vi "MICS Wakeup Calibration Tool JTAG.vi"(8 "error in (no error)":errorcluster, 10 "MICS Dongle Address":refnum<visa-resource-name>="COM8") -> (0 "error out":errorcluster, 2 "Trim Settings":string)   [LabVIEW 2010]
uses:
  <vilib>/Instr/_visa.llb/VISA Configure Serial Port (Instr).vi
panel:
  in  "RSSI Gain":enum16{"1", "3", "10", "30"}(ring)
  in  "WakeupRF":bool
  out "RSSI":u8 format="%02x"
  out "Device Vcc":i32
  in  "DetTrim":bool=TRUE
  in  "Wakeup Signal Transmit":bool
  in  "Samples to Average":u8=5 format="%02d"
  out "Retries":u8 format="%02d"
  out "Loopback Data":u8 format="%02x"
  in  "Loopback Detector":bool
  in  "Update Radio Settings":bool
  in  "Done":bool
  in  "Do RSSI":bool
  out "RSSI Reading":u8(knob) scale=0.0..31.0 scale format="%x"
  in  "Detector Offset Trim":u8(knob)=31 scale=0.0..63.0 scale format="%x"
  in  "Wakeup Signal Power, dBm":dbl(knob)=-32.0 min=-32.25 max=0.0 step=0.25
  in  "RSSI Fine Trim":u8(knob)=16 scale=0.0..31.0 scale format="%x"
  in  "RX Antenna Tune":u8(knob)=7 scale=0.0..15.0 scale format="%x"
  in  "LNA Frequency Trim":u8(knob)=15 scale=0.0..31.0 scale format="%x"
  in  "LNA Gain Trim":u8(knob)=20 scale=0.0..63.0 scale format="%x"
  # "MICS Dongle Address"
  # "All Trims"
  # "Detector Trims Only"
  # "CW RF"
  # "Wakeup Packet"
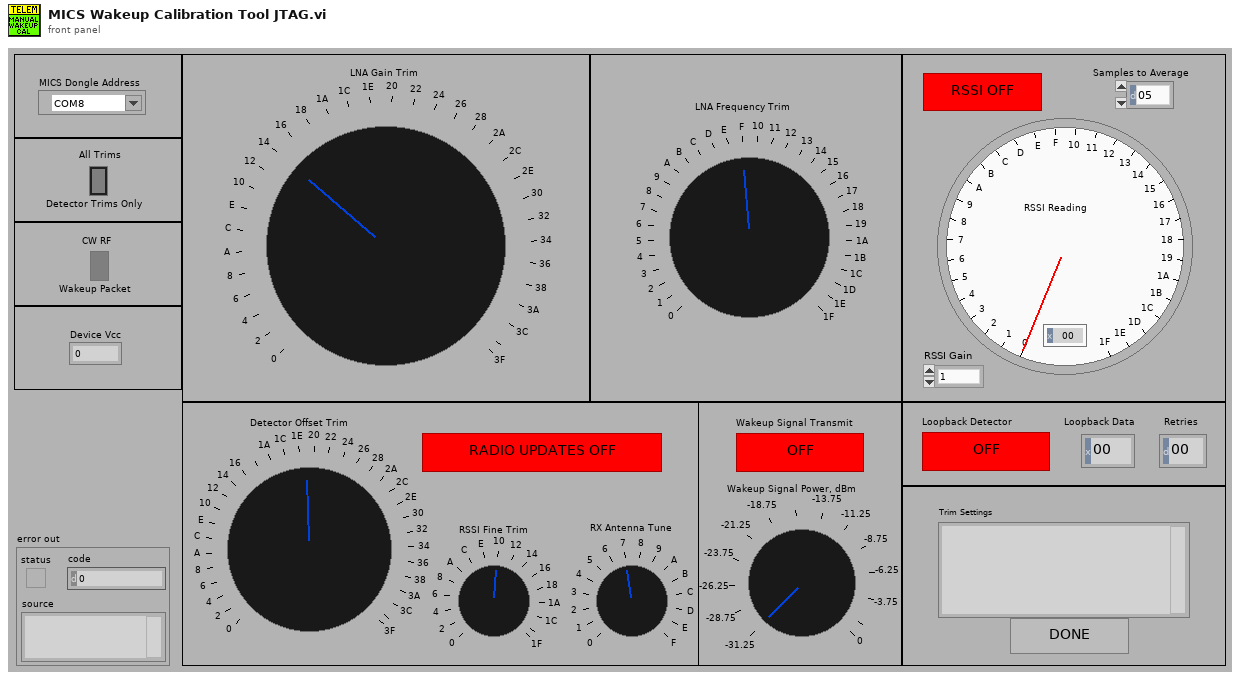
[diagram p1: front panel]
types:
  T1 = cluster{"ConfigFlags":u8, "ImplantID":u32, "CompanyID":u8, "Normal_Comm":cluster{"RF_Channel":u8, "UserData":u8, "TX_Mod":u8, "RX_Mod":u8, "RX_BlockSize":u8, "BlockPerPack":u8, "TX_BlockSize":u8}, "Emerg_Comm":cluster{"RF_Channel":u8, "UserData":u8, "TX_Mod":u8, "RX_Mod":u8, "TX_BlockSize":u8, "BlockPerPack":u8, "RX_BlockSize":u8}, "ImplantRev":u8, "245TX_PowerCal":i8, "245TX_Power":i8, "CCA_RSSI_Thresholds":cluster{"ch0":u16, "ch1":u16, "ch2":u16, "ch3":u16, "ch4":u16, "ch5":u16, "ch6":u16, "ch7":u16, "ch8":u16, "ch9":u16}}
  T2 = enum16{"Start Search", "Continue Search", "End Search"}
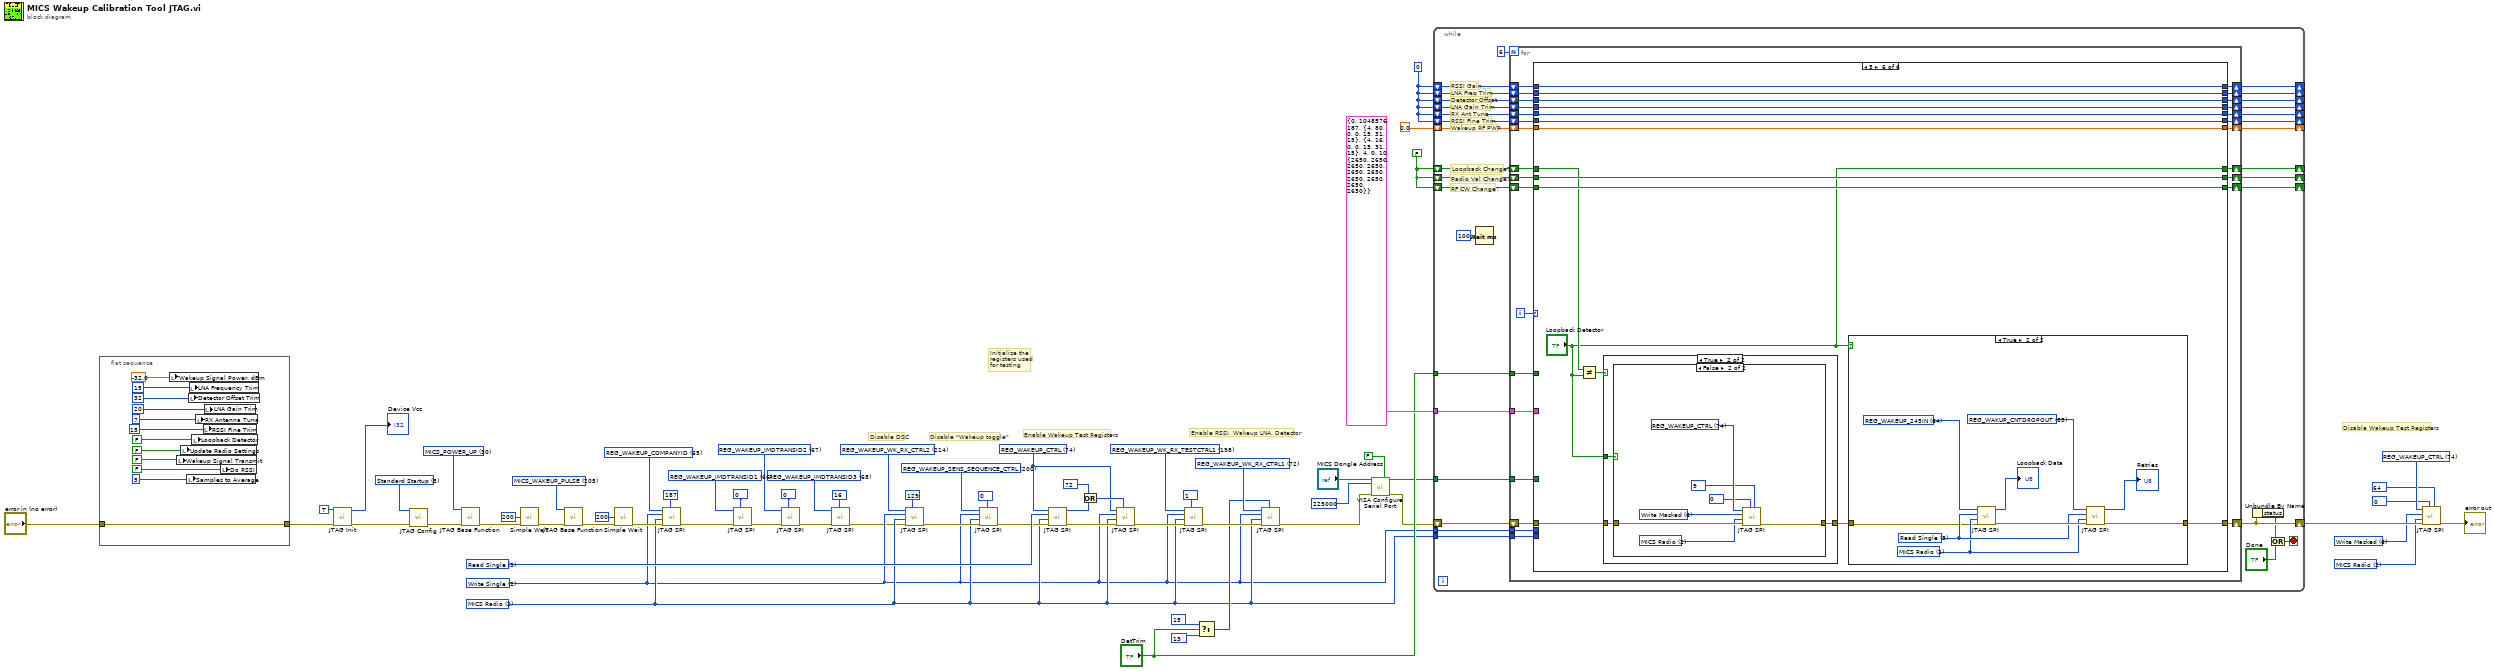
[diagram p0: block diagram]
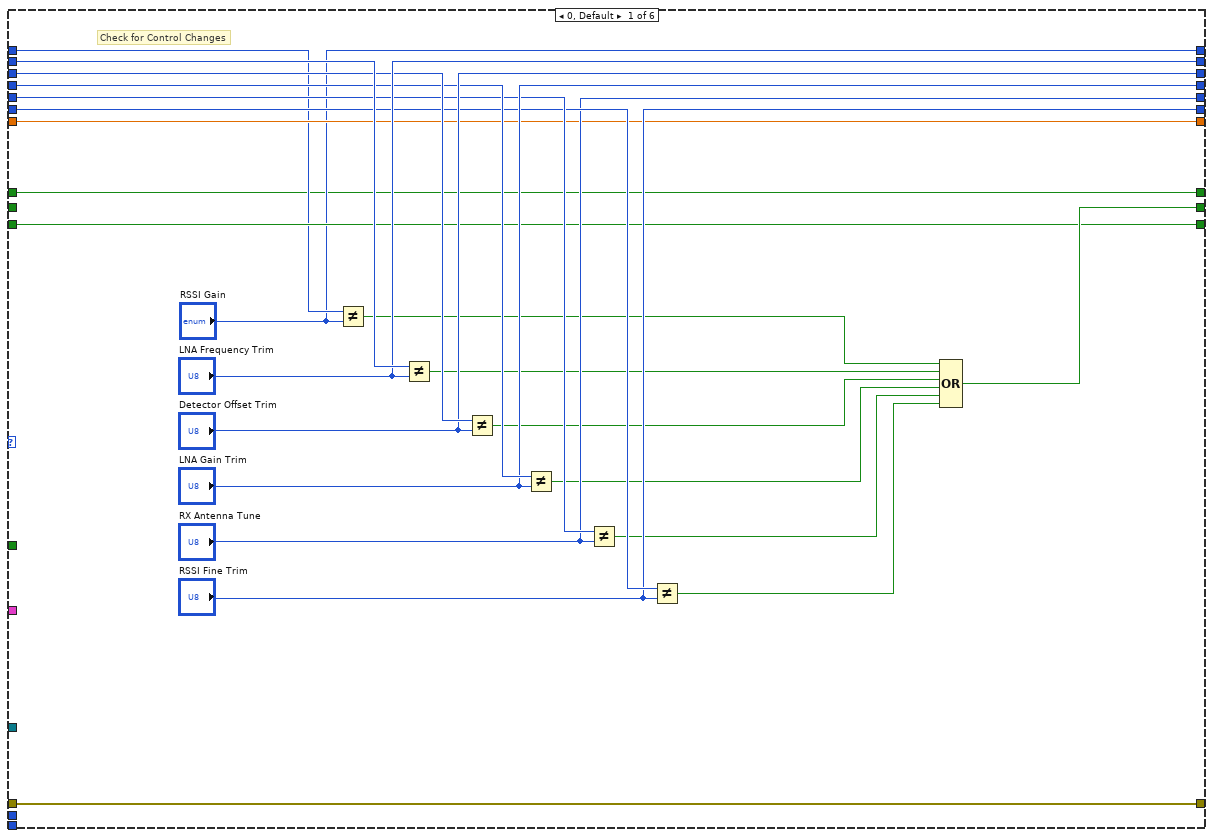
[diagram p2: hidden frame]
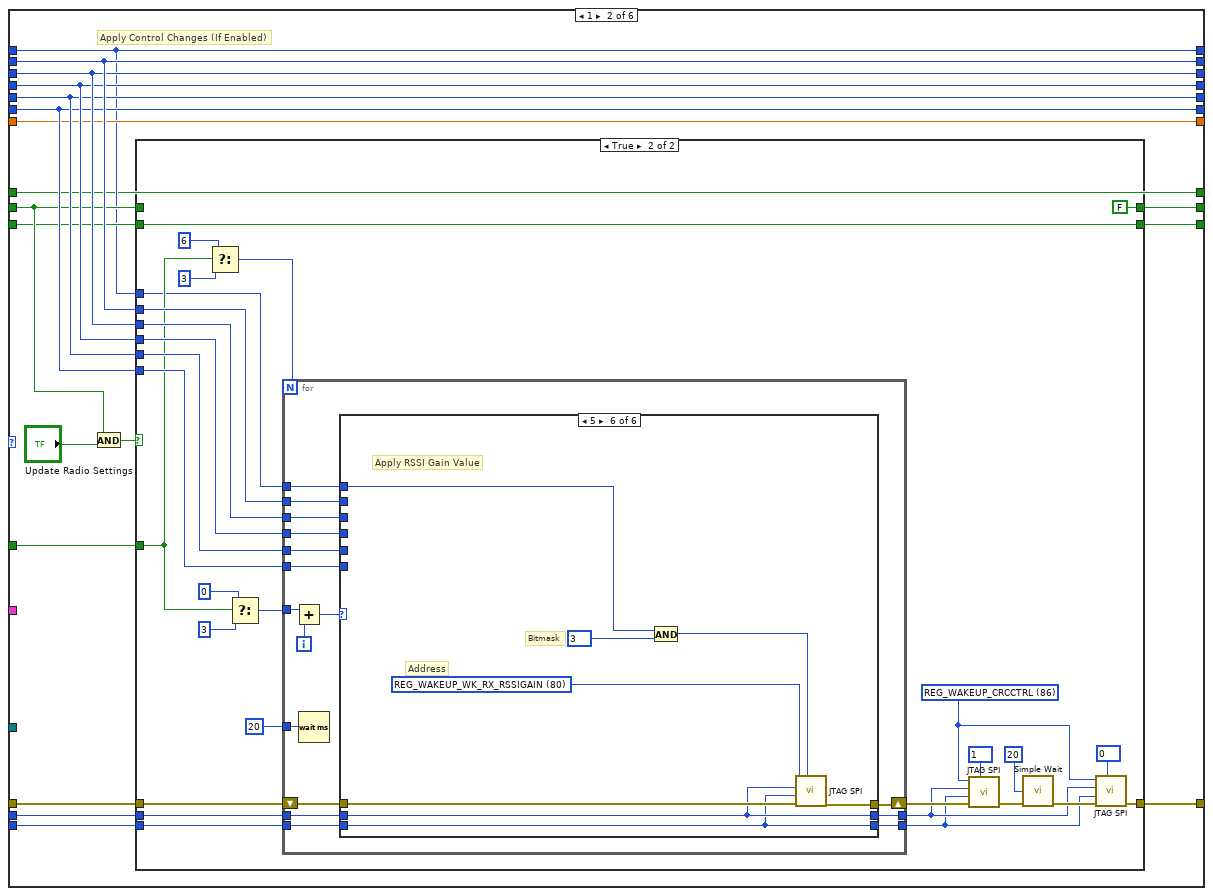
[diagram p3: hidden frame]
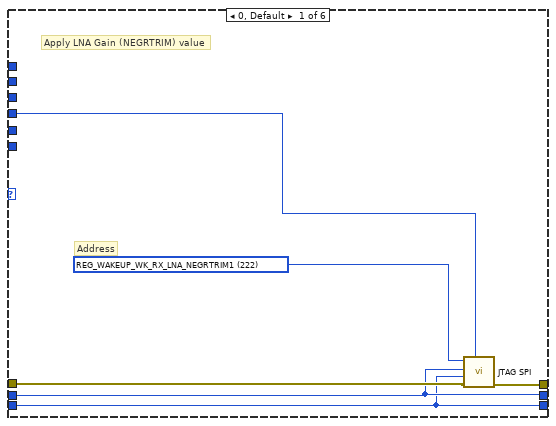
[diagram p5: hidden frame]
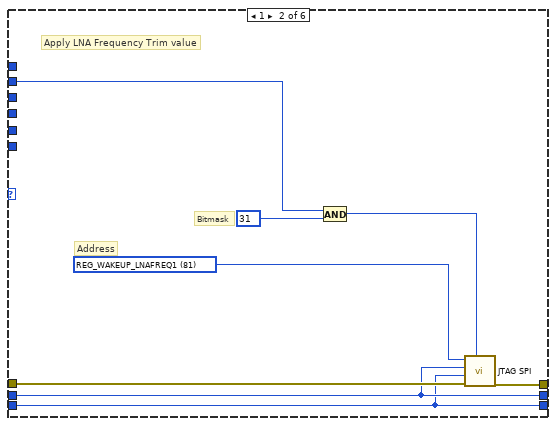
[diagram p6: hidden frame]
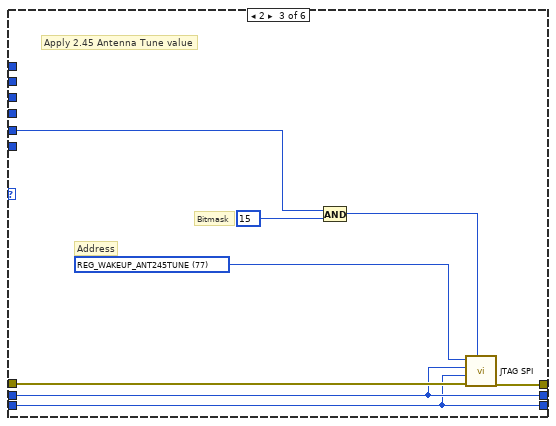
[diagram p7: hidden frame]
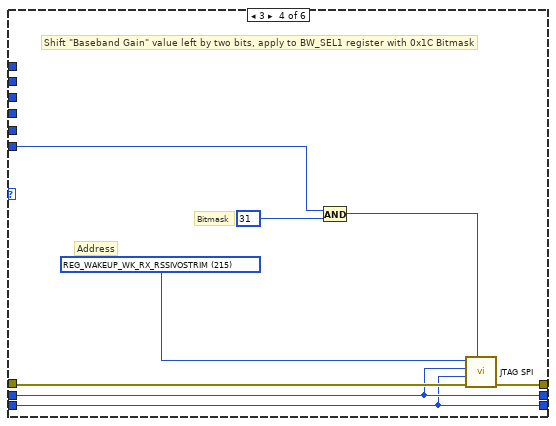
[diagram p8: hidden frame]
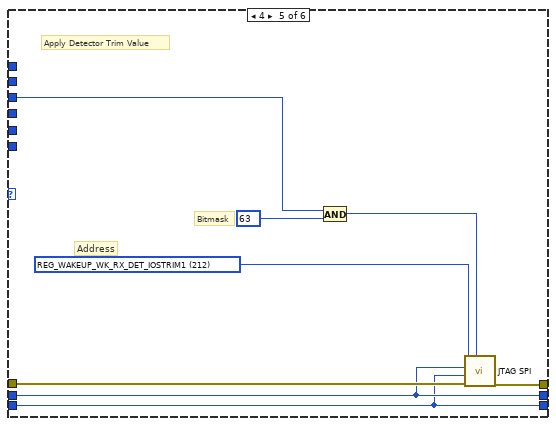
[diagram p9: hidden frame]
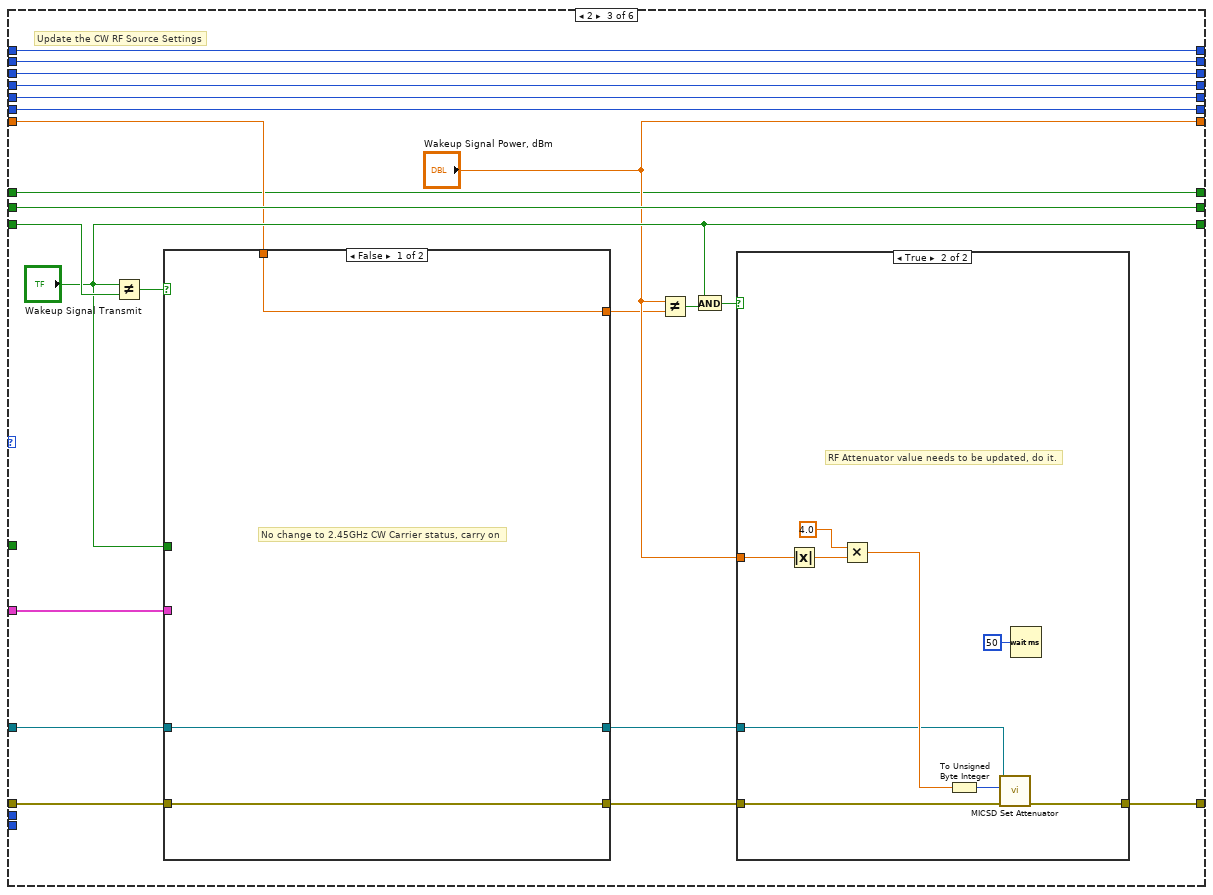
[diagram p10: hidden frame]
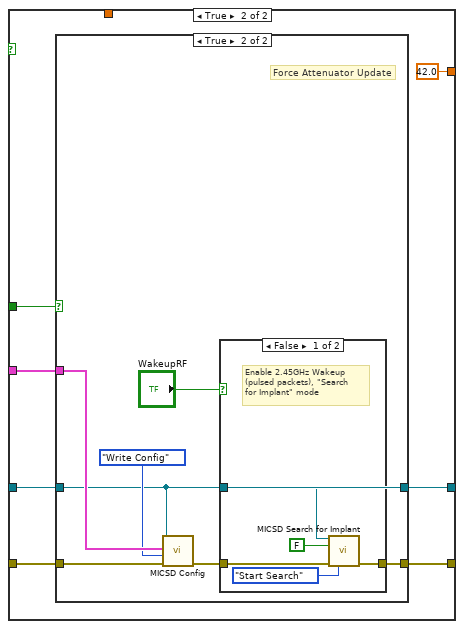
[diagram p12: hidden frame]
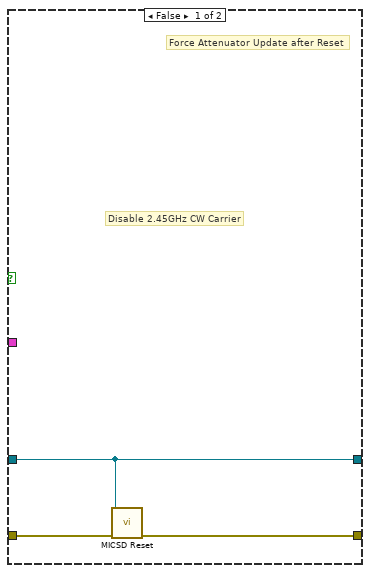
[diagram p13: hidden frame]
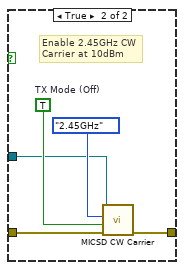
[diagram p14: hidden frame]
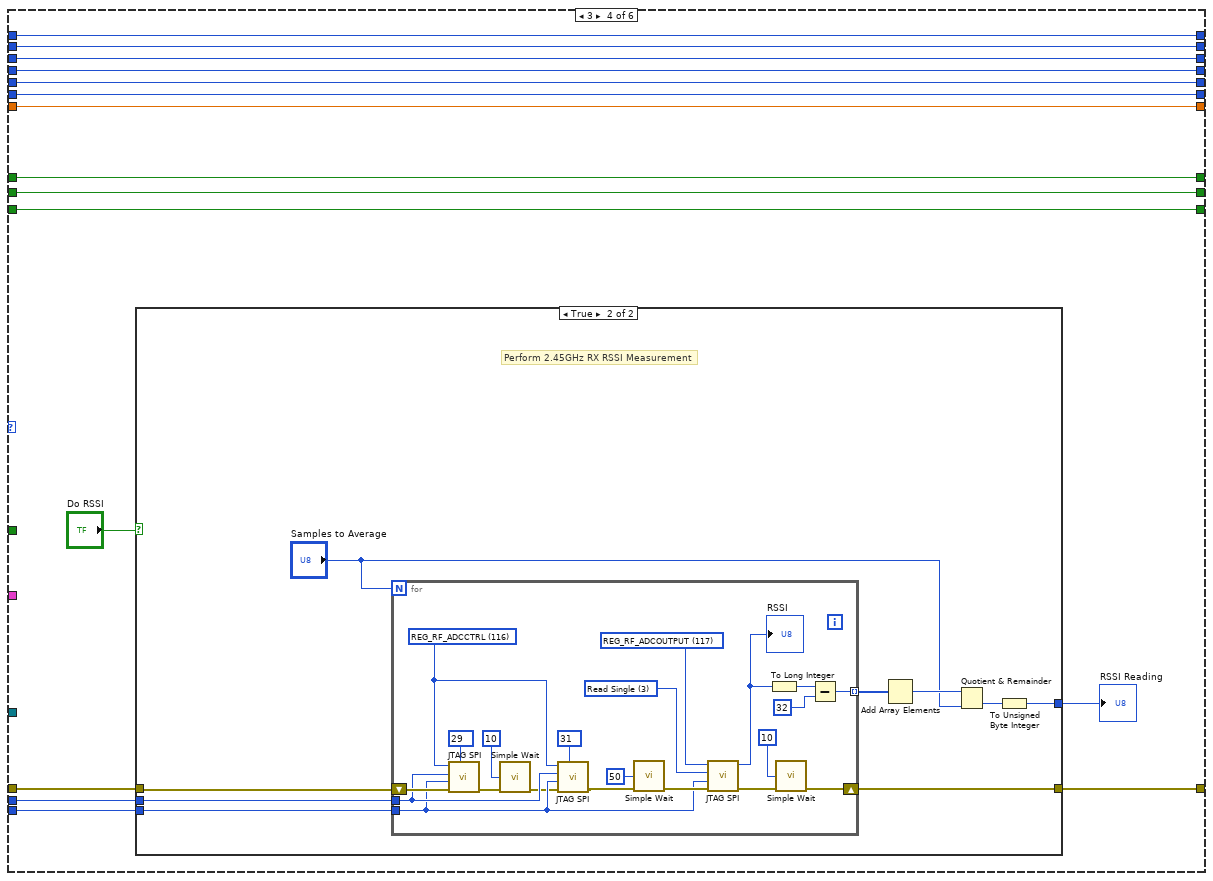
[diagram p15: hidden frame]
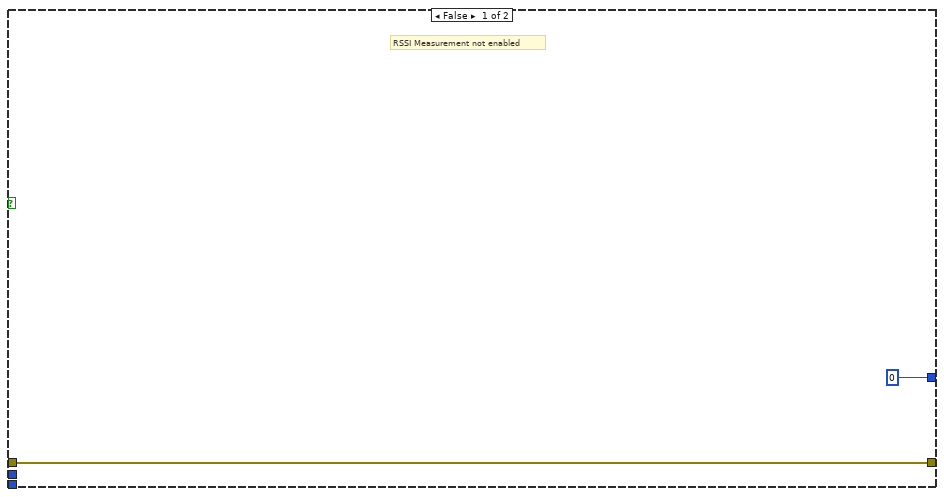
[diagram p16: hidden frame]
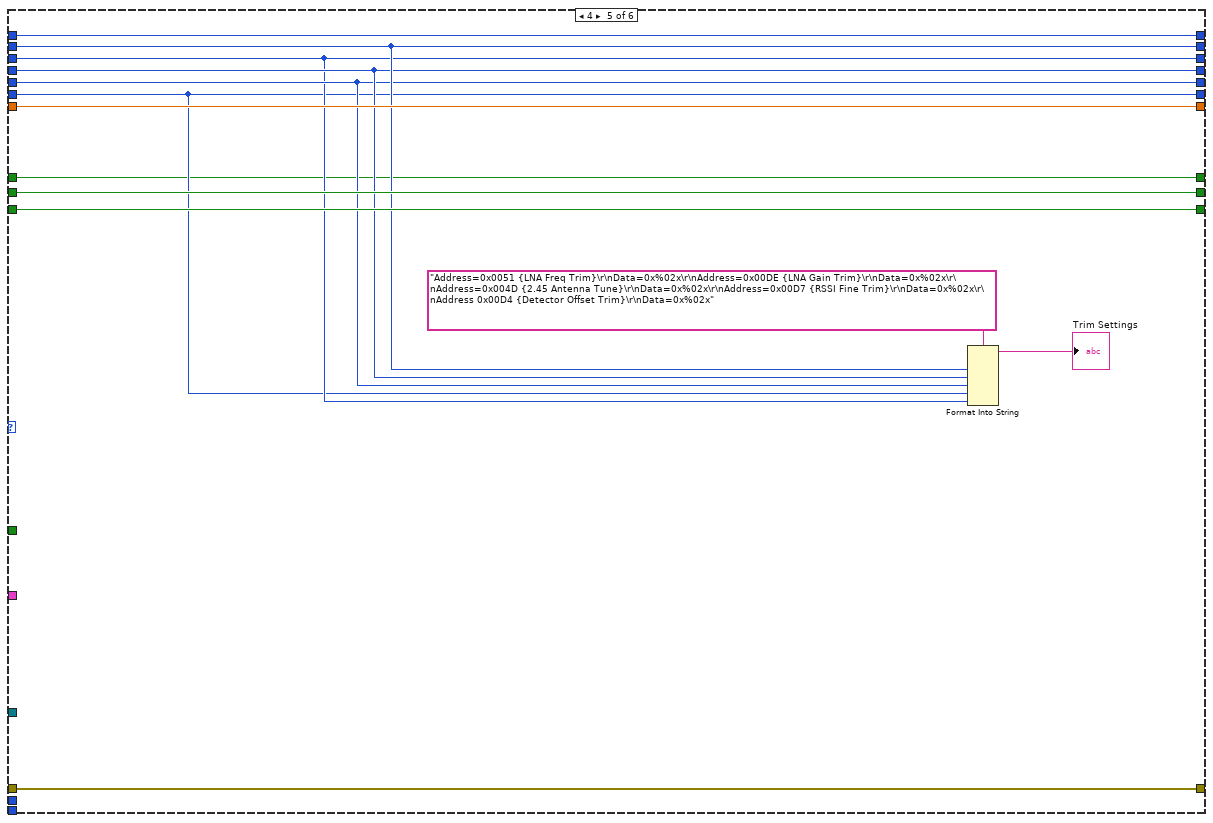
[diagram p17: hidden frame]
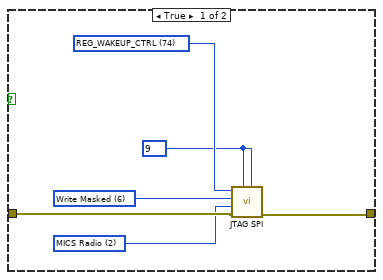
[diagram p19: hidden frame]
diagram:
  w12 = u16 68 items=["---MANUAL ENTRY---"=1000, "REG_NOREG"=0, "REG_RXBUFF_USED"=1, "REG_RXBUFF_BSIZE"=2, "REG_TXBUFF_USED"=3, "REG_TXBUFF_BSIZE"=4, "REG_TXBUFF_MAXPACKSIZE"=5, "REG_MAC_ERRCLR"=6, "REG_MAC_TRAINNUM"=7, "REG_MAC_SYNCMATCH"=8, "REG_MAC_SYNC1"=9, "REG_MAC_SYNC2"=10, "REG_MAC_SYNC3"=11, "REG_MAC_SYNC4"=12, "REG_MAC_SYNC5"=13, "REG_MAC_MAXBERR"=14, "REG_MAC_ECCORR"=15, "REG_MAC_CRCERR"=16, "REG_MAC_BLKCNT1"=17, "REG_MAC_BLKCNT2"=18, "REG_MAC_IMDTRANSID1"=19, "REG_MAC_IMDTRANSID2"=20, "REG_MAC_IMDTRANSID3"=21, "REG_MAC_COMPANYID"=22, "REG_MAC_MODUSER"=23, "REG_MAC_CHANNEL"=25, "REG_MAC_CLEARWDOG"=26, "REG_MAC_CKCORRTHRESH"=27, "REG_HK_TXADDR"=28, "REG_HK_TXDATA"=29, "REG_HK_TXREPLY"=30, "REG_HK_USERDATA"=31, "REG_HK_USERSTATUS"=32, "REG_HK_LASTADDRESS"=33, "REG_HK_MODE"=34, "REG_MAC_STATUSSEQ"=35, "REG_MAC_MAXRETRIES"=36, "REG_MAC_RESENDTIME"=37, "REG_MAC_POWERSAVETIME"=38, "REG_MAC_HEAD_DET"=39, "REG_MAC_CTRL"=41, "REG_MAC_INITCOM"=42, "REG_INTERFACE_MODE"=43, "REG_TXRXBUFF_BOTH"=44, "REG_TXRXBUFF"=45, "REG_IRQ_RAWSTATUS1"=46, "REG_IRQ_ENABLE1"=47, "REG_IRQ_ENABLESET1"=48, "REG_IRQ_ENABLECLEAR1"=49, "REG_IRQ_RAWSTATUS2"=50, "REG_IRQ_ENABLE2"=51, "REG_IRQ_ENABLESET2"=52, "REG_IRQ_ENABLECLEAR2"=53, "REG_IRQ_STATUS1"=54, "REG_IRQ_STATUS2"=55, "REG_IRQ_AUXSTATUS"=56, "REG_TXBUFF_OVERFLOW"=57, "REG_PO0"=58, "REG_P01"=59, "REG_P02"=60, "REG_P03"=61, "REG_GP0"=62, "REG_GPI"=63, "REG_WAKEUP_245IN"=64, "REG_WAKEUP_COMPANYID"=65, "REG_WAKEUP_IMDTRANSID1"=66, "REG_WAKEUP_IMDTRANSID2"=67, "REG_WAKEUP_IMDTRANSID3"=68, "REG_WAKEUP_CHANNEL"=69, "REG_WAKEUP_MODUSER"=70, "REG_WAKEUP_DEVICEMODE"=71, "REG_WAKEUP_WK_RX_CTRL1"=72, "REG_WAKEUP_STACK_ADDR"=73, "REG_WAKEUP_CTRL"=74, "REG_WAKEUP_STROSCRTRIM"=75, "REG_WAKEUP_BIASTRIM"=76, "REG_WAKEUP_ANT245TUNE"=77, "REG_WAKEUP_WK_RX_RTRIMDET"=78, "REG_WAKEUP_WK_RX_RTRIMDEMOD"=79, "REG_WAKEUP_WK_RX_RSSIGAIN"=80, "REG_WAKEUP_LNAFREQ1"=81, "REG_WAKEUP_STACK"=83, "REG_WAKUP_XOSU"=84, "REG_WAKUP_CNTDROPOUT"=85, "REG_WAKEUP_CRCCTRL"=86, "REG_WAKEUP_CRCWORD1"=87, "REG_WAKEUP_CRCWORD2"=88, "REG_WAKEUP_WK_RX_CTRIM"=89, "REG_WAKEUP_VDDATRIM"=90, "REG_WAKEUP_VDDDTRIM"=91, "REG_WAKEUP_TESTIOBUFEN"=92, "REG_WAKEUP_TESTIOCLAMP"=93, "CORE_RESET_ADDRESS"=94, "CHIP_RESET_ADDRESS"=95, "REG_RF_TXGENCTRL"=96, "REG_RF_TXIFCTRL"=97, "REG_RF_TXRF_SEL_CTRL"=98, "REG_RF_TXRFPWRDEFAULTSET"=99, "REG_RF_RSSITRIM"=100, "REG_RF_TXIFOSCTUNE"=101, "REG_RF_TXIFGAINIMB"=102, "REG_RF_TXIFLOCK"=103, "REG_RF_RXRFLNAGAINTRIM"=104, "REG_RF_RXBIASTR"=105, "REG_RF_RXGENCTRL"=106, "REG_RF_RXIFADCDECLEV"=107, "REG_RF_RXIFDETFILTERTUNE"=108, "REG_RF_RXIFFILTERTUNE"=109, "REG_RF_GENENABLES"=110, "REG_RF_SYNTH_CHANNEL"=111, "REG_TX_RAMP_RTRIM"=112, "REG_TX_RAMP_CTRIM"=113, "REG_RF_XO_TRIM"=114, "REG_RF_SYNTH_SET_TRIM"=115, "REG_RF_ADCCTRL"=116, "REG_RF_ADCOUTPUT"=117, "REG_RF_TXIFAMP"=118, "REG_RF_SYNTH_RTRIM"=119, "REG_RF_SYNTH_CTRIM"=120, "REG_RF_SYNTH_CT"=121, "REG_RF_TXMIXER_IOSTRIM_HIGH_IP"=122, "REG_RF_TXMIXER_IOSTRIM_HIGH_IN"=123, "REG_RF_TXMIXER_IOSTRIM_HIGH_QP"=124, "REG_RF_TXMIXER_IOSTRIM_HIGH_QN"=125, "REG_HX_WUADDR"=126, "REG_REVISION"=127, "REG_NOREG_TEST"=128, "REG_DTEST_RXBUFF"=129, "REG_RXBUFF_NEXT_BLOCK"=130, "REG_RXBUFF_FIRST_IN_PACK"=131, "REG_RXBUFF_FIRST_EMPTY"=132, "REG_MAC_BYPASS"=133, "REG_DTEST_TXBUFF"=134, "REG_TXBUFF_NEXT_BLOCK"=135, "REG_TXBUFF_FIRST_IN_PACK"=136, "REG_TXBUFF_FIRST_EMPTY"=137, "REG_DTEST_SEQ"=138, "REG_DTEST_CKCORR"=139, "REG_MAC_TOPSTATE"=140, "REG_DTEST_INTERFACE"=141, "REG_IFACE_TXRX_BYPASS"=142, "REG_MAC_TXRXWAIT"=143, "REG_MAC_TXRFRAMP"=144, "REG_MAC_TRAINWORD"=145, "REG_MAC_TRAINWORD2"=146, "REG_MAC_SETTINGS"=147, "REG_MAC_CALSELECT1"=148, "REG_MAC_CALSELECT2"=149, "REG_MAC_ANTMATCHSEL"=150, "REG_MAC_ANTTUNESEL1"=151, "REG_MAC_ANTTUNESEL2"=152, "REG_MAC_ANTTUNESEL3"=153, "REG_MAC_ANTTUNESTEP"=154, "REG_MAC_WUMODEBURST"=156, "REG_MAC_WUOFFSHORT"=157, "REG_MAC_WUOFFLONG"=158, "REG_MAC_CLKRECCTRL"=159, "REG_HK_MODE_P2"=162, "REG_MAC_ANTTUNERES1"=164, "REG_MAC_ANTTUNERES2"=165, "REG_INTERFACE_MODE_TEST"=171, "REG_TXRXBUFF_BOTH_P2"=172, "REG_TXRXBUFF_P2"=173, "REG_IRQ_RAWSTATUS1_P2"=174, "REG_MAC_TXIFSTATUS1"=176, "REG_MAC_TXIFSTATUS2"=177, "REG_IRQ_RAWSTATUS2_P2"=178, "REG_MAC_TXIFRAMPDELAY"=179, "REG_MAC_TXIFRAMPSLOPE"=180, "REG_MAX_TXIFRAMP"=181, "REG_IRQ_STATUS1_P2"=182, "REG_IRQ_STATUS2_P2"=183, "REG_IRQ_AUXSTATUS_P2"=184, "REG_MAC_UNLOCK"=188, "REG_MAC_TXIFFREQ"=190, "REG_WAKEUP_TESTCTRL1"=192, "REG_WAKEUP_RX_EN_CNT"=193, "REG_WAKEUP_TESTENABLES"=194, "REG_WAKEUP_DTBI_CTRL"=195, "REG_WAKEUP_DTBO_CTRL"=196, "REG_WAKEUP_TESTIOBUFTEST"=197, "REG_WAKEUP_WK_RX_TESTCTRL1"=198, "REG_WAKEUP_WK_RX_TESTCTRL2"=199, "REG_WAKEUP_SENS_SEQUENCE_CTRL"=200, "REG_WAKEUP_LNABIAS"=201, "REG_WAKEUP_DET_TH_TRIM1"=202, "REG_WAKEUP_LNABIAS_NOM1"=203, "REG_WAKEUP_RX_TSHORT_TRIM1"=204, "REG_WAKEUP_LNABIAS_NOM2"=205, "REG_WAKEUP_RX_TLONG_TRIM1"=206, "REG_WAKEUP_LNA_NEGRTRIM_NOM1"=207, "REG_WAKEUP_RX_TBURST_TRIM1"=208, "REG_WAKEUP_RX_LNA_NEGRTRIM_NOM2"=209, "REG_WAKEUP_RX_BB_G_BW_SEL1"=210, "REG_WAKEUP_WK_RX_DET_IOSTRIM1"=212, "REG_WAKEUP_WK_RX_CTRL2"=214, "REG_WAKEUP_WK_RX_RSSIVOSTRIM"=215, "REG_WAKEUP_LNANEGR_EFF"=216, "REG_WAKEUP_XOSU_FAST"=217, "REG_WAKEUP_STROSCPWIDTH1"=218, "REG_WAKEUP_STROSCPERIOD1"=220, "REG_WAKEUP_STROSCPERIOD2"=221, "REG_WAKEUP_WK_RX_LNA_NEGRTRIM1"=222, "REG_RF_TXTESTENABLE"=224, "REG_RF_TXIFTESTMODE"=225, "REG_RF_RXTESTENABLE"=226, "REG_RF_RXIFTESTCTRL1"=227, "REG_RF_RXIFTESTCTRL2"=228, "REG_RF_RXIFTESTCTRL3"=229, "REG_RF_SYNTH_TESTCTRL1"=230, "REG_RF_SYNTH_TESTCTRL2"=231, "REG_RF_SYNTH_TESTCTRL3"=232, "REG_RF_ADCTEST1"=237, "REG_RF_ADCTEST2"=238, "REG_RF_TXMIXER_IOSTRIM_LOW_IP"=240, "REG_RF_TXMIXER_IOSTRIM_LOW_IN"=241, "REG_RF_TXMIXER_ISOTRIM_LOW_QP"=242, "REG_RF_TXMIXER_IOSTRIM_LOW_QN"=243, "REG_RF_SYNTH_KPD"=244, "REG_RF_SYNTH_LOLEV"=245, "REG_RF_TXRFPWRTUNEANTSET"=246, "REG_RF_TXPD_GAIN_CTRL"=247, "REG_RF_SYNTH_STARTUP"=248, "REG_RF_TXRFANTTUNE_TXMODE"=249, "REG_RF_TXRFANTTUNE_RXMODE"=250, "REG_RF_RXRFANTTUNE_TXMODE"=251, "REG_RF_RXRFANTTUNE_RXMODE"=252, "REG_ANTMATCH1"=253, "REG_ANTMATCH2"=254, "REG_REVISION_P2"=255] ("Register")
  w14 = u16 67 items=["---MANUAL ENTRY---"=1000, "REG_NOREG"=0, "REG_RXBUFF_USED"=1, "REG_RXBUFF_BSIZE"=2, "REG_TXBUFF_USED"=3, "REG_TXBUFF_BSIZE"=4, "REG_TXBUFF_MAXPACKSIZE"=5, "REG_MAC_ERRCLR"=6, "REG_MAC_TRAINNUM"=7, "REG_MAC_SYNCMATCH"=8, "REG_MAC_SYNC1"=9, "REG_MAC_SYNC2"=10, "REG_MAC_SYNC3"=11, "REG_MAC_SYNC4"=12, "REG_MAC_SYNC5"=13, "REG_MAC_MAXBERR"=14, "REG_MAC_ECCORR"=15, "REG_MAC_CRCERR"=16, "REG_MAC_BLKCNT1"=17, "REG_MAC_BLKCNT2"=18, "REG_MAC_IMDTRANSID1"=19, "REG_MAC_IMDTRANSID2"=20, "REG_MAC_IMDTRANSID3"=21, "REG_MAC_COMPANYID"=22, "REG_MAC_MODUSER"=23, "REG_MAC_CHANNEL"=25, "REG_MAC_CLEARWDOG"=26, "REG_MAC_CKCORRTHRESH"=27, "REG_HK_TXADDR"=28, "REG_HK_TXDATA"=29, "REG_HK_TXREPLY"=30, "REG_HK_USERDATA"=31, "REG_HK_USERSTATUS"=32, "REG_HK_LASTADDRESS"=33, "REG_HK_MODE"=34, "REG_MAC_STATUSSEQ"=35, "REG_MAC_MAXRETRIES"=36, "REG_MAC_RESENDTIME"=37, "REG_MAC_POWERSAVETIME"=38, "REG_MAC_HEAD_DET"=39, "REG_MAC_CTRL"=41, "REG_MAC_INITCOM"=42, "REG_INTERFACE_MODE"=43, "REG_TXRXBUFF_BOTH"=44, "REG_TXRXBUFF"=45, "REG_IRQ_RAWSTATUS1"=46, "REG_IRQ_ENABLE1"=47, "REG_IRQ_ENABLESET1"=48, "REG_IRQ_ENABLECLEAR1"=49, "REG_IRQ_RAWSTATUS2"=50, "REG_IRQ_ENABLE2"=51, "REG_IRQ_ENABLESET2"=52, "REG_IRQ_ENABLECLEAR2"=53, "REG_IRQ_STATUS1"=54, "REG_IRQ_STATUS2"=55, "REG_IRQ_AUXSTATUS"=56, "REG_TXBUFF_OVERFLOW"=57, "REG_PO0"=58, "REG_P01"=59, "REG_P02"=60, "REG_P03"=61, "REG_GP0"=62, "REG_GPI"=63, "REG_WAKEUP_245IN"=64, "REG_WAKEUP_COMPANYID"=65, "REG_WAKEUP_IMDTRANSID1"=66, "REG_WAKEUP_IMDTRANSID2"=67, "REG_WAKEUP_IMDTRANSID3"=68, "REG_WAKEUP_CHANNEL"=69, "REG_WAKEUP_MODUSER"=70, "REG_WAKEUP_DEVICEMODE"=71, "REG_WAKEUP_WK_RX_CTRL1"=72, "REG_WAKEUP_STACK_ADDR"=73, "REG_WAKEUP_CTRL"=74, "REG_WAKEUP_STROSCRTRIM"=75, "REG_WAKEUP_BIASTRIM"=76, "REG_WAKEUP_ANT245TUNE"=77, "REG_WAKEUP_WK_RX_RTRIMDET"=78, "REG_WAKEUP_WK_RX_RTRIMDEMOD"=79, "REG_WAKEUP_WK_RX_RSSIGAIN"=80, "REG_WAKEUP_LNAFREQ1"=81, "REG_WAKEUP_STACK"=83, "REG_WAKUP_XOSU"=84, "REG_WAKUP_CNTDROPOUT"=85, "REG_WAKEUP_CRCCTRL"=86, "REG_WAKEUP_CRCWORD1"=87, "REG_WAKEUP_CRCWORD2"=88, "REG_WAKEUP_WK_RX_CTRIM"=89, "REG_WAKEUP_VDDATRIM"=90, "REG_WAKEUP_VDDDTRIM"=91, "REG_WAKEUP_TESTIOBUFEN"=92, "REG_WAKEUP_TESTIOCLAMP"=93, "CORE_RESET_ADDRESS"=94, "CHIP_RESET_ADDRESS"=95, "REG_RF_TXGENCTRL"=96, "REG_RF_TXIFCTRL"=97, "REG_RF_TXRF_SEL_CTRL"=98, "REG_RF_TXRFPWRDEFAULTSET"=99, "REG_RF_RSSITRIM"=100, "REG_RF_TXIFOSCTUNE"=101, "REG_RF_TXIFGAINIMB"=102, "REG_RF_TXIFLOCK"=103, "REG_RF_RXRFLNAGAINTRIM"=104, "REG_RF_RXBIASTR"=105, "REG_RF_RXGENCTRL"=106, "REG_RF_RXIFADCDECLEV"=107, "REG_RF_RXIFDETFILTERTUNE"=108, "REG_RF_RXIFFILTERTUNE"=109, "REG_RF_GENENABLES"=110, "REG_RF_SYNTH_CHANNEL"=111, "REG_TX_RAMP_RTRIM"=112, "REG_TX_RAMP_CTRIM"=113, "REG_RF_XO_TRIM"=114, "REG_RF_SYNTH_SET_TRIM"=115, "REG_RF_ADCCTRL"=116, "REG_RF_ADCOUTPUT"=117, "REG_RF_TXIFAMP"=118, "REG_RF_SYNTH_RTRIM"=119, "REG_RF_SYNTH_CTRIM"=120, "REG_RF_SYNTH_CT"=121, "REG_RF_TXMIXER_IOSTRIM_HIGH_IP"=122, "REG_RF_TXMIXER_IOSTRIM_HIGH_IN"=123, "REG_RF_TXMIXER_IOSTRIM_HIGH_QP"=124, "REG_RF_TXMIXER_IOSTRIM_HIGH_QN"=125, "REG_HX_WUADDR"=126, "REG_REVISION"=127, "REG_NOREG_TEST"=128, "REG_DTEST_RXBUFF"=129, "REG_RXBUFF_NEXT_BLOCK"=130, "REG_RXBUFF_FIRST_IN_PACK"=131, "REG_RXBUFF_FIRST_EMPTY"=132, "REG_MAC_BYPASS"=133, "REG_DTEST_TXBUFF"=134, "REG_TXBUFF_NEXT_BLOCK"=135, "REG_TXBUFF_FIRST_IN_PACK"=136, "REG_TXBUFF_FIRST_EMPTY"=137, "REG_DTEST_SEQ"=138, "REG_DTEST_CKCORR"=139, "REG_MAC_TOPSTATE"=140, "REG_DTEST_INTERFACE"=141, "REG_IFACE_TXRX_BYPASS"=142, "REG_MAC_TXRXWAIT"=143, "REG_MAC_TXRFRAMP"=144, "REG_MAC_TRAINWORD"=145, "REG_MAC_TRAINWORD2"=146, "REG_MAC_SETTINGS"=147, "REG_MAC_CALSELECT1"=148, "REG_MAC_CALSELECT2"=149, "REG_MAC_ANTMATCHSEL"=150, "REG_MAC_ANTTUNESEL1"=151, "REG_MAC_ANTTUNESEL2"=152, "REG_MAC_ANTTUNESEL3"=153, "REG_MAC_ANTTUNESTEP"=154, "REG_MAC_WUMODEBURST"=156, "REG_MAC_WUOFFSHORT"=157, "REG_MAC_WUOFFLONG"=158, "REG_MAC_CLKRECCTRL"=159, "REG_HK_MODE_P2"=162, "REG_MAC_ANTTUNERES1"=164, "REG_MAC_ANTTUNERES2"=165, "REG_INTERFACE_MODE_TEST"=171, "REG_TXRXBUFF_BOTH_P2"=172, "REG_TXRXBUFF_P2"=173, "REG_IRQ_RAWSTATUS1_P2"=174, "REG_MAC_TXIFSTATUS1"=176, "REG_MAC_TXIFSTATUS2"=177, "REG_IRQ_RAWSTATUS2_P2"=178, "REG_MAC_TXIFRAMPDELAY"=179, "REG_MAC_TXIFRAMPSLOPE"=180, "REG_MAX_TXIFRAMP"=181, "REG_IRQ_STATUS1_P2"=182, "REG_IRQ_STATUS2_P2"=183, "REG_IRQ_AUXSTATUS_P2"=184, "REG_MAC_UNLOCK"=188, "REG_MAC_TXIFFREQ"=190, "REG_WAKEUP_TESTCTRL1"=192, "REG_WAKEUP_RX_EN_CNT"=193, "REG_WAKEUP_TESTENABLES"=194, "REG_WAKEUP_DTBI_CTRL"=195, "REG_WAKEUP_DTBO_CTRL"=196, "REG_WAKEUP_TESTIOBUFTEST"=197, "REG_WAKEUP_WK_RX_TESTCTRL1"=198, "REG_WAKEUP_WK_RX_TESTCTRL2"=199, "REG_WAKEUP_SENS_SEQUENCE_CTRL"=200, "REG_WAKEUP_LNABIAS"=201, "REG_WAKEUP_DET_TH_TRIM1"=202, "REG_WAKEUP_LNABIAS_NOM1"=203, "REG_WAKEUP_RX_TSHORT_TRIM1"=204, "REG_WAKEUP_LNABIAS_NOM2"=205, "REG_WAKEUP_RX_TLONG_TRIM1"=206, "REG_WAKEUP_LNA_NEGRTRIM_NOM1"=207, "REG_WAKEUP_RX_TBURST_TRIM1"=208, "REG_WAKEUP_RX_LNA_NEGRTRIM_NOM2"=209, "REG_WAKEUP_RX_BB_G_BW_SEL1"=210, "REG_WAKEUP_WK_RX_DET_IOSTRIM1"=212, "REG_WAKEUP_WK_RX_CTRL2"=214, "REG_WAKEUP_WK_RX_RSSIVOSTRIM"=215, "REG_WAKEUP_LNANEGR_EFF"=216, "REG_WAKEUP_XOSU_FAST"=217, "REG_WAKEUP_STROSCPWIDTH1"=218, "REG_WAKEUP_STROSCPERIOD1"=220, "REG_WAKEUP_STROSCPERIOD2"=221, "REG_WAKEUP_WK_RX_LNA_NEGRTRIM1"=222, "REG_RF_TXTESTENABLE"=224, "REG_RF_TXIFTESTMODE"=225, "REG_RF_RXTESTENABLE"=226, "REG_RF_RXIFTESTCTRL1"=227, "REG_RF_RXIFTESTCTRL2"=228, "REG_RF_RXIFTESTCTRL3"=229, "REG_RF_SYNTH_TESTCTRL1"=230, "REG_RF_SYNTH_TESTCTRL2"=231, "REG_RF_SYNTH_TESTCTRL3"=232, "REG_RF_ADCTEST1"=237, "REG_RF_ADCTEST2"=238, "REG_RF_TXMIXER_IOSTRIM_LOW_IP"=240, "REG_RF_TXMIXER_IOSTRIM_LOW_IN"=241, "REG_RF_TXMIXER_ISOTRIM_LOW_QP"=242, "REG_RF_TXMIXER_IOSTRIM_LOW_QN"=243, "REG_RF_SYNTH_KPD"=244, "REG_RF_SYNTH_LOLEV"=245, "REG_RF_TXRFPWRTUNEANTSET"=246, "REG_RF_TXPD_GAIN_CTRL"=247, "REG_RF_SYNTH_STARTUP"=248, "REG_RF_TXRFANTTUNE_TXMODE"=249, "REG_RF_TXRFANTTUNE_RXMODE"=250, "REG_RF_RXRFANTTUNE_TXMODE"=251, "REG_RF_RXRFANTTUNE_RXMODE"=252, "REG_ANTMATCH1"=253, "REG_ANTMATCH2"=254, "REG_REVISION_P2"=255] ("Register")
  w16 = u16 66 items=["---MANUAL ENTRY---"=1000, "REG_NOREG"=0, "REG_RXBUFF_USED"=1, "REG_RXBUFF_BSIZE"=2, "REG_TXBUFF_USED"=3, "REG_TXBUFF_BSIZE"=4, "REG_TXBUFF_MAXPACKSIZE"=5, "REG_MAC_ERRCLR"=6, "REG_MAC_TRAINNUM"=7, "REG_MAC_SYNCMATCH"=8, "REG_MAC_SYNC1"=9, "REG_MAC_SYNC2"=10, "REG_MAC_SYNC3"=11, "REG_MAC_SYNC4"=12, "REG_MAC_SYNC5"=13, "REG_MAC_MAXBERR"=14, "REG_MAC_ECCORR"=15, "REG_MAC_CRCERR"=16, "REG_MAC_BLKCNT1"=17, "REG_MAC_BLKCNT2"=18, "REG_MAC_IMDTRANSID1"=19, "REG_MAC_IMDTRANSID2"=20, "REG_MAC_IMDTRANSID3"=21, "REG_MAC_COMPANYID"=22, "REG_MAC_MODUSER"=23, "REG_MAC_CHANNEL"=25, "REG_MAC_CLEARWDOG"=26, "REG_MAC_CKCORRTHRESH"=27, "REG_HK_TXADDR"=28, "REG_HK_TXDATA"=29, "REG_HK_TXREPLY"=30, "REG_HK_USERDATA"=31, "REG_HK_USERSTATUS"=32, "REG_HK_LASTADDRESS"=33, "REG_HK_MODE"=34, "REG_MAC_STATUSSEQ"=35, "REG_MAC_MAXRETRIES"=36, "REG_MAC_RESENDTIME"=37, "REG_MAC_POWERSAVETIME"=38, "REG_MAC_HEAD_DET"=39, "REG_MAC_CTRL"=41, "REG_MAC_INITCOM"=42, "REG_INTERFACE_MODE"=43, "REG_TXRXBUFF_BOTH"=44, "REG_TXRXBUFF"=45, "REG_IRQ_RAWSTATUS1"=46, "REG_IRQ_ENABLE1"=47, "REG_IRQ_ENABLESET1"=48, "REG_IRQ_ENABLECLEAR1"=49, "REG_IRQ_RAWSTATUS2"=50, "REG_IRQ_ENABLE2"=51, "REG_IRQ_ENABLESET2"=52, "REG_IRQ_ENABLECLEAR2"=53, "REG_IRQ_STATUS1"=54, "REG_IRQ_STATUS2"=55, "REG_IRQ_AUXSTATUS"=56, "REG_TXBUFF_OVERFLOW"=57, "REG_PO0"=58, "REG_P01"=59, "REG_P02"=60, "REG_P03"=61, "REG_GP0"=62, "REG_GPI"=63, "REG_WAKEUP_245IN"=64, "REG_WAKEUP_COMPANYID"=65, "REG_WAKEUP_IMDTRANSID1"=66, "REG_WAKEUP_IMDTRANSID2"=67, "REG_WAKEUP_IMDTRANSID3"=68, "REG_WAKEUP_CHANNEL"=69, "REG_WAKEUP_MODUSER"=70, "REG_WAKEUP_DEVICEMODE"=71, "REG_WAKEUP_WK_RX_CTRL1"=72, "REG_WAKEUP_STACK_ADDR"=73, "REG_WAKEUP_CTRL"=74, "REG_WAKEUP_STROSCRTRIM"=75, "REG_WAKEUP_BIASTRIM"=76, "REG_WAKEUP_ANT245TUNE"=77, "REG_WAKEUP_WK_RX_RTRIMDET"=78, "REG_WAKEUP_WK_RX_RTRIMDEMOD"=79, "REG_WAKEUP_WK_RX_RSSIGAIN"=80, "REG_WAKEUP_LNAFREQ1"=81, "REG_WAKEUP_STACK"=83, "REG_WAKUP_XOSU"=84, "REG_WAKUP_CNTDROPOUT"=85, "REG_WAKEUP_CRCCTRL"=86, "REG_WAKEUP_CRCWORD1"=87, "REG_WAKEUP_CRCWORD2"=88, "REG_WAKEUP_WK_RX_CTRIM"=89, "REG_WAKEUP_VDDATRIM"=90, "REG_WAKEUP_VDDDTRIM"=91, "REG_WAKEUP_TESTIOBUFEN"=92, "REG_WAKEUP_TESTIOCLAMP"=93, "CORE_RESET_ADDRESS"=94, "CHIP_RESET_ADDRESS"=95, "REG_RF_TXGENCTRL"=96, "REG_RF_TXIFCTRL"=97, "REG_RF_TXRF_SEL_CTRL"=98, "REG_RF_TXRFPWRDEFAULTSET"=99, "REG_RF_RSSITRIM"=100, "REG_RF_TXIFOSCTUNE"=101, "REG_RF_TXIFGAINIMB"=102, "REG_RF_TXIFLOCK"=103, "REG_RF_RXRFLNAGAINTRIM"=104, "REG_RF_RXBIASTR"=105, "REG_RF_RXGENCTRL"=106, "REG_RF_RXIFADCDECLEV"=107, "REG_RF_RXIFDETFILTERTUNE"=108, "REG_RF_RXIFFILTERTUNE"=109, "REG_RF_GENENABLES"=110, "REG_RF_SYNTH_CHANNEL"=111, "REG_TX_RAMP_RTRIM"=112, "REG_TX_RAMP_CTRIM"=113, "REG_RF_XO_TRIM"=114, "REG_RF_SYNTH_SET_TRIM"=115, "REG_RF_ADCCTRL"=116, "REG_RF_ADCOUTPUT"=117, "REG_RF_TXIFAMP"=118, "REG_RF_SYNTH_RTRIM"=119, "REG_RF_SYNTH_CTRIM"=120, "REG_RF_SYNTH_CT"=121, "REG_RF_TXMIXER_IOSTRIM_HIGH_IP"=122, "REG_RF_TXMIXER_IOSTRIM_HIGH_IN"=123, "REG_RF_TXMIXER_IOSTRIM_HIGH_QP"=124, "REG_RF_TXMIXER_IOSTRIM_HIGH_QN"=125, "REG_HX_WUADDR"=126, "REG_REVISION"=127, "REG_NOREG_TEST"=128, "REG_DTEST_RXBUFF"=129, "REG_RXBUFF_NEXT_BLOCK"=130, "REG_RXBUFF_FIRST_IN_PACK"=131, "REG_RXBUFF_FIRST_EMPTY"=132, "REG_MAC_BYPASS"=133, "REG_DTEST_TXBUFF"=134, "REG_TXBUFF_NEXT_BLOCK"=135, "REG_TXBUFF_FIRST_IN_PACK"=136, "REG_TXBUFF_FIRST_EMPTY"=137, "REG_DTEST_SEQ"=138, "REG_DTEST_CKCORR"=139, "REG_MAC_TOPSTATE"=140, "REG_DTEST_INTERFACE"=141, "REG_IFACE_TXRX_BYPASS"=142, "REG_MAC_TXRXWAIT"=143, "REG_MAC_TXRFRAMP"=144, "REG_MAC_TRAINWORD"=145, "REG_MAC_TRAINWORD2"=146, "REG_MAC_SETTINGS"=147, "REG_MAC_CALSELECT1"=148, "REG_MAC_CALSELECT2"=149, "REG_MAC_ANTMATCHSEL"=150, "REG_MAC_ANTTUNESEL1"=151, "REG_MAC_ANTTUNESEL2"=152, "REG_MAC_ANTTUNESEL3"=153, "REG_MAC_ANTTUNESTEP"=154, "REG_MAC_WUMODEBURST"=156, "REG_MAC_WUOFFSHORT"=157, "REG_MAC_WUOFFLONG"=158, "REG_MAC_CLKRECCTRL"=159, "REG_HK_MODE_P2"=162, "REG_MAC_ANTTUNERES1"=164, "REG_MAC_ANTTUNERES2"=165, "REG_INTERFACE_MODE_TEST"=171, "REG_TXRXBUFF_BOTH_P2"=172, "REG_TXRXBUFF_P2"=173, "REG_IRQ_RAWSTATUS1_P2"=174, "REG_MAC_TXIFSTATUS1"=176, "REG_MAC_TXIFSTATUS2"=177, "REG_IRQ_RAWSTATUS2_P2"=178, "REG_MAC_TXIFRAMPDELAY"=179, "REG_MAC_TXIFRAMPSLOPE"=180, "REG_MAX_TXIFRAMP"=181, "REG_IRQ_STATUS1_P2"=182, "REG_IRQ_STATUS2_P2"=183, "REG_IRQ_AUXSTATUS_P2"=184, "REG_MAC_UNLOCK"=188, "REG_MAC_TXIFFREQ"=190, "REG_WAKEUP_TESTCTRL1"=192, "REG_WAKEUP_RX_EN_CNT"=193, "REG_WAKEUP_TESTENABLES"=194, "REG_WAKEUP_DTBI_CTRL"=195, "REG_WAKEUP_DTBO_CTRL"=196, "REG_WAKEUP_TESTIOBUFTEST"=197, "REG_WAKEUP_WK_RX_TESTCTRL1"=198, "REG_WAKEUP_WK_RX_TESTCTRL2"=199, "REG_WAKEUP_SENS_SEQUENCE_CTRL"=200, "REG_WAKEUP_LNABIAS"=201, "REG_WAKEUP_DET_TH_TRIM1"=202, "REG_WAKEUP_LNABIAS_NOM1"=203, "REG_WAKEUP_RX_TSHORT_TRIM1"=204, "REG_WAKEUP_LNABIAS_NOM2"=205, "REG_WAKEUP_RX_TLONG_TRIM1"=206, "REG_WAKEUP_LNA_NEGRTRIM_NOM1"=207, "REG_WAKEUP_RX_TBURST_TRIM1"=208, "REG_WAKEUP_RX_LNA_NEGRTRIM_NOM2"=209, "REG_WAKEUP_RX_BB_G_BW_SEL1"=210, "REG_WAKEUP_WK_RX_DET_IOSTRIM1"=212, "REG_WAKEUP_WK_RX_CTRL2"=214, "REG_WAKEUP_WK_RX_RSSIVOSTRIM"=215, "REG_WAKEUP_LNANEGR_EFF"=216, "REG_WAKEUP_XOSU_FAST"=217, "REG_WAKEUP_STROSCPWIDTH1"=218, "REG_WAKEUP_STROSCPERIOD1"=220, "REG_WAKEUP_STROSCPERIOD2"=221, "REG_WAKEUP_WK_RX_LNA_NEGRTRIM1"=222, "REG_RF_TXTESTENABLE"=224, "REG_RF_TXIFTESTMODE"=225, "REG_RF_RXTESTENABLE"=226, "REG_RF_RXIFTESTCTRL1"=227, "REG_RF_RXIFTESTCTRL2"=228, "REG_RF_RXIFTESTCTRL3"=229, "REG_RF_SYNTH_TESTCTRL1"=230, "REG_RF_SYNTH_TESTCTRL2"=231, "REG_RF_SYNTH_TESTCTRL3"=232, "REG_RF_ADCTEST1"=237, "REG_RF_ADCTEST2"=238, "REG_RF_TXMIXER_IOSTRIM_LOW_IP"=240, "REG_RF_TXMIXER_IOSTRIM_LOW_IN"=241, "REG_RF_TXMIXER_ISOTRIM_LOW_QP"=242, "REG_RF_TXMIXER_IOSTRIM_LOW_QN"=243, "REG_RF_SYNTH_KPD"=244, "REG_RF_SYNTH_LOLEV"=245, "REG_RF_TXRFPWRTUNEANTSET"=246, "REG_RF_TXPD_GAIN_CTRL"=247, "REG_RF_SYNTH_STARTUP"=248, "REG_RF_TXRFANTTUNE_TXMODE"=249, "REG_RF_TXRFANTTUNE_RXMODE"=250, "REG_RF_RXRFANTTUNE_TXMODE"=251, "REG_RF_RXRFANTTUNE_RXMODE"=252, "REG_ANTMATCH1"=253, "REG_ANTMATCH2"=254, "REG_REVISION_P2"=255] ("Register")
  w18 = u16 65 items=["---MANUAL ENTRY---"=1000, "REG_NOREG"=0, "REG_RXBUFF_USED"=1, "REG_RXBUFF_BSIZE"=2, "REG_TXBUFF_USED"=3, "REG_TXBUFF_BSIZE"=4, "REG_TXBUFF_MAXPACKSIZE"=5, "REG_MAC_ERRCLR"=6, "REG_MAC_TRAINNUM"=7, "REG_MAC_SYNCMATCH"=8, "REG_MAC_SYNC1"=9, "REG_MAC_SYNC2"=10, "REG_MAC_SYNC3"=11, "REG_MAC_SYNC4"=12, "REG_MAC_SYNC5"=13, "REG_MAC_MAXBERR"=14, "REG_MAC_ECCORR"=15, "REG_MAC_CRCERR"=16, "REG_MAC_BLKCNT1"=17, "REG_MAC_BLKCNT2"=18, "REG_MAC_IMDTRANSID1"=19, "REG_MAC_IMDTRANSID2"=20, "REG_MAC_IMDTRANSID3"=21, "REG_MAC_COMPANYID"=22, "REG_MAC_MODUSER"=23, "REG_MAC_CHANNEL"=25, "REG_MAC_CLEARWDOG"=26, "REG_MAC_CKCORRTHRESH"=27, "REG_HK_TXADDR"=28, "REG_HK_TXDATA"=29, "REG_HK_TXREPLY"=30, "REG_HK_USERDATA"=31, "REG_HK_USERSTATUS"=32, "REG_HK_LASTADDRESS"=33, "REG_HK_MODE"=34, "REG_MAC_STATUSSEQ"=35, "REG_MAC_MAXRETRIES"=36, "REG_MAC_RESENDTIME"=37, "REG_MAC_POWERSAVETIME"=38, "REG_MAC_HEAD_DET"=39, "REG_MAC_CTRL"=41, "REG_MAC_INITCOM"=42, "REG_INTERFACE_MODE"=43, "REG_TXRXBUFF_BOTH"=44, "REG_TXRXBUFF"=45, "REG_IRQ_RAWSTATUS1"=46, "REG_IRQ_ENABLE1"=47, "REG_IRQ_ENABLESET1"=48, "REG_IRQ_ENABLECLEAR1"=49, "REG_IRQ_RAWSTATUS2"=50, "REG_IRQ_ENABLE2"=51, "REG_IRQ_ENABLESET2"=52, "REG_IRQ_ENABLECLEAR2"=53, "REG_IRQ_STATUS1"=54, "REG_IRQ_STATUS2"=55, "REG_IRQ_AUXSTATUS"=56, "REG_TXBUFF_OVERFLOW"=57, "REG_PO0"=58, "REG_P01"=59, "REG_P02"=60, "REG_P03"=61, "REG_GP0"=62, "REG_GPI"=63, "REG_WAKEUP_245IN"=64, "REG_WAKEUP_COMPANYID"=65, "REG_WAKEUP_IMDTRANSID1"=66, "REG_WAKEUP_IMDTRANSID2"=67, "REG_WAKEUP_IMDTRANSID3"=68, "REG_WAKEUP_CHANNEL"=69, "REG_WAKEUP_MODUSER"=70, "REG_WAKEUP_DEVICEMODE"=71, "REG_WAKEUP_WK_RX_CTRL1"=72, "REG_WAKEUP_STACK_ADDR"=73, "REG_WAKEUP_CTRL"=74, "REG_WAKEUP_STROSCRTRIM"=75, "REG_WAKEUP_BIASTRIM"=76, "REG_WAKEUP_ANT245TUNE"=77, "REG_WAKEUP_WK_RX_RTRIMDET"=78, "REG_WAKEUP_WK_RX_RTRIMDEMOD"=79, "REG_WAKEUP_WK_RX_RSSIGAIN"=80, "REG_WAKEUP_LNAFREQ1"=81, "REG_WAKEUP_STACK"=83, "REG_WAKUP_XOSU"=84, "REG_WAKUP_CNTDROPOUT"=85, "REG_WAKEUP_CRCCTRL"=86, "REG_WAKEUP_CRCWORD1"=87, "REG_WAKEUP_CRCWORD2"=88, "REG_WAKEUP_WK_RX_CTRIM"=89, "REG_WAKEUP_VDDATRIM"=90, "REG_WAKEUP_VDDDTRIM"=91, "REG_WAKEUP_TESTIOBUFEN"=92, "REG_WAKEUP_TESTIOCLAMP"=93, "CORE_RESET_ADDRESS"=94, "CHIP_RESET_ADDRESS"=95, "REG_RF_TXGENCTRL"=96, "REG_RF_TXIFCTRL"=97, "REG_RF_TXRF_SEL_CTRL"=98, "REG_RF_TXRFPWRDEFAULTSET"=99, "REG_RF_RSSITRIM"=100, "REG_RF_TXIFOSCTUNE"=101, "REG_RF_TXIFGAINIMB"=102, "REG_RF_TXIFLOCK"=103, "REG_RF_RXRFLNAGAINTRIM"=104, "REG_RF_RXBIASTR"=105, "REG_RF_RXGENCTRL"=106, "REG_RF_RXIFADCDECLEV"=107, "REG_RF_RXIFDETFILTERTUNE"=108, "REG_RF_RXIFFILTERTUNE"=109, "REG_RF_GENENABLES"=110, "REG_RF_SYNTH_CHANNEL"=111, "REG_TX_RAMP_RTRIM"=112, "REG_TX_RAMP_CTRIM"=113, "REG_RF_XO_TRIM"=114, "REG_RF_SYNTH_SET_TRIM"=115, "REG_RF_ADCCTRL"=116, "REG_RF_ADCOUTPUT"=117, "REG_RF_TXIFAMP"=118, "REG_RF_SYNTH_RTRIM"=119, "REG_RF_SYNTH_CTRIM"=120, "REG_RF_SYNTH_CT"=121, "REG_RF_TXMIXER_IOSTRIM_HIGH_IP"=122, "REG_RF_TXMIXER_IOSTRIM_HIGH_IN"=123, "REG_RF_TXMIXER_IOSTRIM_HIGH_QP"=124, "REG_RF_TXMIXER_IOSTRIM_HIGH_QN"=125, "REG_HX_WUADDR"=126, "REG_REVISION"=127, "REG_NOREG_TEST"=128, "REG_DTEST_RXBUFF"=129, "REG_RXBUFF_NEXT_BLOCK"=130, "REG_RXBUFF_FIRST_IN_PACK"=131, "REG_RXBUFF_FIRST_EMPTY"=132, "REG_MAC_BYPASS"=133, "REG_DTEST_TXBUFF"=134, "REG_TXBUFF_NEXT_BLOCK"=135, "REG_TXBUFF_FIRST_IN_PACK"=136, "REG_TXBUFF_FIRST_EMPTY"=137, "REG_DTEST_SEQ"=138, "REG_DTEST_CKCORR"=139, "REG_MAC_TOPSTATE"=140, "REG_DTEST_INTERFACE"=141, "REG_IFACE_TXRX_BYPASS"=142, "REG_MAC_TXRXWAIT"=143, "REG_MAC_TXRFRAMP"=144, "REG_MAC_TRAINWORD"=145, "REG_MAC_TRAINWORD2"=146, "REG_MAC_SETTINGS"=147, "REG_MAC_CALSELECT1"=148, "REG_MAC_CALSELECT2"=149, "REG_MAC_ANTMATCHSEL"=150, "REG_MAC_ANTTUNESEL1"=151, "REG_MAC_ANTTUNESEL2"=152, "REG_MAC_ANTTUNESEL3"=153, "REG_MAC_ANTTUNESTEP"=154, "REG_MAC_WUMODEBURST"=156, "REG_MAC_WUOFFSHORT"=157, "REG_MAC_WUOFFLONG"=158, "REG_MAC_CLKRECCTRL"=159, "REG_HK_MODE_P2"=162, "REG_MAC_ANTTUNERES1"=164, "REG_MAC_ANTTUNERES2"=165, "REG_INTERFACE_MODE_TEST"=171, "REG_TXRXBUFF_BOTH_P2"=172, "REG_TXRXBUFF_P2"=173, "REG_IRQ_RAWSTATUS1_P2"=174, "REG_MAC_TXIFSTATUS1"=176, "REG_MAC_TXIFSTATUS2"=177, "REG_IRQ_RAWSTATUS2_P2"=178, "REG_MAC_TXIFRAMPDELAY"=179, "REG_MAC_TXIFRAMPSLOPE"=180, "REG_MAX_TXIFRAMP"=181, "REG_IRQ_STATUS1_P2"=182, "REG_IRQ_STATUS2_P2"=183, "REG_IRQ_AUXSTATUS_P2"=184, "REG_MAC_UNLOCK"=188, "REG_MAC_TXIFFREQ"=190, "REG_WAKEUP_TESTCTRL1"=192, "REG_WAKEUP_RX_EN_CNT"=193, "REG_WAKEUP_TESTENABLES"=194, "REG_WAKEUP_DTBI_CTRL"=195, "REG_WAKEUP_DTBO_CTRL"=196, "REG_WAKEUP_TESTIOBUFTEST"=197, "REG_WAKEUP_WK_RX_TESTCTRL1"=198, "REG_WAKEUP_WK_RX_TESTCTRL2"=199, "REG_WAKEUP_SENS_SEQUENCE_CTRL"=200, "REG_WAKEUP_LNABIAS"=201, "REG_WAKEUP_DET_TH_TRIM1"=202, "REG_WAKEUP_LNABIAS_NOM1"=203, "REG_WAKEUP_RX_TSHORT_TRIM1"=204, "REG_WAKEUP_LNABIAS_NOM2"=205, "REG_WAKEUP_RX_TLONG_TRIM1"=206, "REG_WAKEUP_LNA_NEGRTRIM_NOM1"=207, "REG_WAKEUP_RX_TBURST_TRIM1"=208, "REG_WAKEUP_RX_LNA_NEGRTRIM_NOM2"=209, "REG_WAKEUP_RX_BB_G_BW_SEL1"=210, "REG_WAKEUP_WK_RX_DET_IOSTRIM1"=212, "REG_WAKEUP_WK_RX_CTRL2"=214, "REG_WAKEUP_WK_RX_RSSIVOSTRIM"=215, "REG_WAKEUP_LNANEGR_EFF"=216, "REG_WAKEUP_XOSU_FAST"=217, "REG_WAKEUP_STROSCPWIDTH1"=218, "REG_WAKEUP_STROSCPERIOD1"=220, "REG_WAKEUP_STROSCPERIOD2"=221, "REG_WAKEUP_WK_RX_LNA_NEGRTRIM1"=222, "REG_RF_TXTESTENABLE"=224, "REG_RF_TXIFTESTMODE"=225, "REG_RF_RXTESTENABLE"=226, "REG_RF_RXIFTESTCTRL1"=227, "REG_RF_RXIFTESTCTRL2"=228, "REG_RF_RXIFTESTCTRL3"=229, "REG_RF_SYNTH_TESTCTRL1"=230, "REG_RF_SYNTH_TESTCTRL2"=231, "REG_RF_SYNTH_TESTCTRL3"=232, "REG_RF_ADCTEST1"=237, "REG_RF_ADCTEST2"=238, "REG_RF_TXMIXER_IOSTRIM_LOW_IP"=240, "REG_RF_TXMIXER_IOSTRIM_LOW_IN"=241, "REG_RF_TXMIXER_ISOTRIM_LOW_QP"=242, "REG_RF_TXMIXER_IOSTRIM_LOW_QN"=243, "REG_RF_SYNTH_KPD"=244, "REG_RF_SYNTH_LOLEV"=245, "REG_RF_TXRFPWRTUNEANTSET"=246, "REG_RF_TXPD_GAIN_CTRL"=247, "REG_RF_SYNTH_STARTUP"=248, "REG_RF_TXRFANTTUNE_TXMODE"=249, "REG_RF_TXRFANTTUNE_RXMODE"=250, "REG_RF_RXRFANTTUNE_TXMODE"=251, "REG_RF_RXRFANTTUNE_RXMODE"=252, "REG_ANTMATCH1"=253, "REG_ANTMATCH2"=254, "REG_REVISION_P2"=255] ("Register")
  w28 = u16 2 items=["Power ASIC", "Stim ASIC", "MICS Radio", "FRAM"] ("Target")
  w29 = u16 6 items=["Power UP", "Power DN", "Write Single", "Read Single", "Write Block", "Read Block", "Write Masked", "Test Value"] ("Function")
  w35 = u16 5 items=["Initialize COMMs", "Release COMMs", "Initialize Variables", "Select 1MHz DCO", "Select 8MHz DCO", "Standard Startup", "Standard Shutdown"] ("Function")
  w41 = u16 205 items=["READ_IO_VARS"=0, "PORT_OUT"=1, "PORT_SEL"=2, "PORT_REN"=3, "PORT_IN"=4, "PORT_DIR"=5, "SET_LCM"=6, "PWR_WRITE_SINGLE"=12, "PWR_READ_SINGLE"=13, "PWR_WRITE_MASK"=16, "PWR_WRITE_TRIM_DEFAULTS"=17, "STIM_POWER_UP"=20, "STIM_POWER_DN"=21, "STIM_WRITE_SINGLE"=22, "STIM_READ_SINGLE"=23, "STIM_WRITE_BLOCK"=24, "STIM_READ_BLOCK"=25, "STIM_WRITE_MASK"=26, "MICS_POWER_UP"=30, "MICS_WAKEUP_PULSE"=205, "MICS_POWER_DN"=31, "MICS_WRITE_SINGLE"=32, "MICS_READ_SINGLE"=33, "MICS_WRITE_BLOCK"=34, "MICS_READ_BLOCK"=35, "MICS_WRITE_MASK"=36, "MEM_POWER_UP"=40, "MEM_POWER_DN"=41, "MEM_WRITE_SINGLE"=42, "MEM_READ_SINGLE"=43, "MEM_WRITE_BLOCK"=44, "MEM_READ_BLOCK"=45, "MEM_WRITE_MASK"=46, "MEM_WRITE_SR"=47, "MEM_READ_SR"=48, "MEM_WRITE_OPCODE"=49, "INIT_PORTS"=50, "INIT_COMMS"=60, "RELEASE_COMMS"=61, "INIT_VARS"=62, "DCO_1MHZ"=63, "DCO_8MHZ"=64, "STANDARD_STARTUP"=65, "SET_LCM"=66, "PLUTO_WRITE_TRIM_DEFAULTS"=67, "SATURN_DIG_STARTUP"=68, "SATURN_BBC_STARTUP"=69, "SATURN_BBC_SHUTDOWN"=70, "SATURN_AUTO_FULL_STARTUP"=71, "SATURN_FULL_SHUTDOWN"=72, "SATURN_ENABLE_PROGRAMMING"=73, "SATURN_ENABLE_SEQUENCER"=74, "START_STIM_CLK"=80, "STOP_STIM_CLK"=81, "PULSE_STIM_CLK"=82, "PULSE_STIM_SCK"=83, "SINGLE_ADC12"=85, "SINGLE_ADC12_REPEAT"=86, "MULTI_ADC12"=87, "MULTI_ADC12_REPEAT"=88, "DISABLE_ADC12"=89, "READ_CLOCK_REGISTERS"=90, "WRITE_CLOCK_REGISTERS"=91, "STIM_SOFT_START_CTL"=100, "SHUTDOWN_CTL"=101, "FRAM_CLEAR"=110, "TC_STIM_RAM_READ"=200, "TC_STIM_RAM_WRITE"=201, "TC_STIM_PHASE_REGS_READ"=202, "TC_STIM_PHASE_REGS_WRITE"=203, "TC_BROWN_OUT_TEST"=204, "TC_TIMING_TEST"=220, "TC_PIN_ECHO_TEST"=221, "ENABLE_CLK_ERR_TRAP"=230, "DISABLE_CLK_ERR_TRAP"=231, "POWER_SPI_IDLE"=300, "POWER_SPI_WAKEUP"=301, "STIM_SPI_IDLE"=302, "STIM_SPI_WAKEUP"=303, "SHUTDOWN"=999] ("Function")
  w42 = u16 30 items=["READ_IO_VARS"=0, "PORT_OUT"=1, "PORT_SEL"=2, "PORT_REN"=3, "PORT_IN"=4, "PORT_DIR"=5, "SET_LCM"=6, "PWR_WRITE_SINGLE"=12, "PWR_READ_SINGLE"=13, "PWR_WRITE_MASK"=16, "PWR_WRITE_TRIM_DEFAULTS"=17, "STIM_POWER_UP"=20, "STIM_POWER_DN"=21, "STIM_WRITE_SINGLE"=22, "STIM_READ_SINGLE"=23, "STIM_WRITE_BLOCK"=24, "STIM_READ_BLOCK"=25, "STIM_WRITE_MASK"=26, "MICS_POWER_UP"=30, "MICS_WAKEUP_PULSE"=205, "MICS_POWER_DN"=31, "MICS_WRITE_SINGLE"=32, "MICS_READ_SINGLE"=33, "MICS_WRITE_BLOCK"=34, "MICS_READ_BLOCK"=35, "MICS_WRITE_MASK"=36, "MEM_POWER_UP"=40, "MEM_POWER_DN"=41, "MEM_WRITE_SINGLE"=42, "MEM_READ_SINGLE"=43, "MEM_WRITE_BLOCK"=44, "MEM_READ_BLOCK"=45, "MEM_WRITE_MASK"=46, "MEM_WRITE_SR"=47, "MEM_READ_SR"=48, "MEM_WRITE_OPCODE"=49, "INIT_PORTS"=50, "INIT_COMMS"=60, "RELEASE_COMMS"=61, "INIT_VARS"=62, "DCO_1MHZ"=63, "DCO_8MHZ"=64, "STANDARD_STARTUP"=65, "SET_LCM"=66, "PLUTO_WRITE_TRIM_DEFAULTS"=67, "SATURN_DIG_STARTUP"=68, "SATURN_BBC_STARTUP"=69, "SATURN_BBC_SHUTDOWN"=70, "SATURN_AUTO_FULL_STARTUP"=71, "SATURN_FULL_SHUTDOWN"=72, "SATURN_ENABLE_PROGRAMMING"=73, "SATURN_ENABLE_SEQUENCER"=74, "START_STIM_CLK"=80, "STOP_STIM_CLK"=81, "PULSE_STIM_CLK"=82, "PULSE_STIM_SCK"=83, "SINGLE_ADC12"=85, "SINGLE_ADC12_REPEAT"=86, "MULTI_ADC12"=87, "MULTI_ADC12_REPEAT"=88, "DISABLE_ADC12"=89, "READ_CLOCK_REGISTERS"=90, "WRITE_CLOCK_REGISTERS"=91, "STIM_SOFT_START_CTL"=100, "SHUTDOWN_CTL"=101, "FRAM_CLEAR"=110, "TC_STIM_RAM_READ"=200, "TC_STIM_RAM_WRITE"=201, "TC_STIM_PHASE_REGS_READ"=202, "TC_STIM_PHASE_REGS_WRITE"=203, "TC_BROWN_OUT_TEST"=204, "TC_TIMING_TEST"=220, "TC_PIN_ECHO_TEST"=221, "ENABLE_CLK_ERR_TRAP"=230, "DISABLE_CLK_ERR_TRAP"=231, "POWER_SPI_IDLE"=300, "POWER_SPI_WAKEUP"=301, "STIM_SPI_IDLE"=302, "STIM_SPI_WAKEUP"=303, "SHUTDOWN"=999] ("Function")
  w54 = u16 3 items=["Power UP", "Power DN", "Write Single", "Read Single", "Write Block", "Read Block", "Write Masked", "Test Value"] ("Function")
  w20 = u16 2 items=["Power ASIC", "Stim ASIC", "MICS Radio", "FRAM"] ("Target")
  w19 = u16 2 items=["Power UP", "Power DN", "Write Single", "Read Single", "Write Block", "Read Block", "Write Masked", "Test Value"] ("Function")
  w56 = u16 200 items=["---MANUAL ENTRY---"=1000, "REG_NOREG"=0, "REG_RXBUFF_USED"=1, "REG_RXBUFF_BSIZE"=2, "REG_TXBUFF_USED"=3, "REG_TXBUFF_BSIZE"=4, "REG_TXBUFF_MAXPACKSIZE"=5, "REG_MAC_ERRCLR"=6, "REG_MAC_TRAINNUM"=7, "REG_MAC_SYNCMATCH"=8, "REG_MAC_SYNC1"=9, "REG_MAC_SYNC2"=10, "REG_MAC_SYNC3"=11, "REG_MAC_SYNC4"=12, "REG_MAC_SYNC5"=13, "REG_MAC_MAXBERR"=14, "REG_MAC_ECCORR"=15, "REG_MAC_CRCERR"=16, "REG_MAC_BLKCNT1"=17, "REG_MAC_BLKCNT2"=18, "REG_MAC_IMDTRANSID1"=19, "REG_MAC_IMDTRANSID2"=20, "REG_MAC_IMDTRANSID3"=21, "REG_MAC_COMPANYID"=22, "REG_MAC_MODUSER"=23, "REG_MAC_CHANNEL"=25, "REG_MAC_CLEARWDOG"=26, "REG_MAC_CKCORRTHRESH"=27, "REG_HK_TXADDR"=28, "REG_HK_TXDATA"=29, "REG_HK_TXREPLY"=30, "REG_HK_USERDATA"=31, "REG_HK_USERSTATUS"=32, "REG_HK_LASTADDRESS"=33, "REG_HK_MODE"=34, "REG_MAC_STATUSSEQ"=35, "REG_MAC_MAXRETRIES"=36, "REG_MAC_RESENDTIME"=37, "REG_MAC_POWERSAVETIME"=38, "REG_MAC_HEAD_DET"=39, "REG_MAC_CTRL"=41, "REG_MAC_INITCOM"=42, "REG_INTERFACE_MODE"=43, "REG_TXRXBUFF_BOTH"=44, "REG_TXRXBUFF"=45, "REG_IRQ_RAWSTATUS1"=46, "REG_IRQ_ENABLE1"=47, "REG_IRQ_ENABLESET1"=48, "REG_IRQ_ENABLECLEAR1"=49, "REG_IRQ_RAWSTATUS2"=50, "REG_IRQ_ENABLE2"=51, "REG_IRQ_ENABLESET2"=52, "REG_IRQ_ENABLECLEAR2"=53, "REG_IRQ_STATUS1"=54, "REG_IRQ_STATUS2"=55, "REG_IRQ_AUXSTATUS"=56, "REG_TXBUFF_OVERFLOW"=57, "REG_PO0"=58, "REG_P01"=59, "REG_P02"=60, "REG_P03"=61, "REG_GP0"=62, "REG_GPI"=63, "REG_WAKEUP_245IN"=64, "REG_WAKEUP_COMPANYID"=65, "REG_WAKEUP_IMDTRANSID1"=66, "REG_WAKEUP_IMDTRANSID2"=67, "REG_WAKEUP_IMDTRANSID3"=68, "REG_WAKEUP_CHANNEL"=69, "REG_WAKEUP_MODUSER"=70, "REG_WAKEUP_DEVICEMODE"=71, "REG_WAKEUP_WK_RX_CTRL1"=72, "REG_WAKEUP_STACK_ADDR"=73, "REG_WAKEUP_CTRL"=74, "REG_WAKEUP_STROSCRTRIM"=75, "REG_WAKEUP_BIASTRIM"=76, "REG_WAKEUP_ANT245TUNE"=77, "REG_WAKEUP_WK_RX_RTRIMDET"=78, "REG_WAKEUP_WK_RX_RTRIMDEMOD"=79, "REG_WAKEUP_WK_RX_RSSIGAIN"=80, "REG_WAKEUP_LNAFREQ1"=81, "REG_WAKEUP_STACK"=83, "REG_WAKUP_XOSU"=84, "REG_WAKUP_CNTDROPOUT"=85, "REG_WAKEUP_CRCCTRL"=86, "REG_WAKEUP_CRCWORD1"=87, "REG_WAKEUP_CRCWORD2"=88, "REG_WAKEUP_WK_RX_CTRIM"=89, "REG_WAKEUP_VDDATRIM"=90, "REG_WAKEUP_VDDDTRIM"=91, "REG_WAKEUP_TESTIOBUFEN"=92, "REG_WAKEUP_TESTIOCLAMP"=93, "CORE_RESET_ADDRESS"=94, "CHIP_RESET_ADDRESS"=95, "REG_RF_TXGENCTRL"=96, "REG_RF_TXIFCTRL"=97, "REG_RF_TXRF_SEL_CTRL"=98, "REG_RF_TXRFPWRDEFAULTSET"=99, "REG_RF_RSSITRIM"=100, "REG_RF_TXIFOSCTUNE"=101, "REG_RF_TXIFGAINIMB"=102, "REG_RF_TXIFLOCK"=103, "REG_RF_RXRFLNAGAINTRIM"=104, "REG_RF_RXBIASTR"=105, "REG_RF_RXGENCTRL"=106, "REG_RF_RXIFADCDECLEV"=107, "REG_RF_RXIFDETFILTERTUNE"=108, "REG_RF_RXIFFILTERTUNE"=109, "REG_RF_GENENABLES"=110, "REG_RF_SYNTH_CHANNEL"=111, "REG_TX_RAMP_RTRIM"=112, "REG_TX_RAMP_CTRIM"=113, "REG_RF_XO_TRIM"=114, "REG_RF_SYNTH_SET_TRIM"=115, "REG_RF_ADCCTRL"=116, "REG_RF_ADCOUTPUT"=117, "REG_RF_TXIFAMP"=118, "REG_RF_SYNTH_RTRIM"=119, "REG_RF_SYNTH_CTRIM"=120, "REG_RF_SYNTH_CT"=121, "REG_RF_TXMIXER_IOSTRIM_HIGH_IP"=122, "REG_RF_TXMIXER_IOSTRIM_HIGH_IN"=123, "REG_RF_TXMIXER_IOSTRIM_HIGH_QP"=124, "REG_RF_TXMIXER_IOSTRIM_HIGH_QN"=125, "REG_HX_WUADDR"=126, "REG_REVISION"=127, "REG_NOREG_TEST"=128, "REG_DTEST_RXBUFF"=129, "REG_RXBUFF_NEXT_BLOCK"=130, "REG_RXBUFF_FIRST_IN_PACK"=131, "REG_RXBUFF_FIRST_EMPTY"=132, "REG_MAC_BYPASS"=133, "REG_DTEST_TXBUFF"=134, "REG_TXBUFF_NEXT_BLOCK"=135, "REG_TXBUFF_FIRST_IN_PACK"=136, "REG_TXBUFF_FIRST_EMPTY"=137, "REG_DTEST_SEQ"=138, "REG_DTEST_CKCORR"=139, "REG_MAC_TOPSTATE"=140, "REG_DTEST_INTERFACE"=141, "REG_IFACE_TXRX_BYPASS"=142, "REG_MAC_TXRXWAIT"=143, "REG_MAC_TXRFRAMP"=144, "REG_MAC_TRAINWORD"=145, "REG_MAC_TRAINWORD2"=146, "REG_MAC_SETTINGS"=147, "REG_MAC_CALSELECT1"=148, "REG_MAC_CALSELECT2"=149, "REG_MAC_ANTMATCHSEL"=150, "REG_MAC_ANTTUNESEL1"=151, "REG_MAC_ANTTUNESEL2"=152, "REG_MAC_ANTTUNESEL3"=153, "REG_MAC_ANTTUNESTEP"=154, "REG_MAC_WUMODEBURST"=156, "REG_MAC_WUOFFSHORT"=157, "REG_MAC_WUOFFLONG"=158, "REG_MAC_CLKRECCTRL"=159, "REG_HK_MODE_P2"=162, "REG_MAC_ANTTUNERES1"=164, "REG_MAC_ANTTUNERES2"=165, "REG_INTERFACE_MODE_TEST"=171, "REG_TXRXBUFF_BOTH_P2"=172, "REG_TXRXBUFF_P2"=173, "REG_IRQ_RAWSTATUS1_P2"=174, "REG_MAC_TXIFSTATUS1"=176, "REG_MAC_TXIFSTATUS2"=177, "REG_IRQ_RAWSTATUS2_P2"=178, "REG_MAC_TXIFRAMPDELAY"=179, "REG_MAC_TXIFRAMPSLOPE"=180, "REG_MAX_TXIFRAMP"=181, "REG_IRQ_STATUS1_P2"=182, "REG_IRQ_STATUS2_P2"=183, "REG_IRQ_AUXSTATUS_P2"=184, "REG_MAC_UNLOCK"=188, "REG_MAC_TXIFFREQ"=190, "REG_WAKEUP_TESTCTRL1"=192, "REG_WAKEUP_RX_EN_CNT"=193, "REG_WAKEUP_TESTENABLES"=194, "REG_WAKEUP_DTBI_CTRL"=195, "REG_WAKEUP_DTBO_CTRL"=196, "REG_WAKEUP_TESTIOBUFTEST"=197, "REG_WAKEUP_WK_RX_TESTCTRL1"=198, "REG_WAKEUP_WK_RX_TESTCTRL2"=199, "REG_WAKEUP_SENS_SEQUENCE_CTRL"=200, "REG_WAKEUP_LNABIAS"=201, "REG_WAKEUP_DET_TH_TRIM1"=202, "REG_WAKEUP_LNABIAS_NOM1"=203, "REG_WAKEUP_RX_TSHORT_TRIM1"=204, "REG_WAKEUP_LNABIAS_NOM2"=205, "REG_WAKEUP_RX_TLONG_TRIM1"=206, "REG_WAKEUP_LNA_NEGRTRIM_NOM1"=207, "REG_WAKEUP_RX_TBURST_TRIM1"=208, "REG_WAKEUP_RX_LNA_NEGRTRIM_NOM2"=209, "REG_WAKEUP_RX_BB_G_BW_SEL1"=210, "REG_WAKEUP_WK_RX_DET_IOSTRIM1"=212, "REG_WAKEUP_WK_RX_CTRL2"=214, "REG_WAKEUP_WK_RX_RSSIVOSTRIM"=215, "REG_WAKEUP_LNANEGR_EFF"=216, "REG_WAKEUP_XOSU_FAST"=217, "REG_WAKEUP_STROSCPWIDTH1"=218, "REG_WAKEUP_STROSCPERIOD1"=220, "REG_WAKEUP_STROSCPERIOD2"=221, "REG_WAKEUP_WK_RX_LNA_NEGRTRIM1"=222, "REG_RF_TXTESTENABLE"=224, "REG_RF_TXIFTESTMODE"=225, "REG_RF_RXTESTENABLE"=226, "REG_RF_RXIFTESTCTRL1"=227, "REG_RF_RXIFTESTCTRL2"=228, "REG_RF_RXIFTESTCTRL3"=229, "REG_RF_SYNTH_TESTCTRL1"=230, "REG_RF_SYNTH_TESTCTRL2"=231, "REG_RF_SYNTH_TESTCTRL3"=232, "REG_RF_ADCTEST1"=237, "REG_RF_ADCTEST2"=238, "REG_RF_TXMIXER_IOSTRIM_LOW_IP"=240, "REG_RF_TXMIXER_IOSTRIM_LOW_IN"=241, "REG_RF_TXMIXER_ISOTRIM_LOW_QP"=242, "REG_RF_TXMIXER_IOSTRIM_LOW_QN"=243, "REG_RF_SYNTH_KPD"=244, "REG_RF_SYNTH_LOLEV"=245, "REG_RF_TXRFPWRTUNEANTSET"=246, "REG_RF_TXPD_GAIN_CTRL"=247, "REG_RF_SYNTH_STARTUP"=248, "REG_RF_TXRFANTTUNE_TXMODE"=249, "REG_RF_TXRFANTTUNE_RXMODE"=250, "REG_RF_RXRFANTTUNE_TXMODE"=251, "REG_RF_RXRFANTTUNE_RXMODE"=252, "REG_ANTMATCH1"=253, "REG_ANTMATCH2"=254, "REG_REVISION_P2"=255] ("Register")
  w59 = u16 214 items=["---MANUAL ENTRY---"=1000, "REG_NOREG"=0, "REG_RXBUFF_USED"=1, "REG_RXBUFF_BSIZE"=2, "REG_TXBUFF_USED"=3, "REG_TXBUFF_BSIZE"=4, "REG_TXBUFF_MAXPACKSIZE"=5, "REG_MAC_ERRCLR"=6, "REG_MAC_TRAINNUM"=7, "REG_MAC_SYNCMATCH"=8, "REG_MAC_SYNC1"=9, "REG_MAC_SYNC2"=10, "REG_MAC_SYNC3"=11, "REG_MAC_SYNC4"=12, "REG_MAC_SYNC5"=13, "REG_MAC_MAXBERR"=14, "REG_MAC_ECCORR"=15, "REG_MAC_CRCERR"=16, "REG_MAC_BLKCNT1"=17, "REG_MAC_BLKCNT2"=18, "REG_MAC_IMDTRANSID1"=19, "REG_MAC_IMDTRANSID2"=20, "REG_MAC_IMDTRANSID3"=21, "REG_MAC_COMPANYID"=22, "REG_MAC_MODUSER"=23, "REG_MAC_CHANNEL"=25, "REG_MAC_CLEARWDOG"=26, "REG_MAC_CKCORRTHRESH"=27, "REG_HK_TXADDR"=28, "REG_HK_TXDATA"=29, "REG_HK_TXREPLY"=30, "REG_HK_USERDATA"=31, "REG_HK_USERSTATUS"=32, "REG_HK_LASTADDRESS"=33, "REG_HK_MODE"=34, "REG_MAC_STATUSSEQ"=35, "REG_MAC_MAXRETRIES"=36, "REG_MAC_RESENDTIME"=37, "REG_MAC_POWERSAVETIME"=38, "REG_MAC_HEAD_DET"=39, "REG_MAC_CTRL"=41, "REG_MAC_INITCOM"=42, "REG_INTERFACE_MODE"=43, "REG_TXRXBUFF_BOTH"=44, "REG_TXRXBUFF"=45, "REG_IRQ_RAWSTATUS1"=46, "REG_IRQ_ENABLE1"=47, "REG_IRQ_ENABLESET1"=48, "REG_IRQ_ENABLECLEAR1"=49, "REG_IRQ_RAWSTATUS2"=50, "REG_IRQ_ENABLE2"=51, "REG_IRQ_ENABLESET2"=52, "REG_IRQ_ENABLECLEAR2"=53, "REG_IRQ_STATUS1"=54, "REG_IRQ_STATUS2"=55, "REG_IRQ_AUXSTATUS"=56, "REG_TXBUFF_OVERFLOW"=57, "REG_PO0"=58, "REG_P01"=59, "REG_P02"=60, "REG_P03"=61, "REG_GP0"=62, "REG_GPI"=63, "REG_WAKEUP_245IN"=64, "REG_WAKEUP_COMPANYID"=65, "REG_WAKEUP_IMDTRANSID1"=66, "REG_WAKEUP_IMDTRANSID2"=67, "REG_WAKEUP_IMDTRANSID3"=68, "REG_WAKEUP_CHANNEL"=69, "REG_WAKEUP_MODUSER"=70, "REG_WAKEUP_DEVICEMODE"=71, "REG_WAKEUP_WK_RX_CTRL1"=72, "REG_WAKEUP_STACK_ADDR"=73, "REG_WAKEUP_CTRL"=74, "REG_WAKEUP_STROSCRTRIM"=75, "REG_WAKEUP_BIASTRIM"=76, "REG_WAKEUP_ANT245TUNE"=77, "REG_WAKEUP_WK_RX_RTRIMDET"=78, "REG_WAKEUP_WK_RX_RTRIMDEMOD"=79, "REG_WAKEUP_WK_RX_RSSIGAIN"=80, "REG_WAKEUP_LNAFREQ1"=81, "REG_WAKEUP_STACK"=83, "REG_WAKUP_XOSU"=84, "REG_WAKUP_CNTDROPOUT"=85, "REG_WAKEUP_CRCCTRL"=86, "REG_WAKEUP_CRCWORD1"=87, "REG_WAKEUP_CRCWORD2"=88, "REG_WAKEUP_WK_RX_CTRIM"=89, "REG_WAKEUP_VDDATRIM"=90, "REG_WAKEUP_VDDDTRIM"=91, "REG_WAKEUP_TESTIOBUFEN"=92, "REG_WAKEUP_TESTIOCLAMP"=93, "CORE_RESET_ADDRESS"=94, "CHIP_RESET_ADDRESS"=95, "REG_RF_TXGENCTRL"=96, "REG_RF_TXIFCTRL"=97, "REG_RF_TXRF_SEL_CTRL"=98, "REG_RF_TXRFPWRDEFAULTSET"=99, "REG_RF_RSSITRIM"=100, "REG_RF_TXIFOSCTUNE"=101, "REG_RF_TXIFGAINIMB"=102, "REG_RF_TXIFLOCK"=103, "REG_RF_RXRFLNAGAINTRIM"=104, "REG_RF_RXBIASTR"=105, "REG_RF_RXGENCTRL"=106, "REG_RF_RXIFADCDECLEV"=107, "REG_RF_RXIFDETFILTERTUNE"=108, "REG_RF_RXIFFILTERTUNE"=109, "REG_RF_GENENABLES"=110, "REG_RF_SYNTH_CHANNEL"=111, "REG_TX_RAMP_RTRIM"=112, "REG_TX_RAMP_CTRIM"=113, "REG_RF_XO_TRIM"=114, "REG_RF_SYNTH_SET_TRIM"=115, "REG_RF_ADCCTRL"=116, "REG_RF_ADCOUTPUT"=117, "REG_RF_TXIFAMP"=118, "REG_RF_SYNTH_RTRIM"=119, "REG_RF_SYNTH_CTRIM"=120, "REG_RF_SYNTH_CT"=121, "REG_RF_TXMIXER_IOSTRIM_HIGH_IP"=122, "REG_RF_TXMIXER_IOSTRIM_HIGH_IN"=123, "REG_RF_TXMIXER_IOSTRIM_HIGH_QP"=124, "REG_RF_TXMIXER_IOSTRIM_HIGH_QN"=125, "REG_HX_WUADDR"=126, "REG_REVISION"=127, "REG_NOREG_TEST"=128, "REG_DTEST_RXBUFF"=129, "REG_RXBUFF_NEXT_BLOCK"=130, "REG_RXBUFF_FIRST_IN_PACK"=131, "REG_RXBUFF_FIRST_EMPTY"=132, "REG_MAC_BYPASS"=133, "REG_DTEST_TXBUFF"=134, "REG_TXBUFF_NEXT_BLOCK"=135, "REG_TXBUFF_FIRST_IN_PACK"=136, "REG_TXBUFF_FIRST_EMPTY"=137, "REG_DTEST_SEQ"=138, "REG_DTEST_CKCORR"=139, "REG_MAC_TOPSTATE"=140, "REG_DTEST_INTERFACE"=141, "REG_IFACE_TXRX_BYPASS"=142, "REG_MAC_TXRXWAIT"=143, "REG_MAC_TXRFRAMP"=144, "REG_MAC_TRAINWORD"=145, "REG_MAC_TRAINWORD2"=146, "REG_MAC_SETTINGS"=147, "REG_MAC_CALSELECT1"=148, "REG_MAC_CALSELECT2"=149, "REG_MAC_ANTMATCHSEL"=150, "REG_MAC_ANTTUNESEL1"=151, "REG_MAC_ANTTUNESEL2"=152, "REG_MAC_ANTTUNESEL3"=153, "REG_MAC_ANTTUNESTEP"=154, "REG_MAC_WUMODEBURST"=156, "REG_MAC_WUOFFSHORT"=157, "REG_MAC_WUOFFLONG"=158, "REG_MAC_CLKRECCTRL"=159, "REG_HK_MODE_P2"=162, "REG_MAC_ANTTUNERES1"=164, "REG_MAC_ANTTUNERES2"=165, "REG_INTERFACE_MODE_TEST"=171, "REG_TXRXBUFF_BOTH_P2"=172, "REG_TXRXBUFF_P2"=173, "REG_IRQ_RAWSTATUS1_P2"=174, "REG_MAC_TXIFSTATUS1"=176, "REG_MAC_TXIFSTATUS2"=177, "REG_IRQ_RAWSTATUS2_P2"=178, "REG_MAC_TXIFRAMPDELAY"=179, "REG_MAC_TXIFRAMPSLOPE"=180, "REG_MAX_TXIFRAMP"=181, "REG_IRQ_STATUS1_P2"=182, "REG_IRQ_STATUS2_P2"=183, "REG_IRQ_AUXSTATUS_P2"=184, "REG_MAC_UNLOCK"=188, "REG_MAC_TXIFFREQ"=190, "REG_WAKEUP_TESTCTRL1"=192, "REG_WAKEUP_RX_EN_CNT"=193, "REG_WAKEUP_TESTENABLES"=194, "REG_WAKEUP_DTBI_CTRL"=195, "REG_WAKEUP_DTBO_CTRL"=196, "REG_WAKEUP_TESTIOBUFTEST"=197, "REG_WAKEUP_WK_RX_TESTCTRL1"=198, "REG_WAKEUP_WK_RX_TESTCTRL2"=199, "REG_WAKEUP_SENS_SEQUENCE_CTRL"=200, "REG_WAKEUP_LNABIAS"=201, "REG_WAKEUP_DET_TH_TRIM1"=202, "REG_WAKEUP_LNABIAS_NOM1"=203, "REG_WAKEUP_RX_TSHORT_TRIM1"=204, "REG_WAKEUP_LNABIAS_NOM2"=205, "REG_WAKEUP_RX_TLONG_TRIM1"=206, "REG_WAKEUP_LNA_NEGRTRIM_NOM1"=207, "REG_WAKEUP_RX_TBURST_TRIM1"=208, "REG_WAKEUP_RX_LNA_NEGRTRIM_NOM2"=209, "REG_WAKEUP_RX_BB_G_BW_SEL1"=210, "REG_WAKEUP_WK_RX_DET_IOSTRIM1"=212, "REG_WAKEUP_WK_RX_CTRL2"=214, "REG_WAKEUP_WK_RX_RSSIVOSTRIM"=215, "REG_WAKEUP_LNANEGR_EFF"=216, "REG_WAKEUP_XOSU_FAST"=217, "REG_WAKEUP_STROSCPWIDTH1"=218, "REG_WAKEUP_STROSCPERIOD1"=220, "REG_WAKEUP_STROSCPERIOD2"=221, "REG_WAKEUP_WK_RX_LNA_NEGRTRIM1"=222, "REG_RF_TXTESTENABLE"=224, "REG_RF_TXIFTESTMODE"=225, "REG_RF_RXTESTENABLE"=226, "REG_RF_RXIFTESTCTRL1"=227, "REG_RF_RXIFTESTCTRL2"=228, "REG_RF_RXIFTESTCTRL3"=229, "REG_RF_SYNTH_TESTCTRL1"=230, "REG_RF_SYNTH_TESTCTRL2"=231, "REG_RF_SYNTH_TESTCTRL3"=232, "REG_RF_ADCTEST1"=237, "REG_RF_ADCTEST2"=238, "REG_RF_TXMIXER_IOSTRIM_LOW_IP"=240, "REG_RF_TXMIXER_IOSTRIM_LOW_IN"=241, "REG_RF_TXMIXER_ISOTRIM_LOW_QP"=242, "REG_RF_TXMIXER_IOSTRIM_LOW_QN"=243, "REG_RF_SYNTH_KPD"=244, "REG_RF_SYNTH_LOLEV"=245, "REG_RF_TXRFPWRTUNEANTSET"=246, "REG_RF_TXPD_GAIN_CTRL"=247, "REG_RF_SYNTH_STARTUP"=248, "REG_RF_TXRFANTTUNE_TXMODE"=249, "REG_RF_TXRFANTTUNE_RXMODE"=250, "REG_RF_RXRFANTTUNE_TXMODE"=251, "REG_RF_RXRFANTTUNE_RXMODE"=252, "REG_ANTMATCH1"=253, "REG_ANTMATCH2"=254, "REG_REVISION_P2"=255] ("Register")
  w32 = u16 74 items=["---MANUAL ENTRY---"=1000, "REG_NOREG"=0, "REG_RXBUFF_USED"=1, "REG_RXBUFF_BSIZE"=2, "REG_TXBUFF_USED"=3, "REG_TXBUFF_BSIZE"=4, "REG_TXBUFF_MAXPACKSIZE"=5, "REG_MAC_ERRCLR"=6, "REG_MAC_TRAINNUM"=7, "REG_MAC_SYNCMATCH"=8, "REG_MAC_SYNC1"=9, "REG_MAC_SYNC2"=10, "REG_MAC_SYNC3"=11, "REG_MAC_SYNC4"=12, "REG_MAC_SYNC5"=13, "REG_MAC_MAXBERR"=14, "REG_MAC_ECCORR"=15, "REG_MAC_CRCERR"=16, "REG_MAC_BLKCNT1"=17, "REG_MAC_BLKCNT2"=18, "REG_MAC_IMDTRANSID1"=19, "REG_MAC_IMDTRANSID2"=20, "REG_MAC_IMDTRANSID3"=21, "REG_MAC_COMPANYID"=22, "REG_MAC_MODUSER"=23, "REG_MAC_CHANNEL"=25, "REG_MAC_CLEARWDOG"=26, "REG_MAC_CKCORRTHRESH"=27, "REG_HK_TXADDR"=28, "REG_HK_TXDATA"=29, "REG_HK_TXREPLY"=30, "REG_HK_USERDATA"=31, "REG_HK_USERSTATUS"=32, "REG_HK_LASTADDRESS"=33, "REG_HK_MODE"=34, "REG_MAC_STATUSSEQ"=35, "REG_MAC_MAXRETRIES"=36, "REG_MAC_RESENDTIME"=37, "REG_MAC_POWERSAVETIME"=38, "REG_MAC_HEAD_DET"=39, "REG_MAC_CTRL"=41, "REG_MAC_INITCOM"=42, "REG_INTERFACE_MODE"=43, "REG_TXRXBUFF_BOTH"=44, "REG_TXRXBUFF"=45, "REG_IRQ_RAWSTATUS1"=46, "REG_IRQ_ENABLE1"=47, "REG_IRQ_ENABLESET1"=48, "REG_IRQ_ENABLECLEAR1"=49, "REG_IRQ_RAWSTATUS2"=50, "REG_IRQ_ENABLE2"=51, "REG_IRQ_ENABLESET2"=52, "REG_IRQ_ENABLECLEAR2"=53, "REG_IRQ_STATUS1"=54, "REG_IRQ_STATUS2"=55, "REG_IRQ_AUXSTATUS"=56, "REG_TXBUFF_OVERFLOW"=57, "REG_PO0"=58, "REG_P01"=59, "REG_P02"=60, "REG_P03"=61, "REG_GP0"=62, "REG_GPI"=63, "REG_WAKEUP_245IN"=64, "REG_WAKEUP_COMPANYID"=65, "REG_WAKEUP_IMDTRANSID1"=66, "REG_WAKEUP_IMDTRANSID2"=67, "REG_WAKEUP_IMDTRANSID3"=68, "REG_WAKEUP_CHANNEL"=69, "REG_WAKEUP_MODUSER"=70, "REG_WAKEUP_DEVICEMODE"=71, "REG_WAKEUP_WK_RX_CTRL1"=72, "REG_WAKEUP_STACK_ADDR"=73, "REG_WAKEUP_CTRL"=74, "REG_WAKEUP_STROSCRTRIM"=75, "REG_WAKEUP_BIASTRIM"=76, "REG_WAKEUP_ANT245TUNE"=77, "REG_WAKEUP_WK_RX_RTRIMDET"=78, "REG_WAKEUP_WK_RX_RTRIMDEMOD"=79, "REG_WAKEUP_WK_RX_RSSIGAIN"=80, "REG_WAKEUP_LNAFREQ1"=81, "REG_WAKEUP_STACK"=83, "REG_WAKUP_XOSU"=84, "REG_WAKUP_CNTDROPOUT"=85, "REG_WAKEUP_CRCCTRL"=86, "REG_WAKEUP_CRCWORD1"=87, "REG_WAKEUP_CRCWORD2"=88, "REG_WAKEUP_WK_RX_CTRIM"=89, "REG_WAKEUP_VDDATRIM"=90, "REG_WAKEUP_VDDDTRIM"=91, "REG_WAKEUP_TESTIOBUFEN"=92, "REG_WAKEUP_TESTIOCLAMP"=93, "CORE_RESET_ADDRESS"=94, "CHIP_RESET_ADDRESS"=95, "REG_RF_TXGENCTRL"=96, "REG_RF_TXIFCTRL"=97, "REG_RF_TXRF_SEL_CTRL"=98, "REG_RF_TXRFPWRDEFAULTSET"=99, "REG_RF_RSSITRIM"=100, "REG_RF_TXIFOSCTUNE"=101, "REG_RF_TXIFGAINIMB"=102, "REG_RF_TXIFLOCK"=103, "REG_RF_RXRFLNAGAINTRIM"=104, "REG_RF_RXBIASTR"=105, "REG_RF_RXGENCTRL"=106, "REG_RF_RXIFADCDECLEV"=107, "REG_RF_RXIFDETFILTERTUNE"=108, "REG_RF_RXIFFILTERTUNE"=109, "REG_RF_GENENABLES"=110, "REG_RF_SYNTH_CHANNEL"=111, "REG_TX_RAMP_RTRIM"=112, "REG_TX_RAMP_CTRIM"=113, "REG_RF_XO_TRIM"=114, "REG_RF_SYNTH_SET_TRIM"=115, "REG_RF_ADCCTRL"=116, "REG_RF_ADCOUTPUT"=117, "REG_RF_TXIFAMP"=118, "REG_RF_SYNTH_RTRIM"=119, "REG_RF_SYNTH_CTRIM"=120, "REG_RF_SYNTH_CT"=121, "REG_RF_TXMIXER_IOSTRIM_HIGH_IP"=122, "REG_RF_TXMIXER_IOSTRIM_HIGH_IN"=123, "REG_RF_TXMIXER_IOSTRIM_HIGH_QP"=124, "REG_RF_TXMIXER_IOSTRIM_HIGH_QN"=125, "REG_HX_WUADDR"=126, "REG_REVISION"=127, "REG_NOREG_TEST"=128, "REG_DTEST_RXBUFF"=129, "REG_RXBUFF_NEXT_BLOCK"=130, "REG_RXBUFF_FIRST_IN_PACK"=131, "REG_RXBUFF_FIRST_EMPTY"=132, "REG_MAC_BYPASS"=133, "REG_DTEST_TXBUFF"=134, "REG_TXBUFF_NEXT_BLOCK"=135, "REG_TXBUFF_FIRST_IN_PACK"=136, "REG_TXBUFF_FIRST_EMPTY"=137, "REG_DTEST_SEQ"=138, "REG_DTEST_CKCORR"=139, "REG_MAC_TOPSTATE"=140, "REG_DTEST_INTERFACE"=141, "REG_IFACE_TXRX_BYPASS"=142, "REG_MAC_TXRXWAIT"=143, "REG_MAC_TXRFRAMP"=144, "REG_MAC_TRAINWORD"=145, "REG_MAC_TRAINWORD2"=146, "REG_MAC_SETTINGS"=147, "REG_MAC_CALSELECT1"=148, "REG_MAC_CALSELECT2"=149, "REG_MAC_ANTMATCHSEL"=150, "REG_MAC_ANTTUNESEL1"=151, "REG_MAC_ANTTUNESEL2"=152, "REG_MAC_ANTTUNESEL3"=153, "REG_MAC_ANTTUNESTEP"=154, "REG_MAC_WUMODEBURST"=156, "REG_MAC_WUOFFSHORT"=157, "REG_MAC_WUOFFLONG"=158, "REG_MAC_CLKRECCTRL"=159, "REG_HK_MODE_P2"=162, "REG_MAC_ANTTUNERES1"=164, "REG_MAC_ANTTUNERES2"=165, "REG_INTERFACE_MODE_TEST"=171, "REG_TXRXBUFF_BOTH_P2"=172, "REG_TXRXBUFF_P2"=173, "REG_IRQ_RAWSTATUS1_P2"=174, "REG_MAC_TXIFSTATUS1"=176, "REG_MAC_TXIFSTATUS2"=177, "REG_IRQ_RAWSTATUS2_P2"=178, "REG_MAC_TXIFRAMPDELAY"=179, "REG_MAC_TXIFRAMPSLOPE"=180, "REG_MAX_TXIFRAMP"=181, "REG_IRQ_STATUS1_P2"=182, "REG_IRQ_STATUS2_P2"=183, "REG_IRQ_AUXSTATUS_P2"=184, "REG_MAC_UNLOCK"=188, "REG_MAC_TXIFFREQ"=190, "REG_WAKEUP_TESTCTRL1"=192, "REG_WAKEUP_RX_EN_CNT"=193, "REG_WAKEUP_TESTENABLES"=194, "REG_WAKEUP_DTBI_CTRL"=195, "REG_WAKEUP_DTBO_CTRL"=196, "REG_WAKEUP_TESTIOBUFTEST"=197, "REG_WAKEUP_WK_RX_TESTCTRL1"=198, "REG_WAKEUP_WK_RX_TESTCTRL2"=199, "REG_WAKEUP_SENS_SEQUENCE_CTRL"=200, "REG_WAKEUP_LNABIAS"=201, "REG_WAKEUP_DET_TH_TRIM1"=202, "REG_WAKEUP_LNABIAS_NOM1"=203, "REG_WAKEUP_RX_TSHORT_TRIM1"=204, "REG_WAKEUP_LNABIAS_NOM2"=205, "REG_WAKEUP_RX_TLONG_TRIM1"=206, "REG_WAKEUP_LNA_NEGRTRIM_NOM1"=207, "REG_WAKEUP_RX_TBURST_TRIM1"=208, "REG_WAKEUP_RX_LNA_NEGRTRIM_NOM2"=209, "REG_WAKEUP_RX_BB_G_BW_SEL1"=210, "REG_WAKEUP_WK_RX_DET_IOSTRIM1"=212, "REG_WAKEUP_WK_RX_CTRL2"=214, "REG_WAKEUP_WK_RX_RSSIVOSTRIM"=215, "REG_WAKEUP_LNANEGR_EFF"=216, "REG_WAKEUP_XOSU_FAST"=217, "REG_WAKEUP_STROSCPWIDTH1"=218, "REG_WAKEUP_STROSCPERIOD1"=220, "REG_WAKEUP_STROSCPERIOD2"=221, "REG_WAKEUP_WK_RX_LNA_NEGRTRIM1"=222, "REG_RF_TXTESTENABLE"=224, "REG_RF_TXIFTESTMODE"=225, "REG_RF_RXTESTENABLE"=226, "REG_RF_RXIFTESTCTRL1"=227, "REG_RF_RXIFTESTCTRL2"=228, "REG_RF_RXIFTESTCTRL3"=229, "REG_RF_SYNTH_TESTCTRL1"=230, "REG_RF_SYNTH_TESTCTRL2"=231, "REG_RF_SYNTH_TESTCTRL3"=232, "REG_RF_ADCTEST1"=237, "REG_RF_ADCTEST2"=238, "REG_RF_TXMIXER_IOSTRIM_LOW_IP"=240, "REG_RF_TXMIXER_IOSTRIM_LOW_IN"=241, "REG_RF_TXMIXER_ISOTRIM_LOW_QP"=242, "REG_RF_TXMIXER_IOSTRIM_LOW_QN"=243, "REG_RF_SYNTH_KPD"=244, "REG_RF_SYNTH_LOLEV"=245, "REG_RF_TXRFPWRTUNEANTSET"=246, "REG_RF_TXPD_GAIN_CTRL"=247, "REG_RF_SYNTH_STARTUP"=248, "REG_RF_TXRFANTTUNE_TXMODE"=249, "REG_RF_TXRFANTTUNE_RXMODE"=250, "REG_RF_RXRFANTTUNE_TXMODE"=251, "REG_RF_RXRFANTTUNE_RXMODE"=252, "REG_ANTMATCH1"=253, "REG_ANTMATCH2"=254, "REG_REVISION_P2"=255] ("Register")
  w49 = u16 74 items=["---MANUAL ENTRY---"=1000, "REG_NOREG"=0, "REG_RXBUFF_USED"=1, "REG_RXBUFF_BSIZE"=2, "REG_TXBUFF_USED"=3, "REG_TXBUFF_BSIZE"=4, "REG_TXBUFF_MAXPACKSIZE"=5, "REG_MAC_ERRCLR"=6, "REG_MAC_TRAINNUM"=7, "REG_MAC_SYNCMATCH"=8, "REG_MAC_SYNC1"=9, "REG_MAC_SYNC2"=10, "REG_MAC_SYNC3"=11, "REG_MAC_SYNC4"=12, "REG_MAC_SYNC5"=13, "REG_MAC_MAXBERR"=14, "REG_MAC_ECCORR"=15, "REG_MAC_CRCERR"=16, "REG_MAC_BLKCNT1"=17, "REG_MAC_BLKCNT2"=18, "REG_MAC_IMDTRANSID1"=19, "REG_MAC_IMDTRANSID2"=20, "REG_MAC_IMDTRANSID3"=21, "REG_MAC_COMPANYID"=22, "REG_MAC_MODUSER"=23, "REG_MAC_CHANNEL"=25, "REG_MAC_CLEARWDOG"=26, "REG_MAC_CKCORRTHRESH"=27, "REG_HK_TXADDR"=28, "REG_HK_TXDATA"=29, "REG_HK_TXREPLY"=30, "REG_HK_USERDATA"=31, "REG_HK_USERSTATUS"=32, "REG_HK_LASTADDRESS"=33, "REG_HK_MODE"=34, "REG_MAC_STATUSSEQ"=35, "REG_MAC_MAXRETRIES"=36, "REG_MAC_RESENDTIME"=37, "REG_MAC_POWERSAVETIME"=38, "REG_MAC_HEAD_DET"=39, "REG_MAC_CTRL"=41, "REG_MAC_INITCOM"=42, "REG_INTERFACE_MODE"=43, "REG_TXRXBUFF_BOTH"=44, "REG_TXRXBUFF"=45, "REG_IRQ_RAWSTATUS1"=46, "REG_IRQ_ENABLE1"=47, "REG_IRQ_ENABLESET1"=48, "REG_IRQ_ENABLECLEAR1"=49, "REG_IRQ_RAWSTATUS2"=50, "REG_IRQ_ENABLE2"=51, "REG_IRQ_ENABLESET2"=52, "REG_IRQ_ENABLECLEAR2"=53, "REG_IRQ_STATUS1"=54, "REG_IRQ_STATUS2"=55, "REG_IRQ_AUXSTATUS"=56, "REG_TXBUFF_OVERFLOW"=57, "REG_PO0"=58, "REG_P01"=59, "REG_P02"=60, "REG_P03"=61, "REG_GP0"=62, "REG_GPI"=63, "REG_WAKEUP_245IN"=64, "REG_WAKEUP_COMPANYID"=65, "REG_WAKEUP_IMDTRANSID1"=66, "REG_WAKEUP_IMDTRANSID2"=67, "REG_WAKEUP_IMDTRANSID3"=68, "REG_WAKEUP_CHANNEL"=69, "REG_WAKEUP_MODUSER"=70, "REG_WAKEUP_DEVICEMODE"=71, "REG_WAKEUP_WK_RX_CTRL1"=72, "REG_WAKEUP_STACK_ADDR"=73, "REG_WAKEUP_CTRL"=74, "REG_WAKEUP_STROSCRTRIM"=75, "REG_WAKEUP_BIASTRIM"=76, "REG_WAKEUP_ANT245TUNE"=77, "REG_WAKEUP_WK_RX_RTRIMDET"=78, "REG_WAKEUP_WK_RX_RTRIMDEMOD"=79, "REG_WAKEUP_WK_RX_RSSIGAIN"=80, "REG_WAKEUP_LNAFREQ1"=81, "REG_WAKEUP_STACK"=83, "REG_WAKUP_XOSU"=84, "REG_WAKUP_CNTDROPOUT"=85, "REG_WAKEUP_CRCCTRL"=86, "REG_WAKEUP_CRCWORD1"=87, "REG_WAKEUP_CRCWORD2"=88, "REG_WAKEUP_WK_RX_CTRIM"=89, "REG_WAKEUP_VDDATRIM"=90, "REG_WAKEUP_VDDDTRIM"=91, "REG_WAKEUP_TESTIOBUFEN"=92, "REG_WAKEUP_TESTIOCLAMP"=93, "CORE_RESET_ADDRESS"=94, "CHIP_RESET_ADDRESS"=95, "REG_RF_TXGENCTRL"=96, "REG_RF_TXIFCTRL"=97, "REG_RF_TXRF_SEL_CTRL"=98, "REG_RF_TXRFPWRDEFAULTSET"=99, "REG_RF_RSSITRIM"=100, "REG_RF_TXIFOSCTUNE"=101, "REG_RF_TXIFGAINIMB"=102, "REG_RF_TXIFLOCK"=103, "REG_RF_RXRFLNAGAINTRIM"=104, "REG_RF_RXBIASTR"=105, "REG_RF_RXGENCTRL"=106, "REG_RF_RXIFADCDECLEV"=107, "REG_RF_RXIFDETFILTERTUNE"=108, "REG_RF_RXIFFILTERTUNE"=109, "REG_RF_GENENABLES"=110, "REG_RF_SYNTH_CHANNEL"=111, "REG_TX_RAMP_RTRIM"=112, "REG_TX_RAMP_CTRIM"=113, "REG_RF_XO_TRIM"=114, "REG_RF_SYNTH_SET_TRIM"=115, "REG_RF_ADCCTRL"=116, "REG_RF_ADCOUTPUT"=117, "REG_RF_TXIFAMP"=118, "REG_RF_SYNTH_RTRIM"=119, "REG_RF_SYNTH_CTRIM"=120, "REG_RF_SYNTH_CT"=121, "REG_RF_TXMIXER_IOSTRIM_HIGH_IP"=122, "REG_RF_TXMIXER_IOSTRIM_HIGH_IN"=123, "REG_RF_TXMIXER_IOSTRIM_HIGH_QP"=124, "REG_RF_TXMIXER_IOSTRIM_HIGH_QN"=125, "REG_HX_WUADDR"=126, "REG_REVISION"=127, "REG_NOREG_TEST"=128, "REG_DTEST_RXBUFF"=129, "REG_RXBUFF_NEXT_BLOCK"=130, "REG_RXBUFF_FIRST_IN_PACK"=131, "REG_RXBUFF_FIRST_EMPTY"=132, "REG_MAC_BYPASS"=133, "REG_DTEST_TXBUFF"=134, "REG_TXBUFF_NEXT_BLOCK"=135, "REG_TXBUFF_FIRST_IN_PACK"=136, "REG_TXBUFF_FIRST_EMPTY"=137, "REG_DTEST_SEQ"=138, "REG_DTEST_CKCORR"=139, "REG_MAC_TOPSTATE"=140, "REG_DTEST_INTERFACE"=141, "REG_IFACE_TXRX_BYPASS"=142, "REG_MAC_TXRXWAIT"=143, "REG_MAC_TXRFRAMP"=144, "REG_MAC_TRAINWORD"=145, "REG_MAC_TRAINWORD2"=146, "REG_MAC_SETTINGS"=147, "REG_MAC_CALSELECT1"=148, "REG_MAC_CALSELECT2"=149, "REG_MAC_ANTMATCHSEL"=150, "REG_MAC_ANTTUNESEL1"=151, "REG_MAC_ANTTUNESEL2"=152, "REG_MAC_ANTTUNESEL3"=153, "REG_MAC_ANTTUNESTEP"=154, "REG_MAC_WUMODEBURST"=156, "REG_MAC_WUOFFSHORT"=157, "REG_MAC_WUOFFLONG"=158, "REG_MAC_CLKRECCTRL"=159, "REG_HK_MODE_P2"=162, "REG_MAC_ANTTUNERES1"=164, "REG_MAC_ANTTUNERES2"=165, "REG_INTERFACE_MODE_TEST"=171, "REG_TXRXBUFF_BOTH_P2"=172, "REG_TXRXBUFF_P2"=173, "REG_IRQ_RAWSTATUS1_P2"=174, "REG_MAC_TXIFSTATUS1"=176, "REG_MAC_TXIFSTATUS2"=177, "REG_IRQ_RAWSTATUS2_P2"=178, "REG_MAC_TXIFRAMPDELAY"=179, "REG_MAC_TXIFRAMPSLOPE"=180, "REG_MAX_TXIFRAMP"=181, "REG_IRQ_STATUS1_P2"=182, "REG_IRQ_STATUS2_P2"=183, "REG_IRQ_AUXSTATUS_P2"=184, "REG_MAC_UNLOCK"=188, "REG_MAC_TXIFFREQ"=190, "REG_WAKEUP_TESTCTRL1"=192, "REG_WAKEUP_RX_EN_CNT"=193, "REG_WAKEUP_TESTENABLES"=194, "REG_WAKEUP_DTBI_CTRL"=195, "REG_WAKEUP_DTBO_CTRL"=196, "REG_WAKEUP_TESTIOBUFTEST"=197, "REG_WAKEUP_WK_RX_TESTCTRL1"=198, "REG_WAKEUP_WK_RX_TESTCTRL2"=199, "REG_WAKEUP_SENS_SEQUENCE_CTRL"=200, "REG_WAKEUP_LNABIAS"=201, "REG_WAKEUP_DET_TH_TRIM1"=202, "REG_WAKEUP_LNABIAS_NOM1"=203, "REG_WAKEUP_RX_TSHORT_TRIM1"=204, "REG_WAKEUP_LNABIAS_NOM2"=205, "REG_WAKEUP_RX_TLONG_TRIM1"=206, "REG_WAKEUP_LNA_NEGRTRIM_NOM1"=207, "REG_WAKEUP_RX_TBURST_TRIM1"=208, "REG_WAKEUP_RX_LNA_NEGRTRIM_NOM2"=209, "REG_WAKEUP_RX_BB_G_BW_SEL1"=210, "REG_WAKEUP_WK_RX_DET_IOSTRIM1"=212, "REG_WAKEUP_WK_RX_CTRL2"=214, "REG_WAKEUP_WK_RX_RSSIVOSTRIM"=215, "REG_WAKEUP_LNANEGR_EFF"=216, "REG_WAKEUP_XOSU_FAST"=217, "REG_WAKEUP_STROSCPWIDTH1"=218, "REG_WAKEUP_STROSCPERIOD1"=220, "REG_WAKEUP_STROSCPERIOD2"=221, "REG_WAKEUP_WK_RX_LNA_NEGRTRIM1"=222, "REG_RF_TXTESTENABLE"=224, "REG_RF_TXIFTESTMODE"=225, "REG_RF_RXTESTENABLE"=226, "REG_RF_RXIFTESTCTRL1"=227, "REG_RF_RXIFTESTCTRL2"=228, "REG_RF_RXIFTESTCTRL3"=229, "REG_RF_SYNTH_TESTCTRL1"=230, "REG_RF_SYNTH_TESTCTRL2"=231, "REG_RF_SYNTH_TESTCTRL3"=232, "REG_RF_ADCTEST1"=237, "REG_RF_ADCTEST2"=238, "REG_RF_TXMIXER_IOSTRIM_LOW_IP"=240, "REG_RF_TXMIXER_IOSTRIM_LOW_IN"=241, "REG_RF_TXMIXER_ISOTRIM_LOW_QP"=242, "REG_RF_TXMIXER_IOSTRIM_LOW_QN"=243, "REG_RF_SYNTH_KPD"=244, "REG_RF_SYNTH_LOLEV"=245, "REG_RF_TXRFPWRTUNEANTSET"=246, "REG_RF_TXPD_GAIN_CTRL"=247, "REG_RF_SYNTH_STARTUP"=248, "REG_RF_TXRFANTTUNE_TXMODE"=249, "REG_RF_TXRFANTTUNE_RXMODE"=250, "REG_RF_RXRFANTTUNE_TXMODE"=251, "REG_RF_RXRFANTTUNE_RXMODE"=252, "REG_ANTMATCH1"=253, "REG_ANTMATCH2"=254, "REG_REVISION_P2"=255] ("Register")
  w45 = u16 72 items=["---MANUAL ENTRY---"=1000, "REG_NOREG"=0, "REG_RXBUFF_USED"=1, "REG_RXBUFF_BSIZE"=2, "REG_TXBUFF_USED"=3, "REG_TXBUFF_BSIZE"=4, "REG_TXBUFF_MAXPACKSIZE"=5, "REG_MAC_ERRCLR"=6, "REG_MAC_TRAINNUM"=7, "REG_MAC_SYNCMATCH"=8, "REG_MAC_SYNC1"=9, "REG_MAC_SYNC2"=10, "REG_MAC_SYNC3"=11, "REG_MAC_SYNC4"=12, "REG_MAC_SYNC5"=13, "REG_MAC_MAXBERR"=14, "REG_MAC_ECCORR"=15, "REG_MAC_CRCERR"=16, "REG_MAC_BLKCNT1"=17, "REG_MAC_BLKCNT2"=18, "REG_MAC_IMDTRANSID1"=19, "REG_MAC_IMDTRANSID2"=20, "REG_MAC_IMDTRANSID3"=21, "REG_MAC_COMPANYID"=22, "REG_MAC_MODUSER"=23, "REG_MAC_CHANNEL"=25, "REG_MAC_CLEARWDOG"=26, "REG_MAC_CKCORRTHRESH"=27, "REG_HK_TXADDR"=28, "REG_HK_TXDATA"=29, "REG_HK_TXREPLY"=30, "REG_HK_USERDATA"=31, "REG_HK_USERSTATUS"=32, "REG_HK_LASTADDRESS"=33, "REG_HK_MODE"=34, "REG_MAC_STATUSSEQ"=35, "REG_MAC_MAXRETRIES"=36, "REG_MAC_RESENDTIME"=37, "REG_MAC_POWERSAVETIME"=38, "REG_MAC_HEAD_DET"=39, "REG_MAC_CTRL"=41, "REG_MAC_INITCOM"=42, "REG_INTERFACE_MODE"=43, "REG_TXRXBUFF_BOTH"=44, "REG_TXRXBUFF"=45, "REG_IRQ_RAWSTATUS1"=46, "REG_IRQ_ENABLE1"=47, "REG_IRQ_ENABLESET1"=48, "REG_IRQ_ENABLECLEAR1"=49, "REG_IRQ_RAWSTATUS2"=50, "REG_IRQ_ENABLE2"=51, "REG_IRQ_ENABLESET2"=52, "REG_IRQ_ENABLECLEAR2"=53, "REG_IRQ_STATUS1"=54, "REG_IRQ_STATUS2"=55, "REG_IRQ_AUXSTATUS"=56, "REG_TXBUFF_OVERFLOW"=57, "REG_PO0"=58, "REG_P01"=59, "REG_P02"=60, "REG_P03"=61, "REG_GP0"=62, "REG_GPI"=63, "REG_WAKEUP_245IN"=64, "REG_WAKEUP_COMPANYID"=65, "REG_WAKEUP_IMDTRANSID1"=66, "REG_WAKEUP_IMDTRANSID2"=67, "REG_WAKEUP_IMDTRANSID3"=68, "REG_WAKEUP_CHANNEL"=69, "REG_WAKEUP_MODUSER"=70, "REG_WAKEUP_DEVICEMODE"=71, "REG_WAKEUP_WK_RX_CTRL1"=72, "REG_WAKEUP_STACK_ADDR"=73, "REG_WAKEUP_CTRL"=74, "REG_WAKEUP_STROSCRTRIM"=75, "REG_WAKEUP_BIASTRIM"=76, "REG_WAKEUP_ANT245TUNE"=77, "REG_WAKEUP_WK_RX_RTRIMDET"=78, "REG_WAKEUP_WK_RX_RTRIMDEMOD"=79, "REG_WAKEUP_WK_RX_RSSIGAIN"=80, "REG_WAKEUP_LNAFREQ1"=81, "REG_WAKEUP_STACK"=83, "REG_WAKUP_XOSU"=84, "REG_WAKUP_CNTDROPOUT"=85, "REG_WAKEUP_CRCCTRL"=86, "REG_WAKEUP_CRCWORD1"=87, "REG_WAKEUP_CRCWORD2"=88, "REG_WAKEUP_WK_RX_CTRIM"=89, "REG_WAKEUP_VDDATRIM"=90, "REG_WAKEUP_VDDDTRIM"=91, "REG_WAKEUP_TESTIOBUFEN"=92, "REG_WAKEUP_TESTIOCLAMP"=93, "CORE_RESET_ADDRESS"=94, "CHIP_RESET_ADDRESS"=95, "REG_RF_TXGENCTRL"=96, "REG_RF_TXIFCTRL"=97, "REG_RF_TXRF_SEL_CTRL"=98, "REG_RF_TXRFPWRDEFAULTSET"=99, "REG_RF_RSSITRIM"=100, "REG_RF_TXIFOSCTUNE"=101, "REG_RF_TXIFGAINIMB"=102, "REG_RF_TXIFLOCK"=103, "REG_RF_RXRFLNAGAINTRIM"=104, "REG_RF_RXBIASTR"=105, "REG_RF_RXGENCTRL"=106, "REG_RF_RXIFADCDECLEV"=107, "REG_RF_RXIFDETFILTERTUNE"=108, "REG_RF_RXIFFILTERTUNE"=109, "REG_RF_GENENABLES"=110, "REG_RF_SYNTH_CHANNEL"=111, "REG_TX_RAMP_RTRIM"=112, "REG_TX_RAMP_CTRIM"=113, "REG_RF_XO_TRIM"=114, "REG_RF_SYNTH_SET_TRIM"=115, "REG_RF_ADCCTRL"=116, "REG_RF_ADCOUTPUT"=117, "REG_RF_TXIFAMP"=118, "REG_RF_SYNTH_RTRIM"=119, "REG_RF_SYNTH_CTRIM"=120, "REG_RF_SYNTH_CT"=121, "REG_RF_TXMIXER_IOSTRIM_HIGH_IP"=122, "REG_RF_TXMIXER_IOSTRIM_HIGH_IN"=123, "REG_RF_TXMIXER_IOSTRIM_HIGH_QP"=124, "REG_RF_TXMIXER_IOSTRIM_HIGH_QN"=125, "REG_HX_WUADDR"=126, "REG_REVISION"=127, "REG_NOREG_TEST"=128, "REG_DTEST_RXBUFF"=129, "REG_RXBUFF_NEXT_BLOCK"=130, "REG_RXBUFF_FIRST_IN_PACK"=131, "REG_RXBUFF_FIRST_EMPTY"=132, "REG_MAC_BYPASS"=133, "REG_DTEST_TXBUFF"=134, "REG_TXBUFF_NEXT_BLOCK"=135, "REG_TXBUFF_FIRST_IN_PACK"=136, "REG_TXBUFF_FIRST_EMPTY"=137, "REG_DTEST_SEQ"=138, "REG_DTEST_CKCORR"=139, "REG_MAC_TOPSTATE"=140, "REG_DTEST_INTERFACE"=141, "REG_IFACE_TXRX_BYPASS"=142, "REG_MAC_TXRXWAIT"=143, "REG_MAC_TXRFRAMP"=144, "REG_MAC_TRAINWORD"=145, "REG_MAC_TRAINWORD2"=146, "REG_MAC_SETTINGS"=147, "REG_MAC_CALSELECT1"=148, "REG_MAC_CALSELECT2"=149, "REG_MAC_ANTMATCHSEL"=150, "REG_MAC_ANTTUNESEL1"=151, "REG_MAC_ANTTUNESEL2"=152, "REG_MAC_ANTTUNESEL3"=153, "REG_MAC_ANTTUNESTEP"=154, "REG_MAC_WUMODEBURST"=156, "REG_MAC_WUOFFSHORT"=157, "REG_MAC_WUOFFLONG"=158, "REG_MAC_CLKRECCTRL"=159, "REG_HK_MODE_P2"=162, "REG_MAC_ANTTUNERES1"=164, "REG_MAC_ANTTUNERES2"=165, "REG_INTERFACE_MODE_TEST"=171, "REG_TXRXBUFF_BOTH_P2"=172, "REG_TXRXBUFF_P2"=173, "REG_IRQ_RAWSTATUS1_P2"=174, "REG_MAC_TXIFSTATUS1"=176, "REG_MAC_TXIFSTATUS2"=177, "REG_IRQ_RAWSTATUS2_P2"=178, "REG_MAC_TXIFRAMPDELAY"=179, "REG_MAC_TXIFRAMPSLOPE"=180, "REG_MAX_TXIFRAMP"=181, "REG_IRQ_STATUS1_P2"=182, "REG_IRQ_STATUS2_P2"=183, "REG_IRQ_AUXSTATUS_P2"=184, "REG_MAC_UNLOCK"=188, "REG_MAC_TXIFFREQ"=190, "REG_WAKEUP_TESTCTRL1"=192, "REG_WAKEUP_RX_EN_CNT"=193, "REG_WAKEUP_TESTENABLES"=194, "REG_WAKEUP_DTBI_CTRL"=195, "REG_WAKEUP_DTBO_CTRL"=196, "REG_WAKEUP_TESTIOBUFTEST"=197, "REG_WAKEUP_WK_RX_TESTCTRL1"=198, "REG_WAKEUP_WK_RX_TESTCTRL2"=199, "REG_WAKEUP_SENS_SEQUENCE_CTRL"=200, "REG_WAKEUP_LNABIAS"=201, "REG_WAKEUP_DET_TH_TRIM1"=202, "REG_WAKEUP_LNABIAS_NOM1"=203, "REG_WAKEUP_RX_TSHORT_TRIM1"=204, "REG_WAKEUP_LNABIAS_NOM2"=205, "REG_WAKEUP_RX_TLONG_TRIM1"=206, "REG_WAKEUP_LNA_NEGRTRIM_NOM1"=207, "REG_WAKEUP_RX_TBURST_TRIM1"=208, "REG_WAKEUP_RX_LNA_NEGRTRIM_NOM2"=209, "REG_WAKEUP_RX_BB_G_BW_SEL1"=210, "REG_WAKEUP_WK_RX_DET_IOSTRIM1"=212, "REG_WAKEUP_WK_RX_CTRL2"=214, "REG_WAKEUP_WK_RX_RSSIVOSTRIM"=215, "REG_WAKEUP_LNANEGR_EFF"=216, "REG_WAKEUP_XOSU_FAST"=217, "REG_WAKEUP_STROSCPWIDTH1"=218, "REG_WAKEUP_STROSCPERIOD1"=220, "REG_WAKEUP_STROSCPERIOD2"=221, "REG_WAKEUP_WK_RX_LNA_NEGRTRIM1"=222, "REG_RF_TXTESTENABLE"=224, "REG_RF_TXIFTESTMODE"=225, "REG_RF_RXTESTENABLE"=226, "REG_RF_RXIFTESTCTRL1"=227, "REG_RF_RXIFTESTCTRL2"=228, "REG_RF_RXIFTESTCTRL3"=229, "REG_RF_SYNTH_TESTCTRL1"=230, "REG_RF_SYNTH_TESTCTRL2"=231, "REG_RF_SYNTH_TESTCTRL3"=232, "REG_RF_ADCTEST1"=237, "REG_RF_ADCTEST2"=238, "REG_RF_TXMIXER_IOSTRIM_LOW_IP"=240, "REG_RF_TXMIXER_IOSTRIM_LOW_IN"=241, "REG_RF_TXMIXER_ISOTRIM_LOW_QP"=242, "REG_RF_TXMIXER_IOSTRIM_LOW_QN"=243, "REG_RF_SYNTH_KPD"=244, "REG_RF_SYNTH_LOLEV"=245, "REG_RF_TXRFPWRTUNEANTSET"=246, "REG_RF_TXPD_GAIN_CTRL"=247, "REG_RF_SYNTH_STARTUP"=248, "REG_RF_TXRFANTTUNE_TXMODE"=249, "REG_RF_TXRFANTTUNE_RXMODE"=250, "REG_RF_RXRFANTTUNE_TXMODE"=251, "REG_RF_RXRFANTTUNE_RXMODE"=252, "REG_ANTMATCH1"=253, "REG_ANTMATCH2"=254, "REG_REVISION_P2"=255] ("Register")
  w47 = u16 198 items=["---MANUAL ENTRY---"=1000, "REG_NOREG"=0, "REG_RXBUFF_USED"=1, "REG_RXBUFF_BSIZE"=2, "REG_TXBUFF_USED"=3, "REG_TXBUFF_BSIZE"=4, "REG_TXBUFF_MAXPACKSIZE"=5, "REG_MAC_ERRCLR"=6, "REG_MAC_TRAINNUM"=7, "REG_MAC_SYNCMATCH"=8, "REG_MAC_SYNC1"=9, "REG_MAC_SYNC2"=10, "REG_MAC_SYNC3"=11, "REG_MAC_SYNC4"=12, "REG_MAC_SYNC5"=13, "REG_MAC_MAXBERR"=14, "REG_MAC_ECCORR"=15, "REG_MAC_CRCERR"=16, "REG_MAC_BLKCNT1"=17, "REG_MAC_BLKCNT2"=18, "REG_MAC_IMDTRANSID1"=19, "REG_MAC_IMDTRANSID2"=20, "REG_MAC_IMDTRANSID3"=21, "REG_MAC_COMPANYID"=22, "REG_MAC_MODUSER"=23, "REG_MAC_CHANNEL"=25, "REG_MAC_CLEARWDOG"=26, "REG_MAC_CKCORRTHRESH"=27, "REG_HK_TXADDR"=28, "REG_HK_TXDATA"=29, "REG_HK_TXREPLY"=30, "REG_HK_USERDATA"=31, "REG_HK_USERSTATUS"=32, "REG_HK_LASTADDRESS"=33, "REG_HK_MODE"=34, "REG_MAC_STATUSSEQ"=35, "REG_MAC_MAXRETRIES"=36, "REG_MAC_RESENDTIME"=37, "REG_MAC_POWERSAVETIME"=38, "REG_MAC_HEAD_DET"=39, "REG_MAC_CTRL"=41, "REG_MAC_INITCOM"=42, "REG_INTERFACE_MODE"=43, "REG_TXRXBUFF_BOTH"=44, "REG_TXRXBUFF"=45, "REG_IRQ_RAWSTATUS1"=46, "REG_IRQ_ENABLE1"=47, "REG_IRQ_ENABLESET1"=48, "REG_IRQ_ENABLECLEAR1"=49, "REG_IRQ_RAWSTATUS2"=50, "REG_IRQ_ENABLE2"=51, "REG_IRQ_ENABLESET2"=52, "REG_IRQ_ENABLECLEAR2"=53, "REG_IRQ_STATUS1"=54, "REG_IRQ_STATUS2"=55, "REG_IRQ_AUXSTATUS"=56, "REG_TXBUFF_OVERFLOW"=57, "REG_PO0"=58, "REG_P01"=59, "REG_P02"=60, "REG_P03"=61, "REG_GP0"=62, "REG_GPI"=63, "REG_WAKEUP_245IN"=64, "REG_WAKEUP_COMPANYID"=65, "REG_WAKEUP_IMDTRANSID1"=66, "REG_WAKEUP_IMDTRANSID2"=67, "REG_WAKEUP_IMDTRANSID3"=68, "REG_WAKEUP_CHANNEL"=69, "REG_WAKEUP_MODUSER"=70, "REG_WAKEUP_DEVICEMODE"=71, "REG_WAKEUP_WK_RX_CTRL1"=72, "REG_WAKEUP_STACK_ADDR"=73, "REG_WAKEUP_CTRL"=74, "REG_WAKEUP_STROSCRTRIM"=75, "REG_WAKEUP_BIASTRIM"=76, "REG_WAKEUP_ANT245TUNE"=77, "REG_WAKEUP_WK_RX_RTRIMDET"=78, "REG_WAKEUP_WK_RX_RTRIMDEMOD"=79, "REG_WAKEUP_WK_RX_RSSIGAIN"=80, "REG_WAKEUP_LNAFREQ1"=81, "REG_WAKEUP_STACK"=83, "REG_WAKUP_XOSU"=84, "REG_WAKUP_CNTDROPOUT"=85, "REG_WAKEUP_CRCCTRL"=86, "REG_WAKEUP_CRCWORD1"=87, "REG_WAKEUP_CRCWORD2"=88, "REG_WAKEUP_WK_RX_CTRIM"=89, "REG_WAKEUP_VDDATRIM"=90, "REG_WAKEUP_VDDDTRIM"=91, "REG_WAKEUP_TESTIOBUFEN"=92, "REG_WAKEUP_TESTIOCLAMP"=93, "CORE_RESET_ADDRESS"=94, "CHIP_RESET_ADDRESS"=95, "REG_RF_TXGENCTRL"=96, "REG_RF_TXIFCTRL"=97, "REG_RF_TXRF_SEL_CTRL"=98, "REG_RF_TXRFPWRDEFAULTSET"=99, "REG_RF_RSSITRIM"=100, "REG_RF_TXIFOSCTUNE"=101, "REG_RF_TXIFGAINIMB"=102, "REG_RF_TXIFLOCK"=103, "REG_RF_RXRFLNAGAINTRIM"=104, "REG_RF_RXBIASTR"=105, "REG_RF_RXGENCTRL"=106, "REG_RF_RXIFADCDECLEV"=107, "REG_RF_RXIFDETFILTERTUNE"=108, "REG_RF_RXIFFILTERTUNE"=109, "REG_RF_GENENABLES"=110, "REG_RF_SYNTH_CHANNEL"=111, "REG_TX_RAMP_RTRIM"=112, "REG_TX_RAMP_CTRIM"=113, "REG_RF_XO_TRIM"=114, "REG_RF_SYNTH_SET_TRIM"=115, "REG_RF_ADCCTRL"=116, "REG_RF_ADCOUTPUT"=117, "REG_RF_TXIFAMP"=118, "REG_RF_SYNTH_RTRIM"=119, "REG_RF_SYNTH_CTRIM"=120, "REG_RF_SYNTH_CT"=121, "REG_RF_TXMIXER_IOSTRIM_HIGH_IP"=122, "REG_RF_TXMIXER_IOSTRIM_HIGH_IN"=123, "REG_RF_TXMIXER_IOSTRIM_HIGH_QP"=124, "REG_RF_TXMIXER_IOSTRIM_HIGH_QN"=125, "REG_HX_WUADDR"=126, "REG_REVISION"=127, "REG_NOREG_TEST"=128, "REG_DTEST_RXBUFF"=129, "REG_RXBUFF_NEXT_BLOCK"=130, "REG_RXBUFF_FIRST_IN_PACK"=131, "REG_RXBUFF_FIRST_EMPTY"=132, "REG_MAC_BYPASS"=133, "REG_DTEST_TXBUFF"=134, "REG_TXBUFF_NEXT_BLOCK"=135, "REG_TXBUFF_FIRST_IN_PACK"=136, "REG_TXBUFF_FIRST_EMPTY"=137, "REG_DTEST_SEQ"=138, "REG_DTEST_CKCORR"=139, "REG_MAC_TOPSTATE"=140, "REG_DTEST_INTERFACE"=141, "REG_IFACE_TXRX_BYPASS"=142, "REG_MAC_TXRXWAIT"=143, "REG_MAC_TXRFRAMP"=144, "REG_MAC_TRAINWORD"=145, "REG_MAC_TRAINWORD2"=146, "REG_MAC_SETTINGS"=147, "REG_MAC_CALSELECT1"=148, "REG_MAC_CALSELECT2"=149, "REG_MAC_ANTMATCHSEL"=150, "REG_MAC_ANTTUNESEL1"=151, "REG_MAC_ANTTUNESEL2"=152, "REG_MAC_ANTTUNESEL3"=153, "REG_MAC_ANTTUNESTEP"=154, "REG_MAC_WUMODEBURST"=156, "REG_MAC_WUOFFSHORT"=157, "REG_MAC_WUOFFLONG"=158, "REG_MAC_CLKRECCTRL"=159, "REG_HK_MODE_P2"=162, "REG_MAC_ANTTUNERES1"=164, "REG_MAC_ANTTUNERES2"=165, "REG_INTERFACE_MODE_TEST"=171, "REG_TXRXBUFF_BOTH_P2"=172, "REG_TXRXBUFF_P2"=173, "REG_IRQ_RAWSTATUS1_P2"=174, "REG_MAC_TXIFSTATUS1"=176, "REG_MAC_TXIFSTATUS2"=177, "REG_IRQ_RAWSTATUS2_P2"=178, "REG_MAC_TXIFRAMPDELAY"=179, "REG_MAC_TXIFRAMPSLOPE"=180, "REG_MAX_TXIFRAMP"=181, "REG_IRQ_STATUS1_P2"=182, "REG_IRQ_STATUS2_P2"=183, "REG_IRQ_AUXSTATUS_P2"=184, "REG_MAC_UNLOCK"=188, "REG_MAC_TXIFFREQ"=190, "REG_WAKEUP_TESTCTRL1"=192, "REG_WAKEUP_RX_EN_CNT"=193, "REG_WAKEUP_TESTENABLES"=194, "REG_WAKEUP_DTBI_CTRL"=195, "REG_WAKEUP_DTBO_CTRL"=196, "REG_WAKEUP_TESTIOBUFTEST"=197, "REG_WAKEUP_WK_RX_TESTCTRL1"=198, "REG_WAKEUP_WK_RX_TESTCTRL2"=199, "REG_WAKEUP_SENS_SEQUENCE_CTRL"=200, "REG_WAKEUP_LNABIAS"=201, "REG_WAKEUP_DET_TH_TRIM1"=202, "REG_WAKEUP_LNABIAS_NOM1"=203, "REG_WAKEUP_RX_TSHORT_TRIM1"=204, "REG_WAKEUP_LNABIAS_NOM2"=205, "REG_WAKEUP_RX_TLONG_TRIM1"=206, "REG_WAKEUP_LNA_NEGRTRIM_NOM1"=207, "REG_WAKEUP_RX_TBURST_TRIM1"=208, "REG_WAKEUP_RX_LNA_NEGRTRIM_NOM2"=209, "REG_WAKEUP_RX_BB_G_BW_SEL1"=210, "REG_WAKEUP_WK_RX_DET_IOSTRIM1"=212, "REG_WAKEUP_WK_RX_CTRL2"=214, "REG_WAKEUP_WK_RX_RSSIVOSTRIM"=215, "REG_WAKEUP_LNANEGR_EFF"=216, "REG_WAKEUP_XOSU_FAST"=217, "REG_WAKEUP_STROSCPWIDTH1"=218, "REG_WAKEUP_STROSCPERIOD1"=220, "REG_WAKEUP_STROSCPERIOD2"=221, "REG_WAKEUP_WK_RX_LNA_NEGRTRIM1"=222, "REG_RF_TXTESTENABLE"=224, "REG_RF_TXIFTESTMODE"=225, "REG_RF_RXTESTENABLE"=226, "REG_RF_RXIFTESTCTRL1"=227, "REG_RF_RXIFTESTCTRL2"=228, "REG_RF_RXIFTESTCTRL3"=229, "REG_RF_SYNTH_TESTCTRL1"=230, "REG_RF_SYNTH_TESTCTRL2"=231, "REG_RF_SYNTH_TESTCTRL3"=232, "REG_RF_ADCTEST1"=237, "REG_RF_ADCTEST2"=238, "REG_RF_TXMIXER_IOSTRIM_LOW_IP"=240, "REG_RF_TXMIXER_IOSTRIM_LOW_IN"=241, "REG_RF_TXMIXER_ISOTRIM_LOW_QP"=242, "REG_RF_TXMIXER_IOSTRIM_LOW_QN"=243, "REG_RF_SYNTH_KPD"=244, "REG_RF_SYNTH_LOLEV"=245, "REG_RF_TXRFPWRTUNEANTSET"=246, "REG_RF_TXPD_GAIN_CTRL"=247, "REG_RF_SYNTH_STARTUP"=248, "REG_RF_TXRFANTTUNE_TXMODE"=249, "REG_RF_TXRFANTTUNE_RXMODE"=250, "REG_RF_RXRFANTTUNE_TXMODE"=251, "REG_RF_RXRFANTTUNE_RXMODE"=252, "REG_ANTMATCH1"=253, "REG_ANTMATCH2"=254, "REG_REVISION_P2"=255] ("Register")
  w1 = FALSE
  w22 = u8 0
  # "Initialize the \nregisters used\nfor testing"
  # "Disable DSC"
  # "Disable \"Wakeup toggle\""
  # "Disable Wakeup Test Registers"
  # "Enable RSSI, Wakeup LNA, Detector"
  # "Enable Wakeup Test Registers"
  n1 = flat-sequence {
    tunnel: "error in (no error)" -> [w68]
    tunnel: [w68] -> w40
    frame #0 {
      n2 = local write "Wakeup Signal Power, dBm"(-32.0 ("Wakeup Signal Power, dBm")) -> ()
      n3 = local write "Wakeup Signal Transmit"(FALSE ("Wakeup Signal Transmit")) -> ()
      n4 = local write "Update Radio Settings"(FALSE ("Update Radio Settings")) -> ()
      n5 = local write "Samples to Average"(u8 5 ("Samples to Average")) -> ()
      n6 = local write "Detector Offset Trim"(u8 32 ("Detector Theshold")) -> ()
      n7 = local write "LNA Frequency Trim"(u8 15 ("LNA Frequency Trim")) -> ()
      n8 = local write "Loopback Detector"(FALSE ("Loopback Detector")) -> ()
      n9 = local write "RX Antenna Tune"(u8 7 ("RX Antenna Tune")) -> ()
      n10 = local write "RSSI Fine Trim"(u8 15 ("Baseband Gain")) -> ()
      n11 = local write "LNA Gain Trim"(u8 20 ("LNA Gain Trim")) -> ()
      n12 = local write "Do RSSI"(FALSE ("Do RSSI")) -> ()
    }
  }
  n13 = call "JTAG Init.vi"("error in (no error)"=w40, "Power Target Device"=TRUE) -> ("error out"=w37:errorcluster, "Device Vcc"=→"Device Vcc":i32)  [unwired: 8 in]
  n14 = call "JTAG Config.vi"("error in (no error)"=w37, "Function"=w35) -> ("error out"=w36:errorcluster)  [unwired: 9 in]
  n15 = call "JTAG Base Function.vi"("Function"=w42, "error in (no error)"=w36) -> ("error out"=w26:errorcluster)  [unwired: 11 in, 2 out]
  n16 = call "Simple Wait.vi"("mS"=u32 200, "error in"=w26) -> ("error out"=w25:errorcluster)  [unwired: 12 in, 1 out]
  n17 = call "JTAG Base Function.vi"("Function"=w41, "error in (no error)"=w25) -> ("error out"=w23:errorcluster)  [unwired: 11 in, 2 out]
  n18 = call "Simple Wait.vi"("mS"=u32 200, "error in"=w23) -> ("error out"=w21:errorcluster)  [unwired: 12 in, 1 out]
  n19 = call "JTAG SPI.vi"("Value"=u8 187 ("Data"), "error in (no error)"=w21, "Target"=w20, "Function"=w19, "Address"=w18) -> ("error out"=w10:errorcluster)  [unwired: 3 in, 3 out]
  n20 = call "JTAG SPI.vi"("Value"=u8 0 ("Data"), "error in (no error)"=w10, "Address"=w16) -> ("error out"=w9:errorcluster)  [unwired: 5 in, 3 out]
  n21 = call "JTAG SPI.vi"("Value"=u8 0 ("Data"), "error in (no error)"=w9, "Address"=w14) -> ("error out"=w8:errorcluster)  [unwired: 5 in, 3 out]
  n22 = call "JTAG SPI.vi"("Value"=u8 16 ("Data"), "error in (no error)"=w8, "Address"=w12) -> ("error out"=w7:errorcluster)  [unwired: 5 in, 3 out]
  n23 = call "JTAG SPI.vi"("Value"=u8 129 ("Data"), "error in (no error)"=w7, "Target"=w20, "Function"=w19, "Address"=w59) -> ("error out"=w57:errorcluster)  [unwired: 3 in, 3 out]
  n24 = call "JTAG SPI.vi"("Value"=u8 0 ("Data"), "error in (no error)"=w57, "Target"=w20, "Function"=w19, "Address"=w56) -> ("error out"=w53:errorcluster)  [unwired: 3 in, 3 out]
  n25 = call "JTAG SPI.vi"("error in (no error)"=w53, "Target"=w20, "Function"=w54, "Address"=w49) -> ("error out"=w52:errorcluster, "Read Value"=w50:u8)  [unwired: 4 in, 2 out]
  n26 = Or(x=u8 72 ("Data"), y=w50) -> (x .or. y?=w51:u8)
  n27 = call "JTAG SPI.vi"("Value"=w51, "error in (no error)"=w52, "Target"=w20, "Function"=w19, "Address"=w49) -> ("error out"=w48:errorcluster)  [unwired: 3 in, 3 out]
  n28 = call "JTAG SPI.vi"("Value"=u8 1 ("Data"), "error in (no error)"=w48, "Target"=w20, "Function"=w19, "Address"=w47) -> ("error out"=w44:errorcluster)  [unwired: 3 in, 3 out]
  n29 = Select(t=u8 15 ("Data"), s="DetTrim", f=u8 13 ("Data")) -> (s? t:f=w43:u8)
  n30 = call "JTAG SPI.vi"("Value"=w43, "error in (no error)"=w44, "Target"=w20, "Function"=w19, "Address"=w45) -> ("error out"=w5:errorcluster)  [unwired: 3 in, 3 out]
  n31 = call-poly "VISA Configure Serial Port"("VISA resource name"="MICS Dongle Address", "Enable Termination\nChar (T)"=FALSE ("Enable Termination\nChar (T)"), "baud rate (9600)"=u32 225000, "error in (no error)"=w5) -> ("VISA resource name out"=w6:refnum<visa-resource-name>, "error out"=w4:errorcluster)  [unwired: 10 in]
  n32 = while {
    shift-right: [w90] -> w33
    shift-left: w4 -> [w94]
    tunnel: w6 -> [w110]
    shift-right: [w103] -> _
    shift-left: w22 -> [w108]
    shift-right: [w102] -> _
    shift-left: w22 -> [w107]
    shift-right: [w101] -> _
    shift-left: w22 -> [w106]
    shift-right: [w100] -> _
    shift-left: w22 -> [w105]
    shift-right: [w99] -> _
    shift-left: w22 -> [w104]
    shift-right: [w98] -> _
    shift-left: 0.0 -> [w109]
    shift-right: [w95] -> _
    shift-left: w1 -> [w96]
    shift-right: [w92] -> _
    shift-left: w1 -> [w93]
    tunnel: T1 {"ConfigFlags"=0, "ImplantID"=1048576, "CompanyID"=187, "Normal_Comm"={"RF_Channel"=4, "UserData"=80, "TX_Mod"=0, "RX_Mod"=0, "RX_BlockSize"=15, "BlockPerPack"=31, "TX_BlockSize"=15}, "Emerg_Comm"={"RF_Channel"=4, "UserData"=16, "TX_Mod"=0, "RX_Mod"=0, "TX_BlockSize"=15, "BlockPerPack"=31, "RX_BlockSize"=15}, "ImplantRev"=4, "245TX_PowerCal"=0, "245TX_Power"=10, "CCA_RSSI_Thresholds"={"ch0"=2650, "ch1"=2650, "ch2"=2650, "ch3"=2650, "ch4"=2650, "ch5"=2650, "ch6"=2650, "ch7"=2650, "ch8"=2650, "ch9"=2650}} ("MICS_Config_In") -> [w91]
    tunnel: "DetTrim" -> [w86]
    tunnel: w19 -> [w85]
    tunnel: w20 -> [w84]
    shift-right: [w82] -> _
    shift-left: w22 -> [w83]
    shift-right: [w80] -> _
    shift-left: w1 -> [w81]
    stop <- w89 stop-if-true
    # "Loopback Change?"
    # "RSSI Gain"
    # "RF CW Change?"
    # "Radio Val Change?"
    # "Wakeup RF PWR"
    # "RSSI Fine Trim"
    # "RX Ant Tune"
    # "LNA Gain Trim"
    # "Detector Offset"
    # "LNA Freq Trim"
    n33 = Wait (ms)(milliseconds to wait=u32 100) -> ()  [unwired: 1 out]
    n34 = for {
      N: 6 -> [_]
      shift-right: [w137] -> w90
      shift-left: w94 -> [w138]
      tunnel: w110 -> [w136]
      shift-right: [w130] -> w103
      shift-left: w108 -> [w135]
      shift-right: [w129] -> w102
      shift-left: w107 -> [w134]
      shift-right: [w128] -> w101
      shift-left: w106 -> [w133]
      shift-right: [w127] -> w100
      shift-left: w105 -> [w132]
      shift-right: [w126] -> w99
      shift-left: w104 -> [w131]
      shift-right: [w124] -> w98
      shift-left: w109 -> [w125]
      tunnel: w91 -> [w119]
      shift-right: [w122] -> w95
      shift-left: w96 -> [w123]
      shift-right: [w120] -> w92
      shift-left: w93 -> [w121]
      tunnel: w86 -> [w118]
      tunnel: w85 -> [w117]
      tunnel: w84 -> [w116]
      shift-right: [w114] -> w82
      shift-left: w83 -> [w115]
      shift-right: [w112] -> w80
      shift-left: w81 -> [w113]
      i -> [w139]
      n35 = case shown="5" w139 {
        tunnel: w138 -> [w162 w181 w289 w344 w398 w401]
        tunnel: [w162 w179 w278 w343 w398 w404] -> w137
        tunnel: w136 -> [_ _ w288 _ _ _]
        tunnel: w135 -> [w161 w178 w297 w353 w393 w410]
        tunnel: w134 -> [w159 w177 w296 w352 w390 w407]
        tunnel: w133 -> [w157 w176 w295 w351 w392 w409]
        tunnel: w132 -> [w155 w175 w294 w350 w391 w408]
        tunnel: w131 -> [w154 w174 w293 w349 w388 w406]
        tunnel: ["LNA Frequency Trim" w178 w297 w353 w393 w410] -> w130
        tunnel: ["Detector Offset Trim" w177 w296 w352 w390 w407] -> w129
        tunnel: ["LNA Gain Trim" w176 w295 w351 w392 w409] -> w128
        tunnel: ["RX Antenna Tune" w175 w294 w350 w391 w408] -> w127
        tunnel: ["RSSI Fine Trim" w174 w293 w349 w388 w406] -> w126
        tunnel: w125 -> [w144 w173 w281 w348 w395 w411]
        tunnel: [w144 w173 "Wakeup Signal Power, dBm" w348 w395 w411] -> w124
        tunnel: w123 -> [_ w171 w292 w347 w396 w412]
        tunnel: [w151 w180 w292 w347 w396 w412] -> w122
        tunnel: w121 -> [w145 w169 w291 w346 w397 w413]
        tunnel: [w145 w168 "Wakeup Signal Transmit" w346 w397 w413] -> w120
        tunnel: w119 -> [_ _ w282 _ _ _]
        tunnel: w118 -> [_ w167 _ _ _ _]
        tunnel: w117 -> [_ w166 _ w341 _ _]
        tunnel: w116 -> [_ w165 _ w340 _ _]
        tunnel: w115 -> [w143 w164 w277 w339 w387 w405]
        tunnel: ["RSSI Gain" w164 w277 w339 w387 w405] -> w114
        tunnel: w113 -> [w140 w163 w276 w338 w386 w403]
        tunnel: [w140 w163 w276 w338 w386 "Loopback Detector"] -> w112
        frame 0, Default {
          # "Check for Control Changes"
          n36 = Not Equal?(x=w143, y="RSSI Gain") -> (x != y?=w141:bool)
          n37 = Not Equal?(x=w161, y="LNA Frequency Trim") -> (x != y?=w146:bool)
          n38 = Not Equal?(x=w159, y="Detector Offset Trim") -> (x != y?=w147:bool)
          n39 = Not Equal?(x=w157, y="LNA Gain Trim") -> (x != y?=w148:bool)
          n40 = Not Equal?(x=w155, y="RX Antenna Tune") -> (x != y?=w149:bool)
          n41 = Not Equal?(x=w154, y="RSSI Fine Trim") -> (x != y?=w150:bool)
          n42 = Compound Arithmetic op=OR(w141, w146, w147, w148, w149, w150) -> (w151:bool)
        }
        frame 1 {
          # "Apply Control Changes (If Enabled)"
          n43 = And(x=w171, y="Update Radio Settings") -> (x .and. y?=w170:bool)
          n44 = case shown="True" w170 {
            tunnel: w181 -> [w183 w212]
            tunnel: w171 -> [w184 _]
            tunnel: [w184 FALSE] -> w180
            tunnel: [w183 w192] -> w179
            tunnel: w178 -> [_ w207]
            tunnel: w177 -> [_ w208]
            tunnel: w176 -> [_ w209]
            tunnel: w175 -> [_ w210]
            tunnel: w174 -> [_ w211]
            tunnel: w169 -> [w182 w206]
            tunnel: [w182 w206] -> w168
            tunnel: w167 -> [_ w198]
            tunnel: w166 -> [_ w197]
            tunnel: w165 -> [_ w196]
            tunnel: w164 -> [_ w185]
            frame False {
            }
            frame True {
              w187 = u16 86 items=["---MANUAL ENTRY---"=1000, "REG_NOREG"=0, "REG_RXBUFF_USED"=1, "REG_RXBUFF_BSIZE"=2, "REG_TXBUFF_USED"=3, "REG_TXBUFF_BSIZE"=4, "REG_TXBUFF_MAXPACKSIZE"=5, "REG_MAC_ERRCLR"=6, "REG_MAC_TRAINNUM"=7, "REG_MAC_SYNCMATCH"=8, "REG_MAC_SYNC1"=9, "REG_MAC_SYNC2"=10, "REG_MAC_SYNC3"=11, "REG_MAC_SYNC4"=12, "REG_MAC_SYNC5"=13, "REG_MAC_MAXBERR"=14, "REG_MAC_ECCORR"=15, "REG_MAC_CRCERR"=16, "REG_MAC_BLKCNT1"=17, "REG_MAC_BLKCNT2"=18, "REG_MAC_IMDTRANSID1"=19, "REG_MAC_IMDTRANSID2"=20, "REG_MAC_IMDTRANSID3"=21, "REG_MAC_COMPANYID"=22, "REG_MAC_MODUSER"=23, "REG_MAC_CHANNEL"=25, "REG_MAC_CLEARWDOG"=26, "REG_MAC_CKCORRTHRESH"=27, "REG_HK_TXADDR"=28, "REG_HK_TXDATA"=29, "REG_HK_TXREPLY"=30, "REG_HK_USERDATA"=31, "REG_HK_USERSTATUS"=32, "REG_HK_LASTADDRESS"=33, "REG_HK_MODE"=34, "REG_MAC_STATUSSEQ"=35, "REG_MAC_MAXRETRIES"=36, "REG_MAC_RESENDTIME"=37, "REG_MAC_POWERSAVETIME"=38, "REG_MAC_HEAD_DET"=39, "REG_MAC_CTRL"=41, "REG_MAC_INITCOM"=42, "REG_INTERFACE_MODE"=43, "REG_TXRXBUFF_BOTH"=44, "REG_TXRXBUFF"=45, "REG_IRQ_RAWSTATUS1"=46, "REG_IRQ_ENABLE1"=47, "REG_IRQ_ENABLESET1"=48, "REG_IRQ_ENABLECLEAR1"=49, "REG_IRQ_RAWSTATUS2"=50, "REG_IRQ_ENABLE2"=51, "REG_IRQ_ENABLESET2"=52, "REG_IRQ_ENABLECLEAR2"=53, "REG_IRQ_STATUS1"=54, "REG_IRQ_STATUS2"=55, "REG_IRQ_AUXSTATUS"=56, "REG_TXBUFF_OVERFLOW"=57, "REG_PO0"=58, "REG_P01"=59, "REG_P02"=60, "REG_P03"=61, "REG_GP0"=62, "REG_GPI"=63, "REG_WAKEUP_245IN"=64, "REG_WAKEUP_COMPANYID"=65, "REG_WAKEUP_IMDTRANSID1"=66, "REG_WAKEUP_IMDTRANSID2"=67, "REG_WAKEUP_IMDTRANSID3"=68, "REG_WAKEUP_CHANNEL"=69, "REG_WAKEUP_MODUSER"=70, "REG_WAKEUP_DEVICEMODE"=71, "REG_WAKEUP_WK_RX_CTRL1"=72, "REG_WAKEUP_STACK_ADDR"=73, "REG_WAKEUP_CTRL"=74, "REG_WAKEUP_STROSCRTRIM"=75, "REG_WAKEUP_BIASTRIM"=76, "REG_WAKEUP_ANT245TUNE"=77, "REG_WAKEUP_WK_RX_RTRIMDET"=78, "REG_WAKEUP_WK_RX_RTRIMDEMOD"=79, "REG_WAKEUP_WK_RX_RSSIGAIN"=80, "REG_WAKEUP_LNAFREQ1"=81, "REG_WAKEUP_STACK"=83, "REG_WAKUP_XOSU"=84, "REG_WAKUP_CNTDROPOUT"=85, "REG_WAKEUP_CRCCTRL"=86, "REG_WAKEUP_CRCWORD1"=87, "REG_WAKEUP_CRCWORD2"=88, "REG_WAKEUP_WK_RX_CTRIM"=89, "REG_WAKEUP_VDDATRIM"=90, "REG_WAKEUP_VDDDTRIM"=91, "REG_WAKEUP_TESTIOBUFEN"=92, "REG_WAKEUP_TESTIOCLAMP"=93, "CORE_RESET_ADDRESS"=94, "CHIP_RESET_ADDRESS"=95, "REG_RF_TXGENCTRL"=96, "REG_RF_TXIFCTRL"=97, "REG_RF_TXRF_SEL_CTRL"=98, "REG_RF_TXRFPWRDEFAULTSET"=99, "REG_RF_RSSITRIM"=100, "REG_RF_TXIFOSCTUNE"=101, "REG_RF_TXIFGAINIMB"=102, "REG_RF_TXIFLOCK"=103, "REG_RF_RXRFLNAGAINTRIM"=104, "REG_RF_RXBIASTR"=105, "REG_RF_RXGENCTRL"=106, "REG_RF_RXIFADCDECLEV"=107, "REG_RF_RXIFDETFILTERTUNE"=108, "REG_RF_RXIFFILTERTUNE"=109, "REG_RF_GENENABLES"=110, "REG_RF_SYNTH_CHANNEL"=111, "REG_TX_RAMP_RTRIM"=112, "REG_TX_RAMP_CTRIM"=113, "REG_RF_XO_TRIM"=114, "REG_RF_SYNTH_SET_TRIM"=115, "REG_RF_ADCCTRL"=116, "REG_RF_ADCOUTPUT"=117, "REG_RF_TXIFAMP"=118, "REG_RF_SYNTH_RTRIM"=119, "REG_RF_SYNTH_CTRIM"=120, "REG_RF_SYNTH_CT"=121, "REG_RF_TXMIXER_IOSTRIM_HIGH_IP"=122, "REG_RF_TXMIXER_IOSTRIM_HIGH_IN"=123, "REG_RF_TXMIXER_IOSTRIM_HIGH_QP"=124, "REG_RF_TXMIXER_IOSTRIM_HIGH_QN"=125, "REG_HX_WUADDR"=126, "REG_REVISION"=127, "REG_NOREG_TEST"=128, "REG_DTEST_RXBUFF"=129, "REG_RXBUFF_NEXT_BLOCK"=130, "REG_RXBUFF_FIRST_IN_PACK"=131, "REG_RXBUFF_FIRST_EMPTY"=132, "REG_MAC_BYPASS"=133, "REG_DTEST_TXBUFF"=134, "REG_TXBUFF_NEXT_BLOCK"=135, "REG_TXBUFF_FIRST_IN_PACK"=136, "REG_TXBUFF_FIRST_EMPTY"=137, "REG_DTEST_SEQ"=138, "REG_DTEST_CKCORR"=139, "REG_MAC_TOPSTATE"=140, "REG_DTEST_INTERFACE"=141, "REG_IFACE_TXRX_BYPASS"=142, "REG_MAC_TXRXWAIT"=143, "REG_MAC_TXRFRAMP"=144, "REG_MAC_TRAINWORD"=145, "REG_MAC_TRAINWORD2"=146, "REG_MAC_SETTINGS"=147, "REG_MAC_CALSELECT1"=148, "REG_MAC_CALSELECT2"=149, "REG_MAC_ANTMATCHSEL"=150, "REG_MAC_ANTTUNESEL1"=151, "REG_MAC_ANTTUNESEL2"=152, "REG_MAC_ANTTUNESEL3"=153, "REG_MAC_ANTTUNESTEP"=154, "REG_MAC_WUMODEBURST"=156, "REG_MAC_WUOFFSHORT"=157, "REG_MAC_WUOFFLONG"=158, "REG_MAC_CLKRECCTRL"=159, "REG_HK_MODE_P2"=162, "REG_MAC_ANTTUNERES1"=164, "REG_MAC_ANTTUNERES2"=165, "REG_INTERFACE_MODE_TEST"=171, "REG_TXRXBUFF_BOTH_P2"=172, "REG_TXRXBUFF_P2"=173, "REG_IRQ_RAWSTATUS1_P2"=174, "REG_MAC_TXIFSTATUS1"=176, "REG_MAC_TXIFSTATUS2"=177, "REG_IRQ_RAWSTATUS2_P2"=178, "REG_MAC_TXIFRAMPDELAY"=179, "REG_MAC_TXIFRAMPSLOPE"=180, "REG_MAX_TXIFRAMP"=181, "REG_IRQ_STATUS1_P2"=182, "REG_IRQ_STATUS2_P2"=183, "REG_IRQ_AUXSTATUS_P2"=184, "REG_MAC_UNLOCK"=188, "REG_MAC_TXIFFREQ"=190, "REG_WAKEUP_TESTCTRL1"=192, "REG_WAKEUP_RX_EN_CNT"=193, "REG_WAKEUP_TESTENABLES"=194, "REG_WAKEUP_DTBI_CTRL"=195, "REG_WAKEUP_DTBO_CTRL"=196, "REG_WAKEUP_TESTIOBUFTEST"=197, "REG_WAKEUP_WK_RX_TESTCTRL1"=198, "REG_WAKEUP_WK_RX_TESTCTRL2"=199, "REG_WAKEUP_SENS_SEQUENCE_CTRL"=200, "REG_WAKEUP_LNABIAS"=201, "REG_WAKEUP_DET_TH_TRIM1"=202, "REG_WAKEUP_LNABIAS_NOM1"=203, "REG_WAKEUP_RX_TSHORT_TRIM1"=204, "REG_WAKEUP_LNABIAS_NOM2"=205, "REG_WAKEUP_RX_TLONG_TRIM1"=206, "REG_WAKEUP_LNA_NEGRTRIM_NOM1"=207, "REG_WAKEUP_RX_TBURST_TRIM1"=208, "REG_WAKEUP_RX_LNA_NEGRTRIM_NOM2"=209, "REG_WAKEUP_RX_BB_G_BW_SEL1"=210, "REG_WAKEUP_WK_RX_DET_IOSTRIM1"=212, "REG_WAKEUP_WK_RX_CTRL2"=214, "REG_WAKEUP_WK_RX_RSSIVOSTRIM"=215, "REG_WAKEUP_LNANEGR_EFF"=216, "REG_WAKEUP_XOSU_FAST"=217, "REG_WAKEUP_STROSCPWIDTH1"=218, "REG_WAKEUP_STROSCPERIOD1"=220, "REG_WAKEUP_STROSCPERIOD2"=221, "REG_WAKEUP_WK_RX_LNA_NEGRTRIM1"=222, "REG_RF_TXTESTENABLE"=224, "REG_RF_TXIFTESTMODE"=225, "REG_RF_RXTESTENABLE"=226, "REG_RF_RXIFTESTCTRL1"=227, "REG_RF_RXIFTESTCTRL2"=228, "REG_RF_RXIFTESTCTRL3"=229, "REG_RF_SYNTH_TESTCTRL1"=230, "REG_RF_SYNTH_TESTCTRL2"=231, "REG_RF_SYNTH_TESTCTRL3"=232, "REG_RF_ADCTEST1"=237, "REG_RF_ADCTEST2"=238, "REG_RF_TXMIXER_IOSTRIM_LOW_IP"=240, "REG_RF_TXMIXER_IOSTRIM_LOW_IN"=241, "REG_RF_TXMIXER_ISOTRIM_LOW_QP"=242, "REG_RF_TXMIXER_IOSTRIM_LOW_QN"=243, "REG_RF_SYNTH_KPD"=244, "REG_RF_SYNTH_LOLEV"=245, "REG_RF_TXRFPWRTUNEANTSET"=246, "REG_RF_TXPD_GAIN_CTRL"=247, "REG_RF_SYNTH_STARTUP"=248, "REG_RF_TXRFANTTUNE_TXMODE"=249, "REG_RF_TXRFANTTUNE_RXMODE"=250, "REG_RF_RXRFANTTUNE_TXMODE"=251, "REG_RF_RXRFANTTUNE_RXMODE"=252, "REG_ANTMATCH1"=253, "REG_ANTMATCH2"=254, "REG_REVISION_P2"=255] ("Register")
              n45 = Select(t=6, s=w198, f=3) -> (s? t:f=w203:i32)
              n46 = Select(t=0, s=w198, f=3) -> (s? t:f=w199:i32)
              n47 = for {
                N: w203 -> [_]
                shift-right: [w228] -> w195
                shift-left: w212 -> [w229]
                tunnel: w211 -> [w227]
                tunnel: w210 -> [w226]
                tunnel: w209 -> [w225]
                tunnel: w208 -> [w224]
                tunnel: w207 -> [w223]
                tunnel: w199 -> [w220]
                tunnel: w197 -> [w219]
                tunnel: w196 -> [w218]
                tunnel: [w217] -> w190
                tunnel: [w216] -> w189
                tunnel: u32 20 ("milliseconds to wait") -> [w215]
                tunnel: w185 -> [w214]
                i -> [w221]
                n48 = Add(x=w220, y=w221) -> (x+y=w222:i32)
                n49 = Wait (ms)(milliseconds to wait=w215) -> ()  [unwired: 1 out]
                n50 = case shown="5" w222 {
                  tunnel: w229 -> [w235 w241 w249 w257 w265 w274]
                  tunnel: [w234 w240 w248 w256 w264 w273] -> w228
                  tunnel: w227 -> [_ _ _ w258 _ _]
                  tunnel: w226 -> [_ _ w251 _ _ _]
                  tunnel: w225 -> [w232 _ _ _ _ _]
                  tunnel: w224 -> [_ _ _ _ w266 _]
                  tunnel: w223 -> [_ w242 _ _ _ _]
                  tunnel: w219 -> [w231 w237 w245 w253 w261 w270]
                  tunnel: w218 -> [w230 w236 w244 w252 w260 w269]
                  tunnel: [w231 w237 w245 w253 w261 w270] -> w217
                  tunnel: [w230 w236 w244 w252 w260 w269] -> w216
                  tunnel: w214 -> [_ _ _ _ _ w268]
                  frame 0, Default {
                    w233 = u16 222 items=["---MANUAL ENTRY---"=1000, "REG_NOREG"=0, "REG_RXBUFF_USED"=1, "REG_RXBUFF_BSIZE"=2, "REG_TXBUFF_USED"=3, "REG_TXBUFF_BSIZE"=4, "REG_TXBUFF_MAXPACKSIZE"=5, "REG_MAC_ERRCLR"=6, "REG_MAC_TRAINNUM"=7, "REG_MAC_SYNCMATCH"=8, "REG_MAC_SYNC1"=9, "REG_MAC_SYNC2"=10, "REG_MAC_SYNC3"=11, "REG_MAC_SYNC4"=12, "REG_MAC_SYNC5"=13, "REG_MAC_MAXBERR"=14, "REG_MAC_ECCORR"=15, "REG_MAC_CRCERR"=16, "REG_MAC_BLKCNT1"=17, "REG_MAC_BLKCNT2"=18, "REG_MAC_IMDTRANSID1"=19, "REG_MAC_IMDTRANSID2"=20, "REG_MAC_IMDTRANSID3"=21, "REG_MAC_COMPANYID"=22, "REG_MAC_MODUSER"=23, "REG_MAC_CHANNEL"=25, "REG_MAC_CLEARWDOG"=26, "REG_MAC_CKCORRTHRESH"=27, "REG_HK_TXADDR"=28, "REG_HK_TXDATA"=29, "REG_HK_TXREPLY"=30, "REG_HK_USERDATA"=31, "REG_HK_USERSTATUS"=32, "REG_HK_LASTADDRESS"=33, "REG_HK_MODE"=34, "REG_MAC_STATUSSEQ"=35, "REG_MAC_MAXRETRIES"=36, "REG_MAC_RESENDTIME"=37, "REG_MAC_POWERSAVETIME"=38, "REG_MAC_HEAD_DET"=39, "REG_MAC_CTRL"=41, "REG_MAC_INITCOM"=42, "REG_INTERFACE_MODE"=43, "REG_TXRXBUFF_BOTH"=44, "REG_TXRXBUFF"=45, "REG_IRQ_RAWSTATUS1"=46, "REG_IRQ_ENABLE1"=47, "REG_IRQ_ENABLESET1"=48, "REG_IRQ_ENABLECLEAR1"=49, "REG_IRQ_RAWSTATUS2"=50, "REG_IRQ_ENABLE2"=51, "REG_IRQ_ENABLESET2"=52, "REG_IRQ_ENABLECLEAR2"=53, "REG_IRQ_STATUS1"=54, "REG_IRQ_STATUS2"=55, "REG_IRQ_AUXSTATUS"=56, "REG_TXBUFF_OVERFLOW"=57, "REG_PO0"=58, "REG_P01"=59, "REG_P02"=60, "REG_P03"=61, "REG_GP0"=62, "REG_GPI"=63, "REG_WAKEUP_245IN"=64, "REG_WAKEUP_COMPANYID"=65, "REG_WAKEUP_IMDTRANSID1"=66, "REG_WAKEUP_IMDTRANSID2"=67, "REG_WAKEUP_IMDTRANSID3"=68, "REG_WAKEUP_CHANNEL"=69, "REG_WAKEUP_MODUSER"=70, "REG_WAKEUP_DEVICEMODE"=71, "REG_WAKEUP_WK_RX_CTRL1"=72, "REG_WAKEUP_STACK_ADDR"=73, "REG_WAKEUP_CTRL"=74, "REG_WAKEUP_STROSCRTRIM"=75, "REG_WAKEUP_BIASTRIM"=76, "REG_WAKEUP_ANT245TUNE"=77, "REG_WAKEUP_WK_RX_RTRIMDET"=78, "REG_WAKEUP_WK_RX_RTRIMDEMOD"=79, "REG_WAKEUP_WK_RX_RSSIGAIN"=80, "REG_WAKEUP_LNAFREQ1"=81, "REG_WAKEUP_STACK"=83, "REG_WAKUP_XOSU"=84, "REG_WAKUP_CNTDROPOUT"=85, "REG_WAKEUP_CRCCTRL"=86, "REG_WAKEUP_CRCWORD1"=87, "REG_WAKEUP_CRCWORD2"=88, "REG_WAKEUP_WK_RX_CTRIM"=89, "REG_WAKEUP_VDDATRIM"=90, "REG_WAKEUP_VDDDTRIM"=91, "REG_WAKEUP_TESTIOBUFEN"=92, "REG_WAKEUP_TESTIOCLAMP"=93, "CORE_RESET_ADDRESS"=94, "CHIP_RESET_ADDRESS"=95, "REG_RF_TXGENCTRL"=96, "REG_RF_TXIFCTRL"=97, "REG_RF_TXRF_SEL_CTRL"=98, "REG_RF_TXRFPWRDEFAULTSET"=99, "REG_RF_RSSITRIM"=100, "REG_RF_TXIFOSCTUNE"=101, "REG_RF_TXIFGAINIMB"=102, "REG_RF_TXIFLOCK"=103, "REG_RF_RXRFLNAGAINTRIM"=104, "REG_RF_RXBIASTR"=105, "REG_RF_RXGENCTRL"=106, "REG_RF_RXIFADCDECLEV"=107, "REG_RF_RXIFDETFILTERTUNE"=108, "REG_RF_RXIFFILTERTUNE"=109, "REG_RF_GENENABLES"=110, "REG_RF_SYNTH_CHANNEL"=111, "REG_TX_RAMP_RTRIM"=112, "REG_TX_RAMP_CTRIM"=113, "REG_RF_XO_TRIM"=114, "REG_RF_SYNTH_SET_TRIM"=115, "REG_RF_ADCCTRL"=116, "REG_RF_ADCOUTPUT"=117, "REG_RF_TXIFAMP"=118, "REG_RF_SYNTH_RTRIM"=119, "REG_RF_SYNTH_CTRIM"=120, "REG_RF_SYNTH_CT"=121, "REG_RF_TXMIXER_IOSTRIM_HIGH_IP"=122, "REG_RF_TXMIXER_IOSTRIM_HIGH_IN"=123, "REG_RF_TXMIXER_IOSTRIM_HIGH_QP"=124, "REG_RF_TXMIXER_IOSTRIM_HIGH_QN"=125, "REG_HX_WUADDR"=126, "REG_REVISION"=127, "REG_NOREG_TEST"=128, "REG_DTEST_RXBUFF"=129, "REG_RXBUFF_NEXT_BLOCK"=130, "REG_RXBUFF_FIRST_IN_PACK"=131, "REG_RXBUFF_FIRST_EMPTY"=132, "REG_MAC_BYPASS"=133, "REG_DTEST_TXBUFF"=134, "REG_TXBUFF_NEXT_BLOCK"=135, "REG_TXBUFF_FIRST_IN_PACK"=136, "REG_TXBUFF_FIRST_EMPTY"=137, "REG_DTEST_SEQ"=138, "REG_DTEST_CKCORR"=139, "REG_MAC_TOPSTATE"=140, "REG_DTEST_INTERFACE"=141, "REG_IFACE_TXRX_BYPASS"=142, "REG_MAC_TXRXWAIT"=143, "REG_MAC_TXRFRAMP"=144, "REG_MAC_TRAINWORD"=145, "REG_MAC_TRAINWORD2"=146, "REG_MAC_SETTINGS"=147, "REG_MAC_CALSELECT1"=148, "REG_MAC_CALSELECT2"=149, "REG_MAC_ANTMATCHSEL"=150, "REG_MAC_ANTTUNESEL1"=151, "REG_MAC_ANTTUNESEL2"=152, "REG_MAC_ANTTUNESEL3"=153, "REG_MAC_ANTTUNESTEP"=154, "REG_MAC_WUMODEBURST"=156, "REG_MAC_WUOFFSHORT"=157, "REG_MAC_WUOFFLONG"=158, "REG_MAC_CLKRECCTRL"=159, "REG_HK_MODE_P2"=162, "REG_MAC_ANTTUNERES1"=164, "REG_MAC_ANTTUNERES2"=165, "REG_INTERFACE_MODE_TEST"=171, "REG_TXRXBUFF_BOTH_P2"=172, "REG_TXRXBUFF_P2"=173, "REG_IRQ_RAWSTATUS1_P2"=174, "REG_MAC_TXIFSTATUS1"=176, "REG_MAC_TXIFSTATUS2"=177, "REG_IRQ_RAWSTATUS2_P2"=178, "REG_MAC_TXIFRAMPDELAY"=179, "REG_MAC_TXIFRAMPSLOPE"=180, "REG_MAX_TXIFRAMP"=181, "REG_IRQ_STATUS1_P2"=182, "REG_IRQ_STATUS2_P2"=183, "REG_IRQ_AUXSTATUS_P2"=184, "REG_MAC_UNLOCK"=188, "REG_MAC_TXIFFREQ"=190, "REG_WAKEUP_TESTCTRL1"=192, "REG_WAKEUP_RX_EN_CNT"=193, "REG_WAKEUP_TESTENABLES"=194, "REG_WAKEUP_DTBI_CTRL"=195, "REG_WAKEUP_DTBO_CTRL"=196, "REG_WAKEUP_TESTIOBUFTEST"=197, "REG_WAKEUP_WK_RX_TESTCTRL1"=198, "REG_WAKEUP_WK_RX_TESTCTRL2"=199, "REG_WAKEUP_SENS_SEQUENCE_CTRL"=200, "REG_WAKEUP_LNABIAS"=201, "REG_WAKEUP_DET_TH_TRIM1"=202, "REG_WAKEUP_LNABIAS_NOM1"=203, "REG_WAKEUP_RX_TSHORT_TRIM1"=204, "REG_WAKEUP_LNABIAS_NOM2"=205, "REG_WAKEUP_RX_TLONG_TRIM1"=206, "REG_WAKEUP_LNA_NEGRTRIM_NOM1"=207, "REG_WAKEUP_RX_TBURST_TRIM1"=208, "REG_WAKEUP_RX_LNA_NEGRTRIM_NOM2"=209, "REG_WAKEUP_RX_BB_G_BW_SEL1"=210, "REG_WAKEUP_WK_RX_DET_IOSTRIM1"=212, "REG_WAKEUP_WK_RX_CTRL2"=214, "REG_WAKEUP_WK_RX_RSSIVOSTRIM"=215, "REG_WAKEUP_LNANEGR_EFF"=216, "REG_WAKEUP_XOSU_FAST"=217, "REG_WAKEUP_STROSCPWIDTH1"=218, "REG_WAKEUP_STROSCPERIOD1"=220, "REG_WAKEUP_STROSCPERIOD2"=221, "REG_WAKEUP_WK_RX_LNA_NEGRTRIM1"=222, "REG_RF_TXTESTENABLE"=224, "REG_RF_TXIFTESTMODE"=225, "REG_RF_RXTESTENABLE"=226, "REG_RF_RXIFTESTCTRL1"=227, "REG_RF_RXIFTESTCTRL2"=228, "REG_RF_RXIFTESTCTRL3"=229, "REG_RF_SYNTH_TESTCTRL1"=230, "REG_RF_SYNTH_TESTCTRL2"=231, "REG_RF_SYNTH_TESTCTRL3"=232, "REG_RF_ADCTEST1"=237, "REG_RF_ADCTEST2"=238, "REG_RF_TXMIXER_IOSTRIM_LOW_IP"=240, "REG_RF_TXMIXER_IOSTRIM_LOW_IN"=241, "REG_RF_TXMIXER_ISOTRIM_LOW_QP"=242, "REG_RF_TXMIXER_IOSTRIM_LOW_QN"=243, "REG_RF_SYNTH_KPD"=244, "REG_RF_SYNTH_LOLEV"=245, "REG_RF_TXRFPWRTUNEANTSET"=246, "REG_RF_TXPD_GAIN_CTRL"=247, "REG_RF_SYNTH_STARTUP"=248, "REG_RF_TXRFANTTUNE_TXMODE"=249, "REG_RF_TXRFANTTUNE_RXMODE"=250, "REG_RF_RXRFANTTUNE_TXMODE"=251, "REG_RF_RXRFANTTUNE_RXMODE"=252, "REG_ANTMATCH1"=253, "REG_ANTMATCH2"=254, "REG_REVISION_P2"=255] ("Register")
                    # "Apply LNA Gain (NEGRTRIM) value"
                    # "Address"
                    n51 = call "JTAG SPI.vi"("Value"=w232, "error in (no error)"=w235, "Target"=w230, "Function"=w231, "Address"=w233) -> ("error out"=w234:errorcluster)  [unwired: 3 in, 3 out]
                  }
                  frame 1 {
                    w239 = u16 81 items=["---MANUAL ENTRY---"=1000, "REG_NOREG"=0, "REG_RXBUFF_USED"=1, "REG_RXBUFF_BSIZE"=2, "REG_TXBUFF_USED"=3, "REG_TXBUFF_BSIZE"=4, "REG_TXBUFF_MAXPACKSIZE"=5, "REG_MAC_ERRCLR"=6, "REG_MAC_TRAINNUM"=7, "REG_MAC_SYNCMATCH"=8, "REG_MAC_SYNC1"=9, "REG_MAC_SYNC2"=10, "REG_MAC_SYNC3"=11, "REG_MAC_SYNC4"=12, "REG_MAC_SYNC5"=13, "REG_MAC_MAXBERR"=14, "REG_MAC_ECCORR"=15, "REG_MAC_CRCERR"=16, "REG_MAC_BLKCNT1"=17, "REG_MAC_BLKCNT2"=18, "REG_MAC_IMDTRANSID1"=19, "REG_MAC_IMDTRANSID2"=20, "REG_MAC_IMDTRANSID3"=21, "REG_MAC_COMPANYID"=22, "REG_MAC_MODUSER"=23, "REG_MAC_CHANNEL"=25, "REG_MAC_CLEARWDOG"=26, "REG_MAC_CKCORRTHRESH"=27, "REG_HK_TXADDR"=28, "REG_HK_TXDATA"=29, "REG_HK_TXREPLY"=30, "REG_HK_USERDATA"=31, "REG_HK_USERSTATUS"=32, "REG_HK_LASTADDRESS"=33, "REG_HK_MODE"=34, "REG_MAC_STATUSSEQ"=35, "REG_MAC_MAXRETRIES"=36, "REG_MAC_RESENDTIME"=37, "REG_MAC_POWERSAVETIME"=38, "REG_MAC_HEAD_DET"=39, "REG_MAC_CTRL"=41, "REG_MAC_INITCOM"=42, "REG_INTERFACE_MODE"=43, "REG_TXRXBUFF_BOTH"=44, "REG_TXRXBUFF"=45, "REG_IRQ_RAWSTATUS1"=46, "REG_IRQ_ENABLE1"=47, "REG_IRQ_ENABLESET1"=48, "REG_IRQ_ENABLECLEAR1"=49, "REG_IRQ_RAWSTATUS2"=50, "REG_IRQ_ENABLE2"=51, "REG_IRQ_ENABLESET2"=52, "REG_IRQ_ENABLECLEAR2"=53, "REG_IRQ_STATUS1"=54, "REG_IRQ_STATUS2"=55, "REG_IRQ_AUXSTATUS"=56, "REG_TXBUFF_OVERFLOW"=57, "REG_PO0"=58, "REG_P01"=59, "REG_P02"=60, "REG_P03"=61, "REG_GP0"=62, "REG_GPI"=63, "REG_WAKEUP_245IN"=64, "REG_WAKEUP_COMPANYID"=65, "REG_WAKEUP_IMDTRANSID1"=66, "REG_WAKEUP_IMDTRANSID2"=67, "REG_WAKEUP_IMDTRANSID3"=68, "REG_WAKEUP_CHANNEL"=69, "REG_WAKEUP_MODUSER"=70, "REG_WAKEUP_DEVICEMODE"=71, "REG_WAKEUP_WK_RX_CTRL1"=72, "REG_WAKEUP_STACK_ADDR"=73, "REG_WAKEUP_CTRL"=74, "REG_WAKEUP_STROSCRTRIM"=75, "REG_WAKEUP_BIASTRIM"=76, "REG_WAKEUP_ANT245TUNE"=77, "REG_WAKEUP_WK_RX_RTRIMDET"=78, "REG_WAKEUP_WK_RX_RTRIMDEMOD"=79, "REG_WAKEUP_WK_RX_RSSIGAIN"=80, "REG_WAKEUP_LNAFREQ1"=81, "REG_WAKEUP_STACK"=83, "REG_WAKUP_XOSU"=84, "REG_WAKUP_CNTDROPOUT"=85, "REG_WAKEUP_CRCCTRL"=86, "REG_WAKEUP_CRCWORD1"=87, "REG_WAKEUP_CRCWORD2"=88, "REG_WAKEUP_WK_RX_CTRIM"=89, "REG_WAKEUP_VDDATRIM"=90, "REG_WAKEUP_VDDDTRIM"=91, "REG_WAKEUP_TESTIOBUFEN"=92, "REG_WAKEUP_TESTIOCLAMP"=93, "CORE_RESET_ADDRESS"=94, "CHIP_RESET_ADDRESS"=95, "REG_RF_TXGENCTRL"=96, "REG_RF_TXIFCTRL"=97, "REG_RF_TXRF_SEL_CTRL"=98, "REG_RF_TXRFPWRDEFAULTSET"=99, "REG_RF_RSSITRIM"=100, "REG_RF_TXIFOSCTUNE"=101, "REG_RF_TXIFGAINIMB"=102, "REG_RF_TXIFLOCK"=103, "REG_RF_RXRFLNAGAINTRIM"=104, "REG_RF_RXBIASTR"=105, "REG_RF_RXGENCTRL"=106, "REG_RF_RXIFADCDECLEV"=107, "REG_RF_RXIFDETFILTERTUNE"=108, "REG_RF_RXIFFILTERTUNE"=109, "REG_RF_GENENABLES"=110, "REG_RF_SYNTH_CHANNEL"=111, "REG_TX_RAMP_RTRIM"=112, "REG_TX_RAMP_CTRIM"=113, "REG_RF_XO_TRIM"=114, "REG_RF_SYNTH_SET_TRIM"=115, "REG_RF_ADCCTRL"=116, "REG_RF_ADCOUTPUT"=117, "REG_RF_TXIFAMP"=118, "REG_RF_SYNTH_RTRIM"=119, "REG_RF_SYNTH_CTRIM"=120, "REG_RF_SYNTH_CT"=121, "REG_RF_TXMIXER_IOSTRIM_HIGH_IP"=122, "REG_RF_TXMIXER_IOSTRIM_HIGH_IN"=123, "REG_RF_TXMIXER_IOSTRIM_HIGH_QP"=124, "REG_RF_TXMIXER_IOSTRIM_HIGH_QN"=125, "REG_HX_WUADDR"=126, "REG_REVISION"=127, "REG_NOREG_TEST"=128, "REG_DTEST_RXBUFF"=129, "REG_RXBUFF_NEXT_BLOCK"=130, "REG_RXBUFF_FIRST_IN_PACK"=131, "REG_RXBUFF_FIRST_EMPTY"=132, "REG_MAC_BYPASS"=133, "REG_DTEST_TXBUFF"=134, "REG_TXBUFF_NEXT_BLOCK"=135, "REG_TXBUFF_FIRST_IN_PACK"=136, "REG_TXBUFF_FIRST_EMPTY"=137, "REG_DTEST_SEQ"=138, "REG_DTEST_CKCORR"=139, "REG_MAC_TOPSTATE"=140, "REG_DTEST_INTERFACE"=141, "REG_IFACE_TXRX_BYPASS"=142, "REG_MAC_TXRXWAIT"=143, "REG_MAC_TXRFRAMP"=144, "REG_MAC_TRAINWORD"=145, "REG_MAC_TRAINWORD2"=146, "REG_MAC_SETTINGS"=147, "REG_MAC_CALSELECT1"=148, "REG_MAC_CALSELECT2"=149, "REG_MAC_ANTMATCHSEL"=150, "REG_MAC_ANTTUNESEL1"=151, "REG_MAC_ANTTUNESEL2"=152, "REG_MAC_ANTTUNESEL3"=153, "REG_MAC_ANTTUNESTEP"=154, "REG_MAC_WUMODEBURST"=156, "REG_MAC_WUOFFSHORT"=157, "REG_MAC_WUOFFLONG"=158, "REG_MAC_CLKRECCTRL"=159, "REG_HK_MODE_P2"=162, "REG_MAC_ANTTUNERES1"=164, "REG_MAC_ANTTUNERES2"=165, "REG_INTERFACE_MODE_TEST"=171, "REG_TXRXBUFF_BOTH_P2"=172, "REG_TXRXBUFF_P2"=173, "REG_IRQ_RAWSTATUS1_P2"=174, "REG_MAC_TXIFSTATUS1"=176, "REG_MAC_TXIFSTATUS2"=177, "REG_IRQ_RAWSTATUS2_P2"=178, "REG_MAC_TXIFRAMPDELAY"=179, "REG_MAC_TXIFRAMPSLOPE"=180, "REG_MAX_TXIFRAMP"=181, "REG_IRQ_STATUS1_P2"=182, "REG_IRQ_STATUS2_P2"=183, "REG_IRQ_AUXSTATUS_P2"=184, "REG_MAC_UNLOCK"=188, "REG_MAC_TXIFFREQ"=190, "REG_WAKEUP_TESTCTRL1"=192, "REG_WAKEUP_RX_EN_CNT"=193, "REG_WAKEUP_TESTENABLES"=194, "REG_WAKEUP_DTBI_CTRL"=195, "REG_WAKEUP_DTBO_CTRL"=196, "REG_WAKEUP_TESTIOBUFTEST"=197, "REG_WAKEUP_WK_RX_TESTCTRL1"=198, "REG_WAKEUP_WK_RX_TESTCTRL2"=199, "REG_WAKEUP_SENS_SEQUENCE_CTRL"=200, "REG_WAKEUP_LNABIAS"=201, "REG_WAKEUP_DET_TH_TRIM1"=202, "REG_WAKEUP_LNABIAS_NOM1"=203, "REG_WAKEUP_RX_TSHORT_TRIM1"=204, "REG_WAKEUP_LNABIAS_NOM2"=205, "REG_WAKEUP_RX_TLONG_TRIM1"=206, "REG_WAKEUP_LNA_NEGRTRIM_NOM1"=207, "REG_WAKEUP_RX_TBURST_TRIM1"=208, "REG_WAKEUP_RX_LNA_NEGRTRIM_NOM2"=209, "REG_WAKEUP_RX_BB_G_BW_SEL1"=210, "REG_WAKEUP_WK_RX_DET_IOSTRIM1"=212, "REG_WAKEUP_WK_RX_CTRL2"=214, "REG_WAKEUP_WK_RX_RSSIVOSTRIM"=215, "REG_WAKEUP_LNANEGR_EFF"=216, "REG_WAKEUP_XOSU_FAST"=217, "REG_WAKEUP_STROSCPWIDTH1"=218, "REG_WAKEUP_STROSCPERIOD1"=220, "REG_WAKEUP_STROSCPERIOD2"=221, "REG_WAKEUP_WK_RX_LNA_NEGRTRIM1"=222, "REG_RF_TXTESTENABLE"=224, "REG_RF_TXIFTESTMODE"=225, "REG_RF_RXTESTENABLE"=226, "REG_RF_RXIFTESTCTRL1"=227, "REG_RF_RXIFTESTCTRL2"=228, "REG_RF_RXIFTESTCTRL3"=229, "REG_RF_SYNTH_TESTCTRL1"=230, "REG_RF_SYNTH_TESTCTRL2"=231, "REG_RF_SYNTH_TESTCTRL3"=232, "REG_RF_ADCTEST1"=237, "REG_RF_ADCTEST2"=238, "REG_RF_TXMIXER_IOSTRIM_LOW_IP"=240, "REG_RF_TXMIXER_IOSTRIM_LOW_IN"=241, "REG_RF_TXMIXER_ISOTRIM_LOW_QP"=242, "REG_RF_TXMIXER_IOSTRIM_LOW_QN"=243, "REG_RF_SYNTH_KPD"=244, "REG_RF_SYNTH_LOLEV"=245, "REG_RF_TXRFPWRTUNEANTSET"=246, "REG_RF_TXPD_GAIN_CTRL"=247, "REG_RF_SYNTH_STARTUP"=248, "REG_RF_TXRFANTTUNE_TXMODE"=249, "REG_RF_TXRFANTTUNE_RXMODE"=250, "REG_RF_RXRFANTTUNE_TXMODE"=251, "REG_RF_RXRFANTTUNE_RXMODE"=252, "REG_ANTMATCH1"=253, "REG_ANTMATCH2"=254, "REG_REVISION_P2"=255] ("Register")
                    # "Apply LNA Frequency Trim value"
                    # "Address"
                    # "Bitmask"
                    n52 = And(x=w242, y=u8 31 ("Data")) -> (x .and. y?=w238:u8)
                    n53 = call "JTAG SPI.vi"("Value"=w238, "error in (no error)"=w241, "Target"=w236, "Function"=w237, "Address"=w239) -> ("error out"=w240:errorcluster)  [unwired: 3 in, 3 out]
                  }
                  frame 2 {
                    w247 = u16 77 items=["---MANUAL ENTRY---"=1000, "REG_NOREG"=0, "REG_RXBUFF_USED"=1, "REG_RXBUFF_BSIZE"=2, "REG_TXBUFF_USED"=3, "REG_TXBUFF_BSIZE"=4, "REG_TXBUFF_MAXPACKSIZE"=5, "REG_MAC_ERRCLR"=6, "REG_MAC_TRAINNUM"=7, "REG_MAC_SYNCMATCH"=8, "REG_MAC_SYNC1"=9, "REG_MAC_SYNC2"=10, "REG_MAC_SYNC3"=11, "REG_MAC_SYNC4"=12, "REG_MAC_SYNC5"=13, "REG_MAC_MAXBERR"=14, "REG_MAC_ECCORR"=15, "REG_MAC_CRCERR"=16, "REG_MAC_BLKCNT1"=17, "REG_MAC_BLKCNT2"=18, "REG_MAC_IMDTRANSID1"=19, "REG_MAC_IMDTRANSID2"=20, "REG_MAC_IMDTRANSID3"=21, "REG_MAC_COMPANYID"=22, "REG_MAC_MODUSER"=23, "REG_MAC_CHANNEL"=25, "REG_MAC_CLEARWDOG"=26, "REG_MAC_CKCORRTHRESH"=27, "REG_HK_TXADDR"=28, "REG_HK_TXDATA"=29, "REG_HK_TXREPLY"=30, "REG_HK_USERDATA"=31, "REG_HK_USERSTATUS"=32, "REG_HK_LASTADDRESS"=33, "REG_HK_MODE"=34, "REG_MAC_STATUSSEQ"=35, "REG_MAC_MAXRETRIES"=36, "REG_MAC_RESENDTIME"=37, "REG_MAC_POWERSAVETIME"=38, "REG_MAC_HEAD_DET"=39, "REG_MAC_CTRL"=41, "REG_MAC_INITCOM"=42, "REG_INTERFACE_MODE"=43, "REG_TXRXBUFF_BOTH"=44, "REG_TXRXBUFF"=45, "REG_IRQ_RAWSTATUS1"=46, "REG_IRQ_ENABLE1"=47, "REG_IRQ_ENABLESET1"=48, "REG_IRQ_ENABLECLEAR1"=49, "REG_IRQ_RAWSTATUS2"=50, "REG_IRQ_ENABLE2"=51, "REG_IRQ_ENABLESET2"=52, "REG_IRQ_ENABLECLEAR2"=53, "REG_IRQ_STATUS1"=54, "REG_IRQ_STATUS2"=55, "REG_IRQ_AUXSTATUS"=56, "REG_TXBUFF_OVERFLOW"=57, "REG_PO0"=58, "REG_P01"=59, "REG_P02"=60, "REG_P03"=61, "REG_GP0"=62, "REG_GPI"=63, "REG_WAKEUP_245IN"=64, "REG_WAKEUP_COMPANYID"=65, "REG_WAKEUP_IMDTRANSID1"=66, "REG_WAKEUP_IMDTRANSID2"=67, "REG_WAKEUP_IMDTRANSID3"=68, "REG_WAKEUP_CHANNEL"=69, "REG_WAKEUP_MODUSER"=70, "REG_WAKEUP_DEVICEMODE"=71, "REG_WAKEUP_WK_RX_CTRL1"=72, "REG_WAKEUP_STACK_ADDR"=73, "REG_WAKEUP_CTRL"=74, "REG_WAKEUP_STROSCRTRIM"=75, "REG_WAKEUP_BIASTRIM"=76, "REG_WAKEUP_ANT245TUNE"=77, "REG_WAKEUP_WK_RX_RTRIMDET"=78, "REG_WAKEUP_WK_RX_RTRIMDEMOD"=79, "REG_WAKEUP_WK_RX_RSSIGAIN"=80, "REG_WAKEUP_LNAFREQ1"=81, "REG_WAKEUP_STACK"=83, "REG_WAKUP_XOSU"=84, "REG_WAKUP_CNTDROPOUT"=85, "REG_WAKEUP_CRCCTRL"=86, "REG_WAKEUP_CRCWORD1"=87, "REG_WAKEUP_CRCWORD2"=88, "REG_WAKEUP_WK_RX_CTRIM"=89, "REG_WAKEUP_VDDATRIM"=90, "REG_WAKEUP_VDDDTRIM"=91, "REG_WAKEUP_TESTIOBUFEN"=92, "REG_WAKEUP_TESTIOCLAMP"=93, "CORE_RESET_ADDRESS"=94, "CHIP_RESET_ADDRESS"=95, "REG_RF_TXGENCTRL"=96, "REG_RF_TXIFCTRL"=97, "REG_RF_TXRF_SEL_CTRL"=98, "REG_RF_TXRFPWRDEFAULTSET"=99, "REG_RF_RSSITRIM"=100, "REG_RF_TXIFOSCTUNE"=101, "REG_RF_TXIFGAINIMB"=102, "REG_RF_TXIFLOCK"=103, "REG_RF_RXRFLNAGAINTRIM"=104, "REG_RF_RXBIASTR"=105, "REG_RF_RXGENCTRL"=106, "REG_RF_RXIFADCDECLEV"=107, "REG_RF_RXIFDETFILTERTUNE"=108, "REG_RF_RXIFFILTERTUNE"=109, "REG_RF_GENENABLES"=110, "REG_RF_SYNTH_CHANNEL"=111, "REG_TX_RAMP_RTRIM"=112, "REG_TX_RAMP_CTRIM"=113, "REG_RF_XO_TRIM"=114, "REG_RF_SYNTH_SET_TRIM"=115, "REG_RF_ADCCTRL"=116, "REG_RF_ADCOUTPUT"=117, "REG_RF_TXIFAMP"=118, "REG_RF_SYNTH_RTRIM"=119, "REG_RF_SYNTH_CTRIM"=120, "REG_RF_SYNTH_CT"=121, "REG_RF_TXMIXER_IOSTRIM_HIGH_IP"=122, "REG_RF_TXMIXER_IOSTRIM_HIGH_IN"=123, "REG_RF_TXMIXER_IOSTRIM_HIGH_QP"=124, "REG_RF_TXMIXER_IOSTRIM_HIGH_QN"=125, "REG_HX_WUADDR"=126, "REG_REVISION"=127, "REG_NOREG_TEST"=128, "REG_DTEST_RXBUFF"=129, "REG_RXBUFF_NEXT_BLOCK"=130, "REG_RXBUFF_FIRST_IN_PACK"=131, "REG_RXBUFF_FIRST_EMPTY"=132, "REG_MAC_BYPASS"=133, "REG_DTEST_TXBUFF"=134, "REG_TXBUFF_NEXT_BLOCK"=135, "REG_TXBUFF_FIRST_IN_PACK"=136, "REG_TXBUFF_FIRST_EMPTY"=137, "REG_DTEST_SEQ"=138, "REG_DTEST_CKCORR"=139, "REG_MAC_TOPSTATE"=140, "REG_DTEST_INTERFACE"=141, "REG_IFACE_TXRX_BYPASS"=142, "REG_MAC_TXRXWAIT"=143, "REG_MAC_TXRFRAMP"=144, "REG_MAC_TRAINWORD"=145, "REG_MAC_TRAINWORD2"=146, "REG_MAC_SETTINGS"=147, "REG_MAC_CALSELECT1"=148, "REG_MAC_CALSELECT2"=149, "REG_MAC_ANTMATCHSEL"=150, "REG_MAC_ANTTUNESEL1"=151, "REG_MAC_ANTTUNESEL2"=152, "REG_MAC_ANTTUNESEL3"=153, "REG_MAC_ANTTUNESTEP"=154, "REG_MAC_WUMODEBURST"=156, "REG_MAC_WUOFFSHORT"=157, "REG_MAC_WUOFFLONG"=158, "REG_MAC_CLKRECCTRL"=159, "REG_HK_MODE_P2"=162, "REG_MAC_ANTTUNERES1"=164, "REG_MAC_ANTTUNERES2"=165, "REG_INTERFACE_MODE_TEST"=171, "REG_TXRXBUFF_BOTH_P2"=172, "REG_TXRXBUFF_P2"=173, "REG_IRQ_RAWSTATUS1_P2"=174, "REG_MAC_TXIFSTATUS1"=176, "REG_MAC_TXIFSTATUS2"=177, "REG_IRQ_RAWSTATUS2_P2"=178, "REG_MAC_TXIFRAMPDELAY"=179, "REG_MAC_TXIFRAMPSLOPE"=180, "REG_MAX_TXIFRAMP"=181, "REG_IRQ_STATUS1_P2"=182, "REG_IRQ_STATUS2_P2"=183, "REG_IRQ_AUXSTATUS_P2"=184, "REG_MAC_UNLOCK"=188, "REG_MAC_TXIFFREQ"=190, "REG_WAKEUP_TESTCTRL1"=192, "REG_WAKEUP_RX_EN_CNT"=193, "REG_WAKEUP_TESTENABLES"=194, "REG_WAKEUP_DTBI_CTRL"=195, "REG_WAKEUP_DTBO_CTRL"=196, "REG_WAKEUP_TESTIOBUFTEST"=197, "REG_WAKEUP_WK_RX_TESTCTRL1"=198, "REG_WAKEUP_WK_RX_TESTCTRL2"=199, "REG_WAKEUP_SENS_SEQUENCE_CTRL"=200, "REG_WAKEUP_LNABIAS"=201, "REG_WAKEUP_DET_TH_TRIM1"=202, "REG_WAKEUP_LNABIAS_NOM1"=203, "REG_WAKEUP_RX_TSHORT_TRIM1"=204, "REG_WAKEUP_LNABIAS_NOM2"=205, "REG_WAKEUP_RX_TLONG_TRIM1"=206, "REG_WAKEUP_LNA_NEGRTRIM_NOM1"=207, "REG_WAKEUP_RX_TBURST_TRIM1"=208, "REG_WAKEUP_RX_LNA_NEGRTRIM_NOM2"=209, "REG_WAKEUP_RX_BB_G_BW_SEL1"=210, "REG_WAKEUP_WK_RX_DET_IOSTRIM1"=212, "REG_WAKEUP_WK_RX_CTRL2"=214, "REG_WAKEUP_WK_RX_RSSIVOSTRIM"=215, "REG_WAKEUP_LNANEGR_EFF"=216, "REG_WAKEUP_XOSU_FAST"=217, "REG_WAKEUP_STROSCPWIDTH1"=218, "REG_WAKEUP_STROSCPERIOD1"=220, "REG_WAKEUP_STROSCPERIOD2"=221, "REG_WAKEUP_WK_RX_LNA_NEGRTRIM1"=222, "REG_RF_TXTESTENABLE"=224, "REG_RF_TXIFTESTMODE"=225, "REG_RF_RXTESTENABLE"=226, "REG_RF_RXIFTESTCTRL1"=227, "REG_RF_RXIFTESTCTRL2"=228, "REG_RF_RXIFTESTCTRL3"=229, "REG_RF_SYNTH_TESTCTRL1"=230, "REG_RF_SYNTH_TESTCTRL2"=231, "REG_RF_SYNTH_TESTCTRL3"=232, "REG_RF_ADCTEST1"=237, "REG_RF_ADCTEST2"=238, "REG_RF_TXMIXER_IOSTRIM_LOW_IP"=240, "REG_RF_TXMIXER_IOSTRIM_LOW_IN"=241, "REG_RF_TXMIXER_ISOTRIM_LOW_QP"=242, "REG_RF_TXMIXER_IOSTRIM_LOW_QN"=243, "REG_RF_SYNTH_KPD"=244, "REG_RF_SYNTH_LOLEV"=245, "REG_RF_TXRFPWRTUNEANTSET"=246, "REG_RF_TXPD_GAIN_CTRL"=247, "REG_RF_SYNTH_STARTUP"=248, "REG_RF_TXRFANTTUNE_TXMODE"=249, "REG_RF_TXRFANTTUNE_RXMODE"=250, "REG_RF_RXRFANTTUNE_TXMODE"=251, "REG_RF_RXRFANTTUNE_RXMODE"=252, "REG_ANTMATCH1"=253, "REG_ANTMATCH2"=254, "REG_REVISION_P2"=255] ("Register")
                    # "Apply 2.45 Antenna Tune value"
                    # "Address"
                    # "Bitmask"
                    n54 = And(x=w251, y=u8 15 ("Data")) -> (x .and. y?=w246:u8)
                    n55 = call "JTAG SPI.vi"("Value"=w246, "error in (no error)"=w249, "Target"=w244, "Function"=w245, "Address"=w247) -> ("error out"=w248:errorcluster)  [unwired: 3 in, 3 out]
                  }
                  frame 3 {
                    w255 = u16 215 items=["---MANUAL ENTRY---"=1000, "REG_NOREG"=0, "REG_RXBUFF_USED"=1, "REG_RXBUFF_BSIZE"=2, "REG_TXBUFF_USED"=3, "REG_TXBUFF_BSIZE"=4, "REG_TXBUFF_MAXPACKSIZE"=5, "REG_MAC_ERRCLR"=6, "REG_MAC_TRAINNUM"=7, "REG_MAC_SYNCMATCH"=8, "REG_MAC_SYNC1"=9, "REG_MAC_SYNC2"=10, "REG_MAC_SYNC3"=11, "REG_MAC_SYNC4"=12, "REG_MAC_SYNC5"=13, "REG_MAC_MAXBERR"=14, "REG_MAC_ECCORR"=15, "REG_MAC_CRCERR"=16, "REG_MAC_BLKCNT1"=17, "REG_MAC_BLKCNT2"=18, "REG_MAC_IMDTRANSID1"=19, "REG_MAC_IMDTRANSID2"=20, "REG_MAC_IMDTRANSID3"=21, "REG_MAC_COMPANYID"=22, "REG_MAC_MODUSER"=23, "REG_MAC_CHANNEL"=25, "REG_MAC_CLEARWDOG"=26, "REG_MAC_CKCORRTHRESH"=27, "REG_HK_TXADDR"=28, "REG_HK_TXDATA"=29, "REG_HK_TXREPLY"=30, "REG_HK_USERDATA"=31, "REG_HK_USERSTATUS"=32, "REG_HK_LASTADDRESS"=33, "REG_HK_MODE"=34, "REG_MAC_STATUSSEQ"=35, "REG_MAC_MAXRETRIES"=36, "REG_MAC_RESENDTIME"=37, "REG_MAC_POWERSAVETIME"=38, "REG_MAC_HEAD_DET"=39, "REG_MAC_CTRL"=41, "REG_MAC_INITCOM"=42, "REG_INTERFACE_MODE"=43, "REG_TXRXBUFF_BOTH"=44, "REG_TXRXBUFF"=45, "REG_IRQ_RAWSTATUS1"=46, "REG_IRQ_ENABLE1"=47, "REG_IRQ_ENABLESET1"=48, "REG_IRQ_ENABLECLEAR1"=49, "REG_IRQ_RAWSTATUS2"=50, "REG_IRQ_ENABLE2"=51, "REG_IRQ_ENABLESET2"=52, "REG_IRQ_ENABLECLEAR2"=53, "REG_IRQ_STATUS1"=54, "REG_IRQ_STATUS2"=55, "REG_IRQ_AUXSTATUS"=56, "REG_TXBUFF_OVERFLOW"=57, "REG_PO0"=58, "REG_P01"=59, "REG_P02"=60, "REG_P03"=61, "REG_GP0"=62, "REG_GPI"=63, "REG_WAKEUP_245IN"=64, "REG_WAKEUP_COMPANYID"=65, "REG_WAKEUP_IMDTRANSID1"=66, "REG_WAKEUP_IMDTRANSID2"=67, "REG_WAKEUP_IMDTRANSID3"=68, "REG_WAKEUP_CHANNEL"=69, "REG_WAKEUP_MODUSER"=70, "REG_WAKEUP_DEVICEMODE"=71, "REG_WAKEUP_WK_RX_CTRL1"=72, "REG_WAKEUP_STACK_ADDR"=73, "REG_WAKEUP_CTRL"=74, "REG_WAKEUP_STROSCRTRIM"=75, "REG_WAKEUP_BIASTRIM"=76, "REG_WAKEUP_ANT245TUNE"=77, "REG_WAKEUP_WK_RX_RTRIMDET"=78, "REG_WAKEUP_WK_RX_RTRIMDEMOD"=79, "REG_WAKEUP_WK_RX_RSSIGAIN"=80, "REG_WAKEUP_LNAFREQ1"=81, "REG_WAKEUP_STACK"=83, "REG_WAKUP_XOSU"=84, "REG_WAKUP_CNTDROPOUT"=85, "REG_WAKEUP_CRCCTRL"=86, "REG_WAKEUP_CRCWORD1"=87, "REG_WAKEUP_CRCWORD2"=88, "REG_WAKEUP_WK_RX_CTRIM"=89, "REG_WAKEUP_VDDATRIM"=90, "REG_WAKEUP_VDDDTRIM"=91, "REG_WAKEUP_TESTIOBUFEN"=92, "REG_WAKEUP_TESTIOCLAMP"=93, "CORE_RESET_ADDRESS"=94, "CHIP_RESET_ADDRESS"=95, "REG_RF_TXGENCTRL"=96, "REG_RF_TXIFCTRL"=97, "REG_RF_TXRF_SEL_CTRL"=98, "REG_RF_TXRFPWRDEFAULTSET"=99, "REG_RF_RSSITRIM"=100, "REG_RF_TXIFOSCTUNE"=101, "REG_RF_TXIFGAINIMB"=102, "REG_RF_TXIFLOCK"=103, "REG_RF_RXRFLNAGAINTRIM"=104, "REG_RF_RXBIASTR"=105, "REG_RF_RXGENCTRL"=106, "REG_RF_RXIFADCDECLEV"=107, "REG_RF_RXIFDETFILTERTUNE"=108, "REG_RF_RXIFFILTERTUNE"=109, "REG_RF_GENENABLES"=110, "REG_RF_SYNTH_CHANNEL"=111, "REG_TX_RAMP_RTRIM"=112, "REG_TX_RAMP_CTRIM"=113, "REG_RF_XO_TRIM"=114, "REG_RF_SYNTH_SET_TRIM"=115, "REG_RF_ADCCTRL"=116, "REG_RF_ADCOUTPUT"=117, "REG_RF_TXIFAMP"=118, "REG_RF_SYNTH_RTRIM"=119, "REG_RF_SYNTH_CTRIM"=120, "REG_RF_SYNTH_CT"=121, "REG_RF_TXMIXER_IOSTRIM_HIGH_IP"=122, "REG_RF_TXMIXER_IOSTRIM_HIGH_IN"=123, "REG_RF_TXMIXER_IOSTRIM_HIGH_QP"=124, "REG_RF_TXMIXER_IOSTRIM_HIGH_QN"=125, "REG_HX_WUADDR"=126, "REG_REVISION"=127, "REG_NOREG_TEST"=128, "REG_DTEST_RXBUFF"=129, "REG_RXBUFF_NEXT_BLOCK"=130, "REG_RXBUFF_FIRST_IN_PACK"=131, "REG_RXBUFF_FIRST_EMPTY"=132, "REG_MAC_BYPASS"=133, "REG_DTEST_TXBUFF"=134, "REG_TXBUFF_NEXT_BLOCK"=135, "REG_TXBUFF_FIRST_IN_PACK"=136, "REG_TXBUFF_FIRST_EMPTY"=137, "REG_DTEST_SEQ"=138, "REG_DTEST_CKCORR"=139, "REG_MAC_TOPSTATE"=140, "REG_DTEST_INTERFACE"=141, "REG_IFACE_TXRX_BYPASS"=142, "REG_MAC_TXRXWAIT"=143, "REG_MAC_TXRFRAMP"=144, "REG_MAC_TRAINWORD"=145, "REG_MAC_TRAINWORD2"=146, "REG_MAC_SETTINGS"=147, "REG_MAC_CALSELECT1"=148, "REG_MAC_CALSELECT2"=149, "REG_MAC_ANTMATCHSEL"=150, "REG_MAC_ANTTUNESEL1"=151, "REG_MAC_ANTTUNESEL2"=152, "REG_MAC_ANTTUNESEL3"=153, "REG_MAC_ANTTUNESTEP"=154, "REG_MAC_WUMODEBURST"=156, "REG_MAC_WUOFFSHORT"=157, "REG_MAC_WUOFFLONG"=158, "REG_MAC_CLKRECCTRL"=159, "REG_HK_MODE_P2"=162, "REG_MAC_ANTTUNERES1"=164, "REG_MAC_ANTTUNERES2"=165, "REG_INTERFACE_MODE_TEST"=171, "REG_TXRXBUFF_BOTH_P2"=172, "REG_TXRXBUFF_P2"=173, "REG_IRQ_RAWSTATUS1_P2"=174, "REG_MAC_TXIFSTATUS1"=176, "REG_MAC_TXIFSTATUS2"=177, "REG_IRQ_RAWSTATUS2_P2"=178, "REG_MAC_TXIFRAMPDELAY"=179, "REG_MAC_TXIFRAMPSLOPE"=180, "REG_MAX_TXIFRAMP"=181, "REG_IRQ_STATUS1_P2"=182, "REG_IRQ_STATUS2_P2"=183, "REG_IRQ_AUXSTATUS_P2"=184, "REG_MAC_UNLOCK"=188, "REG_MAC_TXIFFREQ"=190, "REG_WAKEUP_TESTCTRL1"=192, "REG_WAKEUP_RX_EN_CNT"=193, "REG_WAKEUP_TESTENABLES"=194, "REG_WAKEUP_DTBI_CTRL"=195, "REG_WAKEUP_DTBO_CTRL"=196, "REG_WAKEUP_TESTIOBUFTEST"=197, "REG_WAKEUP_WK_RX_TESTCTRL1"=198, "REG_WAKEUP_WK_RX_TESTCTRL2"=199, "REG_WAKEUP_SENS_SEQUENCE_CTRL"=200, "REG_WAKEUP_LNABIAS"=201, "REG_WAKEUP_DET_TH_TRIM1"=202, "REG_WAKEUP_LNABIAS_NOM1"=203, "REG_WAKEUP_RX_TSHORT_TRIM1"=204, "REG_WAKEUP_LNABIAS_NOM2"=205, "REG_WAKEUP_RX_TLONG_TRIM1"=206, "REG_WAKEUP_LNA_NEGRTRIM_NOM1"=207, "REG_WAKEUP_RX_TBURST_TRIM1"=208, "REG_WAKEUP_RX_LNA_NEGRTRIM_NOM2"=209, "REG_WAKEUP_RX_BB_G_BW_SEL1"=210, "REG_WAKEUP_WK_RX_DET_IOSTRIM1"=212, "REG_WAKEUP_WK_RX_CTRL2"=214, "REG_WAKEUP_WK_RX_RSSIVOSTRIM"=215, "REG_WAKEUP_LNANEGR_EFF"=216, "REG_WAKEUP_XOSU_FAST"=217, "REG_WAKEUP_STROSCPWIDTH1"=218, "REG_WAKEUP_STROSCPERIOD1"=220, "REG_WAKEUP_STROSCPERIOD2"=221, "REG_WAKEUP_WK_RX_LNA_NEGRTRIM1"=222, "REG_RF_TXTESTENABLE"=224, "REG_RF_TXIFTESTMODE"=225, "REG_RF_RXTESTENABLE"=226, "REG_RF_RXIFTESTCTRL1"=227, "REG_RF_RXIFTESTCTRL2"=228, "REG_RF_RXIFTESTCTRL3"=229, "REG_RF_SYNTH_TESTCTRL1"=230, "REG_RF_SYNTH_TESTCTRL2"=231, "REG_RF_SYNTH_TESTCTRL3"=232, "REG_RF_ADCTEST1"=237, "REG_RF_ADCTEST2"=238, "REG_RF_TXMIXER_IOSTRIM_LOW_IP"=240, "REG_RF_TXMIXER_IOSTRIM_LOW_IN"=241, "REG_RF_TXMIXER_ISOTRIM_LOW_QP"=242, "REG_RF_TXMIXER_IOSTRIM_LOW_QN"=243, "REG_RF_SYNTH_KPD"=244, "REG_RF_SYNTH_LOLEV"=245, "REG_RF_TXRFPWRTUNEANTSET"=246, "REG_RF_TXPD_GAIN_CTRL"=247, "REG_RF_SYNTH_STARTUP"=248, "REG_RF_TXRFANTTUNE_TXMODE"=249, "REG_RF_TXRFANTTUNE_RXMODE"=250, "REG_RF_RXRFANTTUNE_TXMODE"=251, "REG_RF_RXRFANTTUNE_RXMODE"=252, "REG_ANTMATCH1"=253, "REG_ANTMATCH2"=254, "REG_REVISION_P2"=255] ("Register")
                    # "Shift \"Baseband Gain\" value left by two bits, apply to BW_SEL1 register with 0x1C Bitmask"
                    # "Address"
                    # "Bitmask"
                    n56 = And(x=w258, y=u8 31 ("Data")) -> (x .and. y?=w254:u8)
                    n57 = call "JTAG SPI.vi"("Value"=w254, "error in (no error)"=w257, "Target"=w252, "Function"=w253, "Address"=w255) -> ("error out"=w256:errorcluster)  [unwired: 3 in, 3 out]
                  }
                  frame 4 {
                    w263 = u16 212 items=["---MANUAL ENTRY---"=1000, "REG_NOREG"=0, "REG_RXBUFF_USED"=1, "REG_RXBUFF_BSIZE"=2, "REG_TXBUFF_USED"=3, "REG_TXBUFF_BSIZE"=4, "REG_TXBUFF_MAXPACKSIZE"=5, "REG_MAC_ERRCLR"=6, "REG_MAC_TRAINNUM"=7, "REG_MAC_SYNCMATCH"=8, "REG_MAC_SYNC1"=9, "REG_MAC_SYNC2"=10, "REG_MAC_SYNC3"=11, "REG_MAC_SYNC4"=12, "REG_MAC_SYNC5"=13, "REG_MAC_MAXBERR"=14, "REG_MAC_ECCORR"=15, "REG_MAC_CRCERR"=16, "REG_MAC_BLKCNT1"=17, "REG_MAC_BLKCNT2"=18, "REG_MAC_IMDTRANSID1"=19, "REG_MAC_IMDTRANSID2"=20, "REG_MAC_IMDTRANSID3"=21, "REG_MAC_COMPANYID"=22, "REG_MAC_MODUSER"=23, "REG_MAC_CHANNEL"=25, "REG_MAC_CLEARWDOG"=26, "REG_MAC_CKCORRTHRESH"=27, "REG_HK_TXADDR"=28, "REG_HK_TXDATA"=29, "REG_HK_TXREPLY"=30, "REG_HK_USERDATA"=31, "REG_HK_USERSTATUS"=32, "REG_HK_LASTADDRESS"=33, "REG_HK_MODE"=34, "REG_MAC_STATUSSEQ"=35, "REG_MAC_MAXRETRIES"=36, "REG_MAC_RESENDTIME"=37, "REG_MAC_POWERSAVETIME"=38, "REG_MAC_HEAD_DET"=39, "REG_MAC_CTRL"=41, "REG_MAC_INITCOM"=42, "REG_INTERFACE_MODE"=43, "REG_TXRXBUFF_BOTH"=44, "REG_TXRXBUFF"=45, "REG_IRQ_RAWSTATUS1"=46, "REG_IRQ_ENABLE1"=47, "REG_IRQ_ENABLESET1"=48, "REG_IRQ_ENABLECLEAR1"=49, "REG_IRQ_RAWSTATUS2"=50, "REG_IRQ_ENABLE2"=51, "REG_IRQ_ENABLESET2"=52, "REG_IRQ_ENABLECLEAR2"=53, "REG_IRQ_STATUS1"=54, "REG_IRQ_STATUS2"=55, "REG_IRQ_AUXSTATUS"=56, "REG_TXBUFF_OVERFLOW"=57, "REG_PO0"=58, "REG_P01"=59, "REG_P02"=60, "REG_P03"=61, "REG_GP0"=62, "REG_GPI"=63, "REG_WAKEUP_245IN"=64, "REG_WAKEUP_COMPANYID"=65, "REG_WAKEUP_IMDTRANSID1"=66, "REG_WAKEUP_IMDTRANSID2"=67, "REG_WAKEUP_IMDTRANSID3"=68, "REG_WAKEUP_CHANNEL"=69, "REG_WAKEUP_MODUSER"=70, "REG_WAKEUP_DEVICEMODE"=71, "REG_WAKEUP_WK_RX_CTRL1"=72, "REG_WAKEUP_STACK_ADDR"=73, "REG_WAKEUP_CTRL"=74, "REG_WAKEUP_STROSCRTRIM"=75, "REG_WAKEUP_BIASTRIM"=76, "REG_WAKEUP_ANT245TUNE"=77, "REG_WAKEUP_WK_RX_RTRIMDET"=78, "REG_WAKEUP_WK_RX_RTRIMDEMOD"=79, "REG_WAKEUP_WK_RX_RSSIGAIN"=80, "REG_WAKEUP_LNAFREQ1"=81, "REG_WAKEUP_STACK"=83, "REG_WAKUP_XOSU"=84, "REG_WAKUP_CNTDROPOUT"=85, "REG_WAKEUP_CRCCTRL"=86, "REG_WAKEUP_CRCWORD1"=87, "REG_WAKEUP_CRCWORD2"=88, "REG_WAKEUP_WK_RX_CTRIM"=89, "REG_WAKEUP_VDDATRIM"=90, "REG_WAKEUP_VDDDTRIM"=91, "REG_WAKEUP_TESTIOBUFEN"=92, "REG_WAKEUP_TESTIOCLAMP"=93, "CORE_RESET_ADDRESS"=94, "CHIP_RESET_ADDRESS"=95, "REG_RF_TXGENCTRL"=96, "REG_RF_TXIFCTRL"=97, "REG_RF_TXRF_SEL_CTRL"=98, "REG_RF_TXRFPWRDEFAULTSET"=99, "REG_RF_RSSITRIM"=100, "REG_RF_TXIFOSCTUNE"=101, "REG_RF_TXIFGAINIMB"=102, "REG_RF_TXIFLOCK"=103, "REG_RF_RXRFLNAGAINTRIM"=104, "REG_RF_RXBIASTR"=105, "REG_RF_RXGENCTRL"=106, "REG_RF_RXIFADCDECLEV"=107, "REG_RF_RXIFDETFILTERTUNE"=108, "REG_RF_RXIFFILTERTUNE"=109, "REG_RF_GENENABLES"=110, "REG_RF_SYNTH_CHANNEL"=111, "REG_TX_RAMP_RTRIM"=112, "REG_TX_RAMP_CTRIM"=113, "REG_RF_XO_TRIM"=114, "REG_RF_SYNTH_SET_TRIM"=115, "REG_RF_ADCCTRL"=116, "REG_RF_ADCOUTPUT"=117, "REG_RF_TXIFAMP"=118, "REG_RF_SYNTH_RTRIM"=119, "REG_RF_SYNTH_CTRIM"=120, "REG_RF_SYNTH_CT"=121, "REG_RF_TXMIXER_IOSTRIM_HIGH_IP"=122, "REG_RF_TXMIXER_IOSTRIM_HIGH_IN"=123, "REG_RF_TXMIXER_IOSTRIM_HIGH_QP"=124, "REG_RF_TXMIXER_IOSTRIM_HIGH_QN"=125, "REG_HX_WUADDR"=126, "REG_REVISION"=127, "REG_NOREG_TEST"=128, "REG_DTEST_RXBUFF"=129, "REG_RXBUFF_NEXT_BLOCK"=130, "REG_RXBUFF_FIRST_IN_PACK"=131, "REG_RXBUFF_FIRST_EMPTY"=132, "REG_MAC_BYPASS"=133, "REG_DTEST_TXBUFF"=134, "REG_TXBUFF_NEXT_BLOCK"=135, "REG_TXBUFF_FIRST_IN_PACK"=136, "REG_TXBUFF_FIRST_EMPTY"=137, "REG_DTEST_SEQ"=138, "REG_DTEST_CKCORR"=139, "REG_MAC_TOPSTATE"=140, "REG_DTEST_INTERFACE"=141, "REG_IFACE_TXRX_BYPASS"=142, "REG_MAC_TXRXWAIT"=143, "REG_MAC_TXRFRAMP"=144, "REG_MAC_TRAINWORD"=145, "REG_MAC_TRAINWORD2"=146, "REG_MAC_SETTINGS"=147, "REG_MAC_CALSELECT1"=148, "REG_MAC_CALSELECT2"=149, "REG_MAC_ANTMATCHSEL"=150, "REG_MAC_ANTTUNESEL1"=151, "REG_MAC_ANTTUNESEL2"=152, "REG_MAC_ANTTUNESEL3"=153, "REG_MAC_ANTTUNESTEP"=154, "REG_MAC_WUMODEBURST"=156, "REG_MAC_WUOFFSHORT"=157, "REG_MAC_WUOFFLONG"=158, "REG_MAC_CLKRECCTRL"=159, "REG_HK_MODE_P2"=162, "REG_MAC_ANTTUNERES1"=164, "REG_MAC_ANTTUNERES2"=165, "REG_INTERFACE_MODE_TEST"=171, "REG_TXRXBUFF_BOTH_P2"=172, "REG_TXRXBUFF_P2"=173, "REG_IRQ_RAWSTATUS1_P2"=174, "REG_MAC_TXIFSTATUS1"=176, "REG_MAC_TXIFSTATUS2"=177, "REG_IRQ_RAWSTATUS2_P2"=178, "REG_MAC_TXIFRAMPDELAY"=179, "REG_MAC_TXIFRAMPSLOPE"=180, "REG_MAX_TXIFRAMP"=181, "REG_IRQ_STATUS1_P2"=182, "REG_IRQ_STATUS2_P2"=183, "REG_IRQ_AUXSTATUS_P2"=184, "REG_MAC_UNLOCK"=188, "REG_MAC_TXIFFREQ"=190, "REG_WAKEUP_TESTCTRL1"=192, "REG_WAKEUP_RX_EN_CNT"=193, "REG_WAKEUP_TESTENABLES"=194, "REG_WAKEUP_DTBI_CTRL"=195, "REG_WAKEUP_DTBO_CTRL"=196, "REG_WAKEUP_TESTIOBUFTEST"=197, "REG_WAKEUP_WK_RX_TESTCTRL1"=198, "REG_WAKEUP_WK_RX_TESTCTRL2"=199, "REG_WAKEUP_SENS_SEQUENCE_CTRL"=200, "REG_WAKEUP_LNABIAS"=201, "REG_WAKEUP_DET_TH_TRIM1"=202, "REG_WAKEUP_LNABIAS_NOM1"=203, "REG_WAKEUP_RX_TSHORT_TRIM1"=204, "REG_WAKEUP_LNABIAS_NOM2"=205, "REG_WAKEUP_RX_TLONG_TRIM1"=206, "REG_WAKEUP_LNA_NEGRTRIM_NOM1"=207, "REG_WAKEUP_RX_TBURST_TRIM1"=208, "REG_WAKEUP_RX_LNA_NEGRTRIM_NOM2"=209, "REG_WAKEUP_RX_BB_G_BW_SEL1"=210, "REG_WAKEUP_WK_RX_DET_IOSTRIM1"=212, "REG_WAKEUP_WK_RX_CTRL2"=214, "REG_WAKEUP_WK_RX_RSSIVOSTRIM"=215, "REG_WAKEUP_LNANEGR_EFF"=216, "REG_WAKEUP_XOSU_FAST"=217, "REG_WAKEUP_STROSCPWIDTH1"=218, "REG_WAKEUP_STROSCPERIOD1"=220, "REG_WAKEUP_STROSCPERIOD2"=221, "REG_WAKEUP_WK_RX_LNA_NEGRTRIM1"=222, "REG_RF_TXTESTENABLE"=224, "REG_RF_TXIFTESTMODE"=225, "REG_RF_RXTESTENABLE"=226, "REG_RF_RXIFTESTCTRL1"=227, "REG_RF_RXIFTESTCTRL2"=228, "REG_RF_RXIFTESTCTRL3"=229, "REG_RF_SYNTH_TESTCTRL1"=230, "REG_RF_SYNTH_TESTCTRL2"=231, "REG_RF_SYNTH_TESTCTRL3"=232, "REG_RF_ADCTEST1"=237, "REG_RF_ADCTEST2"=238, "REG_RF_TXMIXER_IOSTRIM_LOW_IP"=240, "REG_RF_TXMIXER_IOSTRIM_LOW_IN"=241, "REG_RF_TXMIXER_ISOTRIM_LOW_QP"=242, "REG_RF_TXMIXER_IOSTRIM_LOW_QN"=243, "REG_RF_SYNTH_KPD"=244, "REG_RF_SYNTH_LOLEV"=245, "REG_RF_TXRFPWRTUNEANTSET"=246, "REG_RF_TXPD_GAIN_CTRL"=247, "REG_RF_SYNTH_STARTUP"=248, "REG_RF_TXRFANTTUNE_TXMODE"=249, "REG_RF_TXRFANTTUNE_RXMODE"=250, "REG_RF_RXRFANTTUNE_TXMODE"=251, "REG_RF_RXRFANTTUNE_RXMODE"=252, "REG_ANTMATCH1"=253, "REG_ANTMATCH2"=254, "REG_REVISION_P2"=255] ("Register")
                    # "Apply Detector Trim Value"
                    # "Address"
                    # "Bitmask"
                    n58 = And(x=w266, y=u8 63 ("Data")) -> (x .and. y?=w262:u8)
                    n59 = call "JTAG SPI.vi"("Value"=w262, "error in (no error)"=w265, "Target"=w260, "Function"=w261, "Address"=w263) -> ("error out"=w264:errorcluster)  [unwired: 3 in, 3 out]
                  }
                  frame 5 {
                    w272 = u16 80 items=["---MANUAL ENTRY---"=1000, "REG_NOREG"=0, "REG_RXBUFF_USED"=1, "REG_RXBUFF_BSIZE"=2, "REG_TXBUFF_USED"=3, "REG_TXBUFF_BSIZE"=4, "REG_TXBUFF_MAXPACKSIZE"=5, "REG_MAC_ERRCLR"=6, "REG_MAC_TRAINNUM"=7, "REG_MAC_SYNCMATCH"=8, "REG_MAC_SYNC1"=9, "REG_MAC_SYNC2"=10, "REG_MAC_SYNC3"=11, "REG_MAC_SYNC4"=12, "REG_MAC_SYNC5"=13, "REG_MAC_MAXBERR"=14, "REG_MAC_ECCORR"=15, "REG_MAC_CRCERR"=16, "REG_MAC_BLKCNT1"=17, "REG_MAC_BLKCNT2"=18, "REG_MAC_IMDTRANSID1"=19, "REG_MAC_IMDTRANSID2"=20, "REG_MAC_IMDTRANSID3"=21, "REG_MAC_COMPANYID"=22, "REG_MAC_MODUSER"=23, "REG_MAC_CHANNEL"=25, "REG_MAC_CLEARWDOG"=26, "REG_MAC_CKCORRTHRESH"=27, "REG_HK_TXADDR"=28, "REG_HK_TXDATA"=29, "REG_HK_TXREPLY"=30, "REG_HK_USERDATA"=31, "REG_HK_USERSTATUS"=32, "REG_HK_LASTADDRESS"=33, "REG_HK_MODE"=34, "REG_MAC_STATUSSEQ"=35, "REG_MAC_MAXRETRIES"=36, "REG_MAC_RESENDTIME"=37, "REG_MAC_POWERSAVETIME"=38, "REG_MAC_HEAD_DET"=39, "REG_MAC_CTRL"=41, "REG_MAC_INITCOM"=42, "REG_INTERFACE_MODE"=43, "REG_TXRXBUFF_BOTH"=44, "REG_TXRXBUFF"=45, "REG_IRQ_RAWSTATUS1"=46, "REG_IRQ_ENABLE1"=47, "REG_IRQ_ENABLESET1"=48, "REG_IRQ_ENABLECLEAR1"=49, "REG_IRQ_RAWSTATUS2"=50, "REG_IRQ_ENABLE2"=51, "REG_IRQ_ENABLESET2"=52, "REG_IRQ_ENABLECLEAR2"=53, "REG_IRQ_STATUS1"=54, "REG_IRQ_STATUS2"=55, "REG_IRQ_AUXSTATUS"=56, "REG_TXBUFF_OVERFLOW"=57, "REG_PO0"=58, "REG_P01"=59, "REG_P02"=60, "REG_P03"=61, "REG_GP0"=62, "REG_GPI"=63, "REG_WAKEUP_245IN"=64, "REG_WAKEUP_COMPANYID"=65, "REG_WAKEUP_IMDTRANSID1"=66, "REG_WAKEUP_IMDTRANSID2"=67, "REG_WAKEUP_IMDTRANSID3"=68, "REG_WAKEUP_CHANNEL"=69, "REG_WAKEUP_MODUSER"=70, "REG_WAKEUP_DEVICEMODE"=71, "REG_WAKEUP_WK_RX_CTRL1"=72, "REG_WAKEUP_STACK_ADDR"=73, "REG_WAKEUP_CTRL"=74, "REG_WAKEUP_STROSCRTRIM"=75, "REG_WAKEUP_BIASTRIM"=76, "REG_WAKEUP_ANT245TUNE"=77, "REG_WAKEUP_WK_RX_RTRIMDET"=78, "REG_WAKEUP_WK_RX_RTRIMDEMOD"=79, "REG_WAKEUP_WK_RX_RSSIGAIN"=80, "REG_WAKEUP_LNAFREQ1"=81, "REG_WAKEUP_STACK"=83, "REG_WAKUP_XOSU"=84, "REG_WAKUP_CNTDROPOUT"=85, "REG_WAKEUP_CRCCTRL"=86, "REG_WAKEUP_CRCWORD1"=87, "REG_WAKEUP_CRCWORD2"=88, "REG_WAKEUP_WK_RX_CTRIM"=89, "REG_WAKEUP_VDDATRIM"=90, "REG_WAKEUP_VDDDTRIM"=91, "REG_WAKEUP_TESTIOBUFEN"=92, "REG_WAKEUP_TESTIOCLAMP"=93, "CORE_RESET_ADDRESS"=94, "CHIP_RESET_ADDRESS"=95, "REG_RF_TXGENCTRL"=96, "REG_RF_TXIFCTRL"=97, "REG_RF_TXRF_SEL_CTRL"=98, "REG_RF_TXRFPWRDEFAULTSET"=99, "REG_RF_RSSITRIM"=100, "REG_RF_TXIFOSCTUNE"=101, "REG_RF_TXIFGAINIMB"=102, "REG_RF_TXIFLOCK"=103, "REG_RF_RXRFLNAGAINTRIM"=104, "REG_RF_RXBIASTR"=105, "REG_RF_RXGENCTRL"=106, "REG_RF_RXIFADCDECLEV"=107, "REG_RF_RXIFDETFILTERTUNE"=108, "REG_RF_RXIFFILTERTUNE"=109, "REG_RF_GENENABLES"=110, "REG_RF_SYNTH_CHANNEL"=111, "REG_TX_RAMP_RTRIM"=112, "REG_TX_RAMP_CTRIM"=113, "REG_RF_XO_TRIM"=114, "REG_RF_SYNTH_SET_TRIM"=115, "REG_RF_ADCCTRL"=116, "REG_RF_ADCOUTPUT"=117, "REG_RF_TXIFAMP"=118, "REG_RF_SYNTH_RTRIM"=119, "REG_RF_SYNTH_CTRIM"=120, "REG_RF_SYNTH_CT"=121, "REG_RF_TXMIXER_IOSTRIM_HIGH_IP"=122, "REG_RF_TXMIXER_IOSTRIM_HIGH_IN"=123, "REG_RF_TXMIXER_IOSTRIM_HIGH_QP"=124, "REG_RF_TXMIXER_IOSTRIM_HIGH_QN"=125, "REG_HX_WUADDR"=126, "REG_REVISION"=127, "REG_NOREG_TEST"=128, "REG_DTEST_RXBUFF"=129, "REG_RXBUFF_NEXT_BLOCK"=130, "REG_RXBUFF_FIRST_IN_PACK"=131, "REG_RXBUFF_FIRST_EMPTY"=132, "REG_MAC_BYPASS"=133, "REG_DTEST_TXBUFF"=134, "REG_TXBUFF_NEXT_BLOCK"=135, "REG_TXBUFF_FIRST_IN_PACK"=136, "REG_TXBUFF_FIRST_EMPTY"=137, "REG_DTEST_SEQ"=138, "REG_DTEST_CKCORR"=139, "REG_MAC_TOPSTATE"=140, "REG_DTEST_INTERFACE"=141, "REG_IFACE_TXRX_BYPASS"=142, "REG_MAC_TXRXWAIT"=143, "REG_MAC_TXRFRAMP"=144, "REG_MAC_TRAINWORD"=145, "REG_MAC_TRAINWORD2"=146, "REG_MAC_SETTINGS"=147, "REG_MAC_CALSELECT1"=148, "REG_MAC_CALSELECT2"=149, "REG_MAC_ANTMATCHSEL"=150, "REG_MAC_ANTTUNESEL1"=151, "REG_MAC_ANTTUNESEL2"=152, "REG_MAC_ANTTUNESEL3"=153, "REG_MAC_ANTTUNESTEP"=154, "REG_MAC_WUMODEBURST"=156, "REG_MAC_WUOFFSHORT"=157, "REG_MAC_WUOFFLONG"=158, "REG_MAC_CLKRECCTRL"=159, "REG_HK_MODE_P2"=162, "REG_MAC_ANTTUNERES1"=164, "REG_MAC_ANTTUNERES2"=165, "REG_INTERFACE_MODE_TEST"=171, "REG_TXRXBUFF_BOTH_P2"=172, "REG_TXRXBUFF_P2"=173, "REG_IRQ_RAWSTATUS1_P2"=174, "REG_MAC_TXIFSTATUS1"=176, "REG_MAC_TXIFSTATUS2"=177, "REG_IRQ_RAWSTATUS2_P2"=178, "REG_MAC_TXIFRAMPDELAY"=179, "REG_MAC_TXIFRAMPSLOPE"=180, "REG_MAX_TXIFRAMP"=181, "REG_IRQ_STATUS1_P2"=182, "REG_IRQ_STATUS2_P2"=183, "REG_IRQ_AUXSTATUS_P2"=184, "REG_MAC_UNLOCK"=188, "REG_MAC_TXIFFREQ"=190, "REG_WAKEUP_TESTCTRL1"=192, "REG_WAKEUP_RX_EN_CNT"=193, "REG_WAKEUP_TESTENABLES"=194, "REG_WAKEUP_DTBI_CTRL"=195, "REG_WAKEUP_DTBO_CTRL"=196, "REG_WAKEUP_TESTIOBUFTEST"=197, "REG_WAKEUP_WK_RX_TESTCTRL1"=198, "REG_WAKEUP_WK_RX_TESTCTRL2"=199, "REG_WAKEUP_SENS_SEQUENCE_CTRL"=200, "REG_WAKEUP_LNABIAS"=201, "REG_WAKEUP_DET_TH_TRIM1"=202, "REG_WAKEUP_LNABIAS_NOM1"=203, "REG_WAKEUP_RX_TSHORT_TRIM1"=204, "REG_WAKEUP_LNABIAS_NOM2"=205, "REG_WAKEUP_RX_TLONG_TRIM1"=206, "REG_WAKEUP_LNA_NEGRTRIM_NOM1"=207, "REG_WAKEUP_RX_TBURST_TRIM1"=208, "REG_WAKEUP_RX_LNA_NEGRTRIM_NOM2"=209, "REG_WAKEUP_RX_BB_G_BW_SEL1"=210, "REG_WAKEUP_WK_RX_DET_IOSTRIM1"=212, "REG_WAKEUP_WK_RX_CTRL2"=214, "REG_WAKEUP_WK_RX_RSSIVOSTRIM"=215, "REG_WAKEUP_LNANEGR_EFF"=216, "REG_WAKEUP_XOSU_FAST"=217, "REG_WAKEUP_STROSCPWIDTH1"=218, "REG_WAKEUP_STROSCPERIOD1"=220, "REG_WAKEUP_STROSCPERIOD2"=221, "REG_WAKEUP_WK_RX_LNA_NEGRTRIM1"=222, "REG_RF_TXTESTENABLE"=224, "REG_RF_TXIFTESTMODE"=225, "REG_RF_RXTESTENABLE"=226, "REG_RF_RXIFTESTCTRL1"=227, "REG_RF_RXIFTESTCTRL2"=228, "REG_RF_RXIFTESTCTRL3"=229, "REG_RF_SYNTH_TESTCTRL1"=230, "REG_RF_SYNTH_TESTCTRL2"=231, "REG_RF_SYNTH_TESTCTRL3"=232, "REG_RF_ADCTEST1"=237, "REG_RF_ADCTEST2"=238, "REG_RF_TXMIXER_IOSTRIM_LOW_IP"=240, "REG_RF_TXMIXER_IOSTRIM_LOW_IN"=241, "REG_RF_TXMIXER_ISOTRIM_LOW_QP"=242, "REG_RF_TXMIXER_IOSTRIM_LOW_QN"=243, "REG_RF_SYNTH_KPD"=244, "REG_RF_SYNTH_LOLEV"=245, "REG_RF_TXRFPWRTUNEANTSET"=246, "REG_RF_TXPD_GAIN_CTRL"=247, "REG_RF_SYNTH_STARTUP"=248, "REG_RF_TXRFANTTUNE_TXMODE"=249, "REG_RF_TXRFANTTUNE_RXMODE"=250, "REG_RF_RXRFANTTUNE_TXMODE"=251, "REG_RF_RXRFANTTUNE_RXMODE"=252, "REG_ANTMATCH1"=253, "REG_ANTMATCH2"=254, "REG_REVISION_P2"=255] ("Register")
                    # "Apply RSSI Gain Value"
                    # "Address"
                    # "Bitmask"
                    n60 = And(x=w268, y=u8 3 ("Data")) -> (x .and. y?=w271:u16)
                    n61 = call "JTAG SPI.vi"("Value"=w271, "error in (no error)"=w274, "Target"=w269, "Function"=w270, "Address"=w272) -> ("error out"=w273:errorcluster)  [unwired: 3 in, 3 out]
                  }
                }
              }
              n62 = call "JTAG SPI.vi"("Value"=u8 1 ("Data"), "error in (no error)"=w195, "Target"=w189, "Function"=w190, "Address"=w187) -> ("error out"=w194:errorcluster)  [unwired: 3 in, 3 out]
              n63 = call "Simple Wait.vi"("mS"=u32 20, "error in"=w194) -> ("error out"=w191:errorcluster)  [unwired: 12 in, 1 out]
              n64 = call "JTAG SPI.vi"("Value"=u8 0 ("Data"), "error in (no error)"=w191, "Target"=w189, "Function"=w190, "Address"=w187) -> ("error out"=w192:errorcluster)  [unwired: 3 in, 3 out]
            }
          }
        }
        frame 2 {
          # "Update the CW RF Source Settings"
          n65 = Not Equal?(x="Wakeup Signal Transmit", y=w291) -> (x != y?=w290:bool)
          n66 = case shown="False" w290 {
            tunnel: w289 -> [w310 w317]
            tunnel: w288 -> [w308 w316]
            tunnel: [w310 w314] -> w285
            tunnel: "Wakeup Signal Transmit" -> [_ w315]
            tunnel: w282 -> [_ w313]
            tunnel: w281 -> [w309 _]
            tunnel: [w309 42.0 ("Wakeup Signal Power, dBm")] -> w280
            tunnel: [w308 w311] -> w279
            frame False {
              # "No change to 2.45GHz CW Carrier status, carry on"
            }
            frame True {
              n67 = case shown="True" w315 {
                tunnel: w317 -> [w320 w326]
                tunnel: w316 -> [w319 w322]
                tunnel: [w318 w327] -> w314
                tunnel: w313 -> [_ w324]
                tunnel: [w319 w322] -> w311
                frame False {
                  # "Force Attenuator Update after Reset"
                  # "Disable 2.45GHz CW Carrier"
                  n68 = call "MICSD Reset.vi"("error in (no error)"=w320, "VISA Resource Name"=w319) -> ("error out"=w318:errorcluster)  [unwired: 8 in, 1 out]
                }
                frame True {
                  # "Force Attenuator Update"
                  n69 = call "MICSD Config.vi"("error in (no error)"=w326, "Function"=enum16{"Write Config", "Read Config"}."Write Config", "MICS_Config_In"=w324, "VISA Resource Name"=w322) -> ("error out"=w325:errorcluster)  [unwired: 5 in, 2 out]
                  n70 = case shown="False" "WakeupRF" {
                    tunnel: [w332 w337] -> w327
                    tunnel: w325 -> [w331 w334]
                    tunnel: w322 -> [w330 w333]
                    frame False {
                      # "Enable 2.45GHz Wakeup\n(pulsed packets), \"Search\nfor Implant\" mode"
                      n71 = call "MICSD Search for Implant.vi"("VISA Resource Name"=w330, "Enable Watchdog?(T)"=FALSE, "error in (no error)"=w331, "Mode"=T2."Start Search") -> ("error out"=w332:errorcluster)  [unwired: 8 in, 3 out]
                    }
                    frame True {
                      w335 = TRUE  # TX Mode (Off)
                      # "Enable 2.45GHz CW \nCarrier at 10dBm"
                      n72 = call "MICSD CW Carrier.vi"("error in (no error)"=w334, "TX Mode (Off)"=w335, "Frequency Range"=enum16{"2.45GHz", "400MHz"}."2.45GHz", "VISA Resource Name"=w333) -> ("error out"=w337:errorcluster)  [unwired: 6 in, 1 out]
                    }
                  }
                }
              }
            }
          }
          n73 = Not Equal?(x="Wakeup Signal Power, dBm", y=w280) -> (x != y?=w287:bool)
          n74 = And(x="Wakeup Signal Transmit", y=w287) -> (x .and. y?=w284:bool)
          n75 = case shown="True" w284 {
            tunnel: w285 -> [w298 w306]
            tunnel: "Wakeup Signal Power, dBm" -> [_ w307]
            tunnel: w279 -> [_ w300]
            tunnel: [w298 w305] -> w278
            frame False {
              # "No update to RF Attenuator value"
            }
            frame True {
              # "RF Attenuator value needs to be updated, do it."
              n76 = Absolute Value(x=w307) -> (abs(x)=w304:dbl)
              n77 = Multiply(x=4.0, y=w304) -> (x*y=w303:dbl)
              n78 = To Unsigned Byte Integer(number=w303) -> (unsigned 8bit integer=w301:u8)
              n79 = call "MICSD Set Attenuator.vi"("error in (no error)"=w306, "Attenuation"=w301, "VISA Resource Name"=w300) -> ("error out"=w305:errorcluster)  [unwired: 7 in, 1 out]
              n80 = Wait (ms)(milliseconds to wait=u32 50) -> ()  [unwired: 1 out]
            }
          }
        }
        frame 3 {
          n81 = case shown="True" "Do RSSI" {
            tunnel: w344 -> [w355 w361]
            tunnel: [w355 w362] -> w343
            tunnel: [u8 0 w358] -> w342
            tunnel: w341 -> [_ w357]
            tunnel: w340 -> [_ w356]
            frame False {
              # "RSSI Measurement not enabled"
            }
            frame True {
              # "Perform 2.45GHz RX RSSI Measurement"
              n82 = for {
                N: "Samples to Average" -> [_]
                tunnel: [w384] -> w364 mode=indexing
                shift-right: [w365] -> w362
                shift-left: w361 -> [w381]
                tunnel: w357 -> [w376]
                tunnel: w356 -> [w372]
                w371 = u16 3 items=["Power UP", "Power DN", "Write Single", "Read Single", "Write Block", "Read Block", "Write Masked", "Test Value"] ("Function")
                w374 = u16 117 items=["---MANUAL ENTRY---"=1000, "REG_NOREG"=0, "REG_RXBUFF_USED"=1, "REG_RXBUFF_BSIZE"=2, "REG_TXBUFF_USED"=3, "REG_TXBUFF_BSIZE"=4, "REG_TXBUFF_MAXPACKSIZE"=5, "REG_MAC_ERRCLR"=6, "REG_MAC_TRAINNUM"=7, "REG_MAC_SYNCMATCH"=8, "REG_MAC_SYNC1"=9, "REG_MAC_SYNC2"=10, "REG_MAC_SYNC3"=11, "REG_MAC_SYNC4"=12, "REG_MAC_SYNC5"=13, "REG_MAC_MAXBERR"=14, "REG_MAC_ECCORR"=15, "REG_MAC_CRCERR"=16, "REG_MAC_BLKCNT1"=17, "REG_MAC_BLKCNT2"=18, "REG_MAC_IMDTRANSID1"=19, "REG_MAC_IMDTRANSID2"=20, "REG_MAC_IMDTRANSID3"=21, "REG_MAC_COMPANYID"=22, "REG_MAC_MODUSER"=23, "REG_MAC_CHANNEL"=25, "REG_MAC_CLEARWDOG"=26, "REG_MAC_CKCORRTHRESH"=27, "REG_HK_TXADDR"=28, "REG_HK_TXDATA"=29, "REG_HK_TXREPLY"=30, "REG_HK_USERDATA"=31, "REG_HK_USERSTATUS"=32, "REG_HK_LASTADDRESS"=33, "REG_HK_MODE"=34, "REG_MAC_STATUSSEQ"=35, "REG_MAC_MAXRETRIES"=36, "REG_MAC_RESENDTIME"=37, "REG_MAC_POWERSAVETIME"=38, "REG_MAC_HEAD_DET"=39, "REG_MAC_CTRL"=41, "REG_MAC_INITCOM"=42, "REG_INTERFACE_MODE"=43, "REG_TXRXBUFF_BOTH"=44, "REG_TXRXBUFF"=45, "REG_IRQ_RAWSTATUS1"=46, "REG_IRQ_ENABLE1"=47, "REG_IRQ_ENABLESET1"=48, "REG_IRQ_ENABLECLEAR1"=49, "REG_IRQ_RAWSTATUS2"=50, "REG_IRQ_ENABLE2"=51, "REG_IRQ_ENABLESET2"=52, "REG_IRQ_ENABLECLEAR2"=53, "REG_IRQ_STATUS1"=54, "REG_IRQ_STATUS2"=55, "REG_IRQ_AUXSTATUS"=56, "REG_TXBUFF_OVERFLOW"=57, "REG_PO0"=58, "REG_P01"=59, "REG_P02"=60, "REG_P03"=61, "REG_GP0"=62, "REG_GPI"=63, "REG_WAKEUP_245IN"=64, "REG_WAKEUP_COMPANYID"=65, "REG_WAKEUP_IMDTRANSID1"=66, "REG_WAKEUP_IMDTRANSID2"=67, "REG_WAKEUP_IMDTRANSID3"=68, "REG_WAKEUP_CHANNEL"=69, "REG_WAKEUP_MODUSER"=70, "REG_WAKEUP_DEVICEMODE"=71, "REG_WAKEUP_WK_RX_CTRL1"=72, "REG_WAKEUP_STACK_ADDR"=73, "REG_WAKEUP_CTRL"=74, "REG_WAKEUP_STROSCRTRIM"=75, "REG_WAKEUP_BIASTRIM"=76, "REG_WAKEUP_ANT245TUNE"=77, "REG_WAKEUP_WK_RX_RTRIMDET"=78, "REG_WAKEUP_WK_RX_RTRIMDEMOD"=79, "REG_WAKEUP_WK_RX_RSSIGAIN"=80, "REG_WAKEUP_LNAFREQ1"=81, "REG_WAKEUP_STACK"=83, "REG_WAKUP_XOSU"=84, "REG_WAKUP_CNTDROPOUT"=85, "REG_WAKEUP_CRCCTRL"=86, "REG_WAKEUP_CRCWORD1"=87, "REG_WAKEUP_CRCWORD2"=88, "REG_WAKEUP_WK_RX_CTRIM"=89, "REG_WAKEUP_VDDATRIM"=90, "REG_WAKEUP_VDDDTRIM"=91, "REG_WAKEUP_TESTIOBUFEN"=92, "REG_WAKEUP_TESTIOCLAMP"=93, "CORE_RESET_ADDRESS"=94, "CHIP_RESET_ADDRESS"=95, "REG_RF_TXGENCTRL"=96, "REG_RF_TXIFCTRL"=97, "REG_RF_TXRF_SEL_CTRL"=98, "REG_RF_TXRFPWRDEFAULTSET"=99, "REG_RF_RSSITRIM"=100, "REG_RF_TXIFOSCTUNE"=101, "REG_RF_TXIFGAINIMB"=102, "REG_RF_TXIFLOCK"=103, "REG_RF_RXRFLNAGAINTRIM"=104, "REG_RF_RXBIASTR"=105, "REG_RF_RXGENCTRL"=106, "REG_RF_RXIFADCDECLEV"=107, "REG_RF_RXIFDETFILTERTUNE"=108, "REG_RF_RXIFFILTERTUNE"=109, "REG_RF_GENENABLES"=110, "REG_RF_SYNTH_CHANNEL"=111, "REG_TX_RAMP_RTRIM"=112, "REG_TX_RAMP_CTRIM"=113, "REG_RF_XO_TRIM"=114, "REG_RF_SYNTH_SET_TRIM"=115, "REG_RF_ADCCTRL"=116, "REG_RF_ADCOUTPUT"=117, "REG_RF_TXIFAMP"=118, "REG_RF_SYNTH_RTRIM"=119, "REG_RF_SYNTH_CTRIM"=120, "REG_RF_SYNTH_CT"=121, "REG_RF_TXMIXER_IOSTRIM_HIGH_IP"=122, "REG_RF_TXMIXER_IOSTRIM_HIGH_IN"=123, "REG_RF_TXMIXER_IOSTRIM_HIGH_QP"=124, "REG_RF_TXMIXER_IOSTRIM_HIGH_QN"=125, "REG_HX_WUADDR"=126, "REG_REVISION"=127, "REG_NOREG_TEST"=128, "REG_DTEST_RXBUFF"=129, "REG_RXBUFF_NEXT_BLOCK"=130, "REG_RXBUFF_FIRST_IN_PACK"=131, "REG_RXBUFF_FIRST_EMPTY"=132, "REG_MAC_BYPASS"=133, "REG_DTEST_TXBUFF"=134, "REG_TXBUFF_NEXT_BLOCK"=135, "REG_TXBUFF_FIRST_IN_PACK"=136, "REG_TXBUFF_FIRST_EMPTY"=137, "REG_DTEST_SEQ"=138, "REG_DTEST_CKCORR"=139, "REG_MAC_TOPSTATE"=140, "REG_DTEST_INTERFACE"=141, "REG_IFACE_TXRX_BYPASS"=142, "REG_MAC_TXRXWAIT"=143, "REG_MAC_TXRFRAMP"=144, "REG_MAC_TRAINWORD"=145, "REG_MAC_TRAINWORD2"=146, "REG_MAC_SETTINGS"=147, "REG_MAC_CALSELECT1"=148, "REG_MAC_CALSELECT2"=149, "REG_MAC_ANTMATCHSEL"=150, "REG_MAC_ANTTUNESEL1"=151, "REG_MAC_ANTTUNESEL2"=152, "REG_MAC_ANTTUNESEL3"=153, "REG_MAC_ANTTUNESTEP"=154, "REG_MAC_WUMODEBURST"=156, "REG_MAC_WUOFFSHORT"=157, "REG_MAC_WUOFFLONG"=158, "REG_MAC_CLKRECCTRL"=159, "REG_HK_MODE_P2"=162, "REG_MAC_ANTTUNERES1"=164, "REG_MAC_ANTTUNERES2"=165, "REG_INTERFACE_MODE_TEST"=171, "REG_TXRXBUFF_BOTH_P2"=172, "REG_TXRXBUFF_P2"=173, "REG_IRQ_RAWSTATUS1_P2"=174, "REG_MAC_TXIFSTATUS1"=176, "REG_MAC_TXIFSTATUS2"=177, "REG_IRQ_RAWSTATUS2_P2"=178, "REG_MAC_TXIFRAMPDELAY"=179, "REG_MAC_TXIFRAMPSLOPE"=180, "REG_MAX_TXIFRAMP"=181, "REG_IRQ_STATUS1_P2"=182, "REG_IRQ_STATUS2_P2"=183, "REG_IRQ_AUXSTATUS_P2"=184, "REG_MAC_UNLOCK"=188, "REG_MAC_TXIFFREQ"=190, "REG_WAKEUP_TESTCTRL1"=192, "REG_WAKEUP_RX_EN_CNT"=193, "REG_WAKEUP_TESTENABLES"=194, "REG_WAKEUP_DTBI_CTRL"=195, "REG_WAKEUP_DTBO_CTRL"=196, "REG_WAKEUP_TESTIOBUFTEST"=197, "REG_WAKEUP_WK_RX_TESTCTRL1"=198, "REG_WAKEUP_WK_RX_TESTCTRL2"=199, "REG_WAKEUP_SENS_SEQUENCE_CTRL"=200, "REG_WAKEUP_LNABIAS"=201, "REG_WAKEUP_DET_TH_TRIM1"=202, "REG_WAKEUP_LNABIAS_NOM1"=203, "REG_WAKEUP_RX_TSHORT_TRIM1"=204, "REG_WAKEUP_LNABIAS_NOM2"=205, "REG_WAKEUP_RX_TLONG_TRIM1"=206, "REG_WAKEUP_LNA_NEGRTRIM_NOM1"=207, "REG_WAKEUP_RX_TBURST_TRIM1"=208, "REG_WAKEUP_RX_LNA_NEGRTRIM_NOM2"=209, "REG_WAKEUP_RX_BB_G_BW_SEL1"=210, "REG_WAKEUP_WK_RX_DET_IOSTRIM1"=212, "REG_WAKEUP_WK_RX_CTRL2"=214, "REG_WAKEUP_WK_RX_RSSIVOSTRIM"=215, "REG_WAKEUP_LNANEGR_EFF"=216, "REG_WAKEUP_XOSU_FAST"=217, "REG_WAKEUP_STROSCPWIDTH1"=218, "REG_WAKEUP_STROSCPERIOD1"=220, "REG_WAKEUP_STROSCPERIOD2"=221, "REG_WAKEUP_WK_RX_LNA_NEGRTRIM1"=222, "REG_RF_TXTESTENABLE"=224, "REG_RF_TXIFTESTMODE"=225, "REG_RF_RXTESTENABLE"=226, "REG_RF_RXIFTESTCTRL1"=227, "REG_RF_RXIFTESTCTRL2"=228, "REG_RF_RXIFTESTCTRL3"=229, "REG_RF_SYNTH_TESTCTRL1"=230, "REG_RF_SYNTH_TESTCTRL2"=231, "REG_RF_SYNTH_TESTCTRL3"=232, "REG_RF_ADCTEST1"=237, "REG_RF_ADCTEST2"=238, "REG_RF_TXMIXER_IOSTRIM_LOW_IP"=240, "REG_RF_TXMIXER_IOSTRIM_LOW_IN"=241, "REG_RF_TXMIXER_ISOTRIM_LOW_QP"=242, "REG_RF_TXMIXER_IOSTRIM_LOW_QN"=243, "REG_RF_SYNTH_KPD"=244, "REG_RF_SYNTH_LOLEV"=245, "REG_RF_TXRFPWRTUNEANTSET"=246, "REG_RF_TXPD_GAIN_CTRL"=247, "REG_RF_SYNTH_STARTUP"=248, "REG_RF_TXRFANTTUNE_TXMODE"=249, "REG_RF_TXRFANTTUNE_RXMODE"=250, "REG_RF_RXRFANTTUNE_TXMODE"=251, "REG_RF_RXRFANTTUNE_RXMODE"=252, "REG_ANTMATCH1"=253, "REG_ANTMATCH2"=254, "REG_REVISION_P2"=255] ("Register")
                w378 = u16 116 items=["---MANUAL ENTRY---"=1000, "REG_NOREG"=0, "REG_RXBUFF_USED"=1, "REG_RXBUFF_BSIZE"=2, "REG_TXBUFF_USED"=3, "REG_TXBUFF_BSIZE"=4, "REG_TXBUFF_MAXPACKSIZE"=5, "REG_MAC_ERRCLR"=6, "REG_MAC_TRAINNUM"=7, "REG_MAC_SYNCMATCH"=8, "REG_MAC_SYNC1"=9, "REG_MAC_SYNC2"=10, "REG_MAC_SYNC3"=11, "REG_MAC_SYNC4"=12, "REG_MAC_SYNC5"=13, "REG_MAC_MAXBERR"=14, "REG_MAC_ECCORR"=15, "REG_MAC_CRCERR"=16, "REG_MAC_BLKCNT1"=17, "REG_MAC_BLKCNT2"=18, "REG_MAC_IMDTRANSID1"=19, "REG_MAC_IMDTRANSID2"=20, "REG_MAC_IMDTRANSID3"=21, "REG_MAC_COMPANYID"=22, "REG_MAC_MODUSER"=23, "REG_MAC_CHANNEL"=25, "REG_MAC_CLEARWDOG"=26, "REG_MAC_CKCORRTHRESH"=27, "REG_HK_TXADDR"=28, "REG_HK_TXDATA"=29, "REG_HK_TXREPLY"=30, "REG_HK_USERDATA"=31, "REG_HK_USERSTATUS"=32, "REG_HK_LASTADDRESS"=33, "REG_HK_MODE"=34, "REG_MAC_STATUSSEQ"=35, "REG_MAC_MAXRETRIES"=36, "REG_MAC_RESENDTIME"=37, "REG_MAC_POWERSAVETIME"=38, "REG_MAC_HEAD_DET"=39, "REG_MAC_CTRL"=41, "REG_MAC_INITCOM"=42, "REG_INTERFACE_MODE"=43, "REG_TXRXBUFF_BOTH"=44, "REG_TXRXBUFF"=45, "REG_IRQ_RAWSTATUS1"=46, "REG_IRQ_ENABLE1"=47, "REG_IRQ_ENABLESET1"=48, "REG_IRQ_ENABLECLEAR1"=49, "REG_IRQ_RAWSTATUS2"=50, "REG_IRQ_ENABLE2"=51, "REG_IRQ_ENABLESET2"=52, "REG_IRQ_ENABLECLEAR2"=53, "REG_IRQ_STATUS1"=54, "REG_IRQ_STATUS2"=55, "REG_IRQ_AUXSTATUS"=56, "REG_TXBUFF_OVERFLOW"=57, "REG_PO0"=58, "REG_P01"=59, "REG_P02"=60, "REG_P03"=61, "REG_GP0"=62, "REG_GPI"=63, "REG_WAKEUP_245IN"=64, "REG_WAKEUP_COMPANYID"=65, "REG_WAKEUP_IMDTRANSID1"=66, "REG_WAKEUP_IMDTRANSID2"=67, "REG_WAKEUP_IMDTRANSID3"=68, "REG_WAKEUP_CHANNEL"=69, "REG_WAKEUP_MODUSER"=70, "REG_WAKEUP_DEVICEMODE"=71, "REG_WAKEUP_WK_RX_CTRL1"=72, "REG_WAKEUP_STACK_ADDR"=73, "REG_WAKEUP_CTRL"=74, "REG_WAKEUP_STROSCRTRIM"=75, "REG_WAKEUP_BIASTRIM"=76, "REG_WAKEUP_ANT245TUNE"=77, "REG_WAKEUP_WK_RX_RTRIMDET"=78, "REG_WAKEUP_WK_RX_RTRIMDEMOD"=79, "REG_WAKEUP_WK_RX_RSSIGAIN"=80, "REG_WAKEUP_LNAFREQ1"=81, "REG_WAKEUP_STACK"=83, "REG_WAKUP_XOSU"=84, "REG_WAKUP_CNTDROPOUT"=85, "REG_WAKEUP_CRCCTRL"=86, "REG_WAKEUP_CRCWORD1"=87, "REG_WAKEUP_CRCWORD2"=88, "REG_WAKEUP_WK_RX_CTRIM"=89, "REG_WAKEUP_VDDATRIM"=90, "REG_WAKEUP_VDDDTRIM"=91, "REG_WAKEUP_TESTIOBUFEN"=92, "REG_WAKEUP_TESTIOCLAMP"=93, "CORE_RESET_ADDRESS"=94, "CHIP_RESET_ADDRESS"=95, "REG_RF_TXGENCTRL"=96, "REG_RF_TXIFCTRL"=97, "REG_RF_TXRF_SEL_CTRL"=98, "REG_RF_TXRFPWRDEFAULTSET"=99, "REG_RF_RSSITRIM"=100, "REG_RF_TXIFOSCTUNE"=101, "REG_RF_TXIFGAINIMB"=102, "REG_RF_TXIFLOCK"=103, "REG_RF_RXRFLNAGAINTRIM"=104, "REG_RF_RXBIASTR"=105, "REG_RF_RXGENCTRL"=106, "REG_RF_RXIFADCDECLEV"=107, "REG_RF_RXIFDETFILTERTUNE"=108, "REG_RF_RXIFFILTERTUNE"=109, "REG_RF_GENENABLES"=110, "REG_RF_SYNTH_CHANNEL"=111, "REG_TX_RAMP_RTRIM"=112, "REG_TX_RAMP_CTRIM"=113, "REG_RF_XO_TRIM"=114, "REG_RF_SYNTH_SET_TRIM"=115, "REG_RF_ADCCTRL"=116, "REG_RF_ADCOUTPUT"=117, "REG_RF_TXIFAMP"=118, "REG_RF_SYNTH_RTRIM"=119, "REG_RF_SYNTH_CTRIM"=120, "REG_RF_SYNTH_CT"=121, "REG_RF_TXMIXER_IOSTRIM_HIGH_IP"=122, "REG_RF_TXMIXER_IOSTRIM_HIGH_IN"=123, "REG_RF_TXMIXER_IOSTRIM_HIGH_QP"=124, "REG_RF_TXMIXER_IOSTRIM_HIGH_QN"=125, "REG_HX_WUADDR"=126, "REG_REVISION"=127, "REG_NOREG_TEST"=128, "REG_DTEST_RXBUFF"=129, "REG_RXBUFF_NEXT_BLOCK"=130, "REG_RXBUFF_FIRST_IN_PACK"=131, "REG_RXBUFF_FIRST_EMPTY"=132, "REG_MAC_BYPASS"=133, "REG_DTEST_TXBUFF"=134, "REG_TXBUFF_NEXT_BLOCK"=135, "REG_TXBUFF_FIRST_IN_PACK"=136, "REG_TXBUFF_FIRST_EMPTY"=137, "REG_DTEST_SEQ"=138, "REG_DTEST_CKCORR"=139, "REG_MAC_TOPSTATE"=140, "REG_DTEST_INTERFACE"=141, "REG_IFACE_TXRX_BYPASS"=142, "REG_MAC_TXRXWAIT"=143, "REG_MAC_TXRFRAMP"=144, "REG_MAC_TRAINWORD"=145, "REG_MAC_TRAINWORD2"=146, "REG_MAC_SETTINGS"=147, "REG_MAC_CALSELECT1"=148, "REG_MAC_CALSELECT2"=149, "REG_MAC_ANTMATCHSEL"=150, "REG_MAC_ANTTUNESEL1"=151, "REG_MAC_ANTTUNESEL2"=152, "REG_MAC_ANTTUNESEL3"=153, "REG_MAC_ANTTUNESTEP"=154, "REG_MAC_WUMODEBURST"=156, "REG_MAC_WUOFFSHORT"=157, "REG_MAC_WUOFFLONG"=158, "REG_MAC_CLKRECCTRL"=159, "REG_HK_MODE_P2"=162, "REG_MAC_ANTTUNERES1"=164, "REG_MAC_ANTTUNERES2"=165, "REG_INTERFACE_MODE_TEST"=171, "REG_TXRXBUFF_BOTH_P2"=172, "REG_TXRXBUFF_P2"=173, "REG_IRQ_RAWSTATUS1_P2"=174, "REG_MAC_TXIFSTATUS1"=176, "REG_MAC_TXIFSTATUS2"=177, "REG_IRQ_RAWSTATUS2_P2"=178, "REG_MAC_TXIFRAMPDELAY"=179, "REG_MAC_TXIFRAMPSLOPE"=180, "REG_MAX_TXIFRAMP"=181, "REG_IRQ_STATUS1_P2"=182, "REG_IRQ_STATUS2_P2"=183, "REG_IRQ_AUXSTATUS_P2"=184, "REG_MAC_UNLOCK"=188, "REG_MAC_TXIFFREQ"=190, "REG_WAKEUP_TESTCTRL1"=192, "REG_WAKEUP_RX_EN_CNT"=193, "REG_WAKEUP_TESTENABLES"=194, "REG_WAKEUP_DTBI_CTRL"=195, "REG_WAKEUP_DTBO_CTRL"=196, "REG_WAKEUP_TESTIOBUFTEST"=197, "REG_WAKEUP_WK_RX_TESTCTRL1"=198, "REG_WAKEUP_WK_RX_TESTCTRL2"=199, "REG_WAKEUP_SENS_SEQUENCE_CTRL"=200, "REG_WAKEUP_LNABIAS"=201, "REG_WAKEUP_DET_TH_TRIM1"=202, "REG_WAKEUP_LNABIAS_NOM1"=203, "REG_WAKEUP_RX_TSHORT_TRIM1"=204, "REG_WAKEUP_LNABIAS_NOM2"=205, "REG_WAKEUP_RX_TLONG_TRIM1"=206, "REG_WAKEUP_LNA_NEGRTRIM_NOM1"=207, "REG_WAKEUP_RX_TBURST_TRIM1"=208, "REG_WAKEUP_RX_LNA_NEGRTRIM_NOM2"=209, "REG_WAKEUP_RX_BB_G_BW_SEL1"=210, "REG_WAKEUP_WK_RX_DET_IOSTRIM1"=212, "REG_WAKEUP_WK_RX_CTRL2"=214, "REG_WAKEUP_WK_RX_RSSIVOSTRIM"=215, "REG_WAKEUP_LNANEGR_EFF"=216, "REG_WAKEUP_XOSU_FAST"=217, "REG_WAKEUP_STROSCPWIDTH1"=218, "REG_WAKEUP_STROSCPERIOD1"=220, "REG_WAKEUP_STROSCPERIOD2"=221, "REG_WAKEUP_WK_RX_LNA_NEGRTRIM1"=222, "REG_RF_TXTESTENABLE"=224, "REG_RF_TXIFTESTMODE"=225, "REG_RF_RXTESTENABLE"=226, "REG_RF_RXIFTESTCTRL1"=227, "REG_RF_RXIFTESTCTRL2"=228, "REG_RF_RXIFTESTCTRL3"=229, "REG_RF_SYNTH_TESTCTRL1"=230, "REG_RF_SYNTH_TESTCTRL2"=231, "REG_RF_SYNTH_TESTCTRL3"=232, "REG_RF_ADCTEST1"=237, "REG_RF_ADCTEST2"=238, "REG_RF_TXMIXER_IOSTRIM_LOW_IP"=240, "REG_RF_TXMIXER_IOSTRIM_LOW_IN"=241, "REG_RF_TXMIXER_ISOTRIM_LOW_QP"=242, "REG_RF_TXMIXER_IOSTRIM_LOW_QN"=243, "REG_RF_SYNTH_KPD"=244, "REG_RF_SYNTH_LOLEV"=245, "REG_RF_TXRFPWRTUNEANTSET"=246, "REG_RF_TXPD_GAIN_CTRL"=247, "REG_RF_SYNTH_STARTUP"=248, "REG_RF_TXRFANTTUNE_TXMODE"=249, "REG_RF_TXRFANTTUNE_RXMODE"=250, "REG_RF_RXRFANTTUNE_TXMODE"=251, "REG_RF_RXRFANTTUNE_RXMODE"=252, "REG_ANTMATCH1"=253, "REG_ANTMATCH2"=254, "REG_REVISION_P2"=255] ("Register")
                n83 = call "JTAG SPI.vi"("Value"=u8 29 ("Data"), "error in (no error)"=w381, "Target"=w372, "Function"=w376, "Address"=w378) -> ("error out"=w369:errorcluster)  [unwired: 3 in, 3 out]
                n84 = call "Simple Wait.vi"("mS"=u32 10, "error in"=w369) -> ("error out"=w368:errorcluster)  [unwired: 12 in, 1 out]
                n85 = call "JTAG SPI.vi"("Value"=u8 31 ("Data"), "error in (no error)"=w368, "Target"=w372, "Function"=w376, "Address"=w378) -> ("error out"=w379:errorcluster)  [unwired: 3 in, 3 out]
                n86 = call "Simple Wait.vi"("mS"=u32 50, "error in"=w379) -> ("error out"=w375:errorcluster)  [unwired: 12 in, 1 out]
                n87 = call "JTAG SPI.vi"("error in (no error)"=w375, "Target"=w372, "Function"=w371, "Address"=w374) -> ("error out"=w366:errorcluster, "Read Value"=w373:u8)  [unwired: 4 in, 2 out]
                "RSSI" <- w373
                n88 = To Long Integer(number=w373) -> (32bit integer=w382:i32)
                n89 = call "Simple Wait.vi"("mS"=u32 10, "error in"=w366) -> ("error out"=w365:errorcluster)  [unwired: 12 in, 1 out]
                n90 = Subtract(x=w382, y=32) -> (x-y=w384:i32)
              }
              n91 = Add Array Elements(numeric array=w364) -> (sum=w363:i32)
              n92 = Quotient & Remainder(x=w363, y="Samples to Average") -> (floor(x/y)=w359:i32)  [unwired: 1 out]
              n93 = To Unsigned Byte Integer(number=w359) -> (unsigned 8bit integer=w358:u8)
            }
          }
          "RSSI Reading" <- w342
        }
        frame 4 {
          n94 = Format Into String(format string="Address=0x0051 {LNA Freq Trim}\r\nData=0x%02x\r\nAddress=0x00DE {LNA Gain Trim}\r\nData=0x%02x\r\nAddress=0x004D {2.45 Antenna Tune}\r\nData=0x%02x\r\nAddress=0x00D7 {RSSI Fine Trim}\r\nData=0x%02x\r\nAddress 0x00D4 {Detector Offset Trim}\r\nData=0x%02x", w393, w392, w391, w388, w390) -> (resulting string=→"Trim Settings":string)  [unwired: 2 in, 1 out]
        }
        frame 5 {
          n95 = Not Equal?(x=w403, y="Loopback Detector") -> (x != y?=w402:bool)
          n96 = case shown="True" w402 {
            tunnel: w401 -> [w414 w417]
            tunnel: [w414 w416] -> w400
            tunnel: "Loopback Detector" -> [_ w415]
            frame False {
            }
            frame True {
              n97 = case shown="False" w415 {
                tunnel: w417 -> [w423 w430]
                tunnel: [w422 w429] -> w416
                frame True {
                  w418 = u16 6 items=["Power UP", "Power DN", "Write Single", "Read Single", "Write Block", "Read Block", "Write Masked", "Test Value"] ("Function")
                  w419 = u16 2 items=["Power ASIC", "Stim ASIC", "MICS Radio", "FRAM"] ("Target")
                  w420 = u8 9 ("Data")
                  w421 = u16 74 items=["---MANUAL ENTRY---"=1000, "REG_NOREG"=0, "REG_RXBUFF_USED"=1, "REG_RXBUFF_BSIZE"=2, "REG_TXBUFF_USED"=3, "REG_TXBUFF_BSIZE"=4, "REG_TXBUFF_MAXPACKSIZE"=5, "REG_MAC_ERRCLR"=6, "REG_MAC_TRAINNUM"=7, "REG_MAC_SYNCMATCH"=8, "REG_MAC_SYNC1"=9, "REG_MAC_SYNC2"=10, "REG_MAC_SYNC3"=11, "REG_MAC_SYNC4"=12, "REG_MAC_SYNC5"=13, "REG_MAC_MAXBERR"=14, "REG_MAC_ECCORR"=15, "REG_MAC_CRCERR"=16, "REG_MAC_BLKCNT1"=17, "REG_MAC_BLKCNT2"=18, "REG_MAC_IMDTRANSID1"=19, "REG_MAC_IMDTRANSID2"=20, "REG_MAC_IMDTRANSID3"=21, "REG_MAC_COMPANYID"=22, "REG_MAC_MODUSER"=23, "REG_MAC_CHANNEL"=25, "REG_MAC_CLEARWDOG"=26, "REG_MAC_CKCORRTHRESH"=27, "REG_HK_TXADDR"=28, "REG_HK_TXDATA"=29, "REG_HK_TXREPLY"=30, "REG_HK_USERDATA"=31, "REG_HK_USERSTATUS"=32, "REG_HK_LASTADDRESS"=33, "REG_HK_MODE"=34, "REG_MAC_STATUSSEQ"=35, "REG_MAC_MAXRETRIES"=36, "REG_MAC_RESENDTIME"=37, "REG_MAC_POWERSAVETIME"=38, "REG_MAC_HEAD_DET"=39, "REG_MAC_CTRL"=41, "REG_MAC_INITCOM"=42, "REG_INTERFACE_MODE"=43, "REG_TXRXBUFF_BOTH"=44, "REG_TXRXBUFF"=45, "REG_IRQ_RAWSTATUS1"=46, "REG_IRQ_ENABLE1"=47, "REG_IRQ_ENABLESET1"=48, "REG_IRQ_ENABLECLEAR1"=49, "REG_IRQ_RAWSTATUS2"=50, "REG_IRQ_ENABLE2"=51, "REG_IRQ_ENABLESET2"=52, "REG_IRQ_ENABLECLEAR2"=53, "REG_IRQ_STATUS1"=54, "REG_IRQ_STATUS2"=55, "REG_IRQ_AUXSTATUS"=56, "REG_TXBUFF_OVERFLOW"=57, "REG_PO0"=58, "REG_P01"=59, "REG_P02"=60, "REG_P03"=61, "REG_GP0"=62, "REG_GPI"=63, "REG_WAKEUP_245IN"=64, "REG_WAKEUP_COMPANYID"=65, "REG_WAKEUP_IMDTRANSID1"=66, "REG_WAKEUP_IMDTRANSID2"=67, "REG_WAKEUP_IMDTRANSID3"=68, "REG_WAKEUP_CHANNEL"=69, "REG_WAKEUP_MODUSER"=70, "REG_WAKEUP_DEVICEMODE"=71, "REG_WAKEUP_WK_RX_CTRL1"=72, "REG_WAKEUP_STACK_ADDR"=73, "REG_WAKEUP_CTRL"=74, "REG_WAKEUP_STROSCRTRIM"=75, "REG_WAKEUP_BIASTRIM"=76, "REG_WAKEUP_ANT245TUNE"=77, "REG_WAKEUP_WK_RX_RTRIMDET"=78, "REG_WAKEUP_WK_RX_RTRIMDEMOD"=79, "REG_WAKEUP_WK_RX_RSSIGAIN"=80, "REG_WAKEUP_LNAFREQ1"=81, "REG_WAKEUP_STACK"=83, "REG_WAKUP_XOSU"=84, "REG_WAKUP_CNTDROPOUT"=85, "REG_WAKEUP_CRCCTRL"=86, "REG_WAKEUP_CRCWORD1"=87, "REG_WAKEUP_CRCWORD2"=88, "REG_WAKEUP_WK_RX_CTRIM"=89, "REG_WAKEUP_VDDATRIM"=90, "REG_WAKEUP_VDDDTRIM"=91, "REG_WAKEUP_TESTIOBUFEN"=92, "REG_WAKEUP_TESTIOCLAMP"=93, "CORE_RESET_ADDRESS"=94, "CHIP_RESET_ADDRESS"=95, "REG_RF_TXGENCTRL"=96, "REG_RF_TXIFCTRL"=97, "REG_RF_TXRF_SEL_CTRL"=98, "REG_RF_TXRFPWRDEFAULTSET"=99, "REG_RF_RSSITRIM"=100, "REG_RF_TXIFOSCTUNE"=101, "REG_RF_TXIFGAINIMB"=102, "REG_RF_TXIFLOCK"=103, "REG_RF_RXRFLNAGAINTRIM"=104, "REG_RF_RXBIASTR"=105, "REG_RF_RXGENCTRL"=106, "REG_RF_RXIFADCDECLEV"=107, "REG_RF_RXIFDETFILTERTUNE"=108, "REG_RF_RXIFFILTERTUNE"=109, "REG_RF_GENENABLES"=110, "REG_RF_SYNTH_CHANNEL"=111, "REG_TX_RAMP_RTRIM"=112, "REG_TX_RAMP_CTRIM"=113, "REG_RF_XO_TRIM"=114, "REG_RF_SYNTH_SET_TRIM"=115, "REG_RF_ADCCTRL"=116, "REG_RF_ADCOUTPUT"=117, "REG_RF_TXIFAMP"=118, "REG_RF_SYNTH_RTRIM"=119, "REG_RF_SYNTH_CTRIM"=120, "REG_RF_SYNTH_CT"=121, "REG_RF_TXMIXER_IOSTRIM_HIGH_IP"=122, "REG_RF_TXMIXER_IOSTRIM_HIGH_IN"=123, "REG_RF_TXMIXER_IOSTRIM_HIGH_QP"=124, "REG_RF_TXMIXER_IOSTRIM_HIGH_QN"=125, "REG_HX_WUADDR"=126, "REG_REVISION"=127, "REG_NOREG_TEST"=128, "REG_DTEST_RXBUFF"=129, "REG_RXBUFF_NEXT_BLOCK"=130, "REG_RXBUFF_FIRST_IN_PACK"=131, "REG_RXBUFF_FIRST_EMPTY"=132, "REG_MAC_BYPASS"=133, "REG_DTEST_TXBUFF"=134, "REG_TXBUFF_NEXT_BLOCK"=135, "REG_TXBUFF_FIRST_IN_PACK"=136, "REG_TXBUFF_FIRST_EMPTY"=137, "REG_DTEST_SEQ"=138, "REG_DTEST_CKCORR"=139, "REG_MAC_TOPSTATE"=140, "REG_DTEST_INTERFACE"=141, "REG_IFACE_TXRX_BYPASS"=142, "REG_MAC_TXRXWAIT"=143, "REG_MAC_TXRFRAMP"=144, "REG_MAC_TRAINWORD"=145, "REG_MAC_TRAINWORD2"=146, "REG_MAC_SETTINGS"=147, "REG_MAC_CALSELECT1"=148, "REG_MAC_CALSELECT2"=149, "REG_MAC_ANTMATCHSEL"=150, "REG_MAC_ANTTUNESEL1"=151, "REG_MAC_ANTTUNESEL2"=152, "REG_MAC_ANTTUNESEL3"=153, "REG_MAC_ANTTUNESTEP"=154, "REG_MAC_WUMODEBURST"=156, "REG_MAC_WUOFFSHORT"=157, "REG_MAC_WUOFFLONG"=158, "REG_MAC_CLKRECCTRL"=159, "REG_HK_MODE_P2"=162, "REG_MAC_ANTTUNERES1"=164, "REG_MAC_ANTTUNERES2"=165, "REG_INTERFACE_MODE_TEST"=171, "REG_TXRXBUFF_BOTH_P2"=172, "REG_TXRXBUFF_P2"=173, "REG_IRQ_RAWSTATUS1_P2"=174, "REG_MAC_TXIFSTATUS1"=176, "REG_MAC_TXIFSTATUS2"=177, "REG_IRQ_RAWSTATUS2_P2"=178, "REG_MAC_TXIFRAMPDELAY"=179, "REG_MAC_TXIFRAMPSLOPE"=180, "REG_MAX_TXIFRAMP"=181, "REG_IRQ_STATUS1_P2"=182, "REG_IRQ_STATUS2_P2"=183, "REG_IRQ_AUXSTATUS_P2"=184, "REG_MAC_UNLOCK"=188, "REG_MAC_TXIFFREQ"=190, "REG_WAKEUP_TESTCTRL1"=192, "REG_WAKEUP_RX_EN_CNT"=193, "REG_WAKEUP_TESTENABLES"=194, "REG_WAKEUP_DTBI_CTRL"=195, "REG_WAKEUP_DTBO_CTRL"=196, "REG_WAKEUP_TESTIOBUFTEST"=197, "REG_WAKEUP_WK_RX_TESTCTRL1"=198, "REG_WAKEUP_WK_RX_TESTCTRL2"=199, "REG_WAKEUP_SENS_SEQUENCE_CTRL"=200, "REG_WAKEUP_LNABIAS"=201, "REG_WAKEUP_DET_TH_TRIM1"=202, "REG_WAKEUP_LNABIAS_NOM1"=203, "REG_WAKEUP_RX_TSHORT_TRIM1"=204, "REG_WAKEUP_LNABIAS_NOM2"=205, "REG_WAKEUP_RX_TLONG_TRIM1"=206, "REG_WAKEUP_LNA_NEGRTRIM_NOM1"=207, "REG_WAKEUP_RX_TBURST_TRIM1"=208, "REG_WAKEUP_RX_LNA_NEGRTRIM_NOM2"=209, "REG_WAKEUP_RX_BB_G_BW_SEL1"=210, "REG_WAKEUP_WK_RX_DET_IOSTRIM1"=212, "REG_WAKEUP_WK_RX_CTRL2"=214, "REG_WAKEUP_WK_RX_RSSIVOSTRIM"=215, "REG_WAKEUP_LNANEGR_EFF"=216, "REG_WAKEUP_XOSU_FAST"=217, "REG_WAKEUP_STROSCPWIDTH1"=218, "REG_WAKEUP_STROSCPERIOD1"=220, "REG_WAKEUP_STROSCPERIOD2"=221, "REG_WAKEUP_WK_RX_LNA_NEGRTRIM1"=222, "REG_RF_TXTESTENABLE"=224, "REG_RF_TXIFTESTMODE"=225, "REG_RF_RXTESTENABLE"=226, "REG_RF_RXIFTESTCTRL1"=227, "REG_RF_RXIFTESTCTRL2"=228, "REG_RF_RXIFTESTCTRL3"=229, "REG_RF_SYNTH_TESTCTRL1"=230, "REG_RF_SYNTH_TESTCTRL2"=231, "REG_RF_SYNTH_TESTCTRL3"=232, "REG_RF_ADCTEST1"=237, "REG_RF_ADCTEST2"=238, "REG_RF_TXMIXER_IOSTRIM_LOW_IP"=240, "REG_RF_TXMIXER_IOSTRIM_LOW_IN"=241, "REG_RF_TXMIXER_ISOTRIM_LOW_QP"=242, "REG_RF_TXMIXER_IOSTRIM_LOW_QN"=243, "REG_RF_SYNTH_KPD"=244, "REG_RF_SYNTH_LOLEV"=245, "REG_RF_TXRFPWRTUNEANTSET"=246, "REG_RF_TXPD_GAIN_CTRL"=247, "REG_RF_SYNTH_STARTUP"=248, "REG_RF_TXRFANTTUNE_TXMODE"=249, "REG_RF_TXRFANTTUNE_RXMODE"=250, "REG_RF_RXRFANTTUNE_TXMODE"=251, "REG_RF_RXRFANTTUNE_RXMODE"=252, "REG_ANTMATCH1"=253, "REG_ANTMATCH2"=254, "REG_REVISION_P2"=255] ("Register")
                  n98 = call "JTAG SPI.vi"("Mask"=w420, "Value"=w420, "error in (no error)"=w423, "Target"=w419, "Function"=w418, "Address"=w421) -> ("error out"=w422:errorcluster)  [unwired: 2 in, 3 out]
                }
                frame False {
                  w425 = u16 6 items=["Power UP", "Power DN", "Write Single", "Read Single", "Write Block", "Read Block", "Write Masked", "Test Value"] ("Function")
                  w426 = u16 2 items=["Power ASIC", "Stim ASIC", "MICS Radio", "FRAM"] ("Target")
                  w428 = u16 74 items=["---MANUAL ENTRY---"=1000, "REG_NOREG"=0, "REG_RXBUFF_USED"=1, "REG_RXBUFF_BSIZE"=2, "REG_TXBUFF_USED"=3, "REG_TXBUFF_BSIZE"=4, "REG_TXBUFF_MAXPACKSIZE"=5, "REG_MAC_ERRCLR"=6, "REG_MAC_TRAINNUM"=7, "REG_MAC_SYNCMATCH"=8, "REG_MAC_SYNC1"=9, "REG_MAC_SYNC2"=10, "REG_MAC_SYNC3"=11, "REG_MAC_SYNC4"=12, "REG_MAC_SYNC5"=13, "REG_MAC_MAXBERR"=14, "REG_MAC_ECCORR"=15, "REG_MAC_CRCERR"=16, "REG_MAC_BLKCNT1"=17, "REG_MAC_BLKCNT2"=18, "REG_MAC_IMDTRANSID1"=19, "REG_MAC_IMDTRANSID2"=20, "REG_MAC_IMDTRANSID3"=21, "REG_MAC_COMPANYID"=22, "REG_MAC_MODUSER"=23, "REG_MAC_CHANNEL"=25, "REG_MAC_CLEARWDOG"=26, "REG_MAC_CKCORRTHRESH"=27, "REG_HK_TXADDR"=28, "REG_HK_TXDATA"=29, "REG_HK_TXREPLY"=30, "REG_HK_USERDATA"=31, "REG_HK_USERSTATUS"=32, "REG_HK_LASTADDRESS"=33, "REG_HK_MODE"=34, "REG_MAC_STATUSSEQ"=35, "REG_MAC_MAXRETRIES"=36, "REG_MAC_RESENDTIME"=37, "REG_MAC_POWERSAVETIME"=38, "REG_MAC_HEAD_DET"=39, "REG_MAC_CTRL"=41, "REG_MAC_INITCOM"=42, "REG_INTERFACE_MODE"=43, "REG_TXRXBUFF_BOTH"=44, "REG_TXRXBUFF"=45, "REG_IRQ_RAWSTATUS1"=46, "REG_IRQ_ENABLE1"=47, "REG_IRQ_ENABLESET1"=48, "REG_IRQ_ENABLECLEAR1"=49, "REG_IRQ_RAWSTATUS2"=50, "REG_IRQ_ENABLE2"=51, "REG_IRQ_ENABLESET2"=52, "REG_IRQ_ENABLECLEAR2"=53, "REG_IRQ_STATUS1"=54, "REG_IRQ_STATUS2"=55, "REG_IRQ_AUXSTATUS"=56, "REG_TXBUFF_OVERFLOW"=57, "REG_PO0"=58, "REG_P01"=59, "REG_P02"=60, "REG_P03"=61, "REG_GP0"=62, "REG_GPI"=63, "REG_WAKEUP_245IN"=64, "REG_WAKEUP_COMPANYID"=65, "REG_WAKEUP_IMDTRANSID1"=66, "REG_WAKEUP_IMDTRANSID2"=67, "REG_WAKEUP_IMDTRANSID3"=68, "REG_WAKEUP_CHANNEL"=69, "REG_WAKEUP_MODUSER"=70, "REG_WAKEUP_DEVICEMODE"=71, "REG_WAKEUP_WK_RX_CTRL1"=72, "REG_WAKEUP_STACK_ADDR"=73, "REG_WAKEUP_CTRL"=74, "REG_WAKEUP_STROSCRTRIM"=75, "REG_WAKEUP_BIASTRIM"=76, "REG_WAKEUP_ANT245TUNE"=77, "REG_WAKEUP_WK_RX_RTRIMDET"=78, "REG_WAKEUP_WK_RX_RTRIMDEMOD"=79, "REG_WAKEUP_WK_RX_RSSIGAIN"=80, "REG_WAKEUP_LNAFREQ1"=81, "REG_WAKEUP_STACK"=83, "REG_WAKUP_XOSU"=84, "REG_WAKUP_CNTDROPOUT"=85, "REG_WAKEUP_CRCCTRL"=86, "REG_WAKEUP_CRCWORD1"=87, "REG_WAKEUP_CRCWORD2"=88, "REG_WAKEUP_WK_RX_CTRIM"=89, "REG_WAKEUP_VDDATRIM"=90, "REG_WAKEUP_VDDDTRIM"=91, "REG_WAKEUP_TESTIOBUFEN"=92, "REG_WAKEUP_TESTIOCLAMP"=93, "CORE_RESET_ADDRESS"=94, "CHIP_RESET_ADDRESS"=95, "REG_RF_TXGENCTRL"=96, "REG_RF_TXIFCTRL"=97, "REG_RF_TXRF_SEL_CTRL"=98, "REG_RF_TXRFPWRDEFAULTSET"=99, "REG_RF_RSSITRIM"=100, "REG_RF_TXIFOSCTUNE"=101, "REG_RF_TXIFGAINIMB"=102, "REG_RF_TXIFLOCK"=103, "REG_RF_RXRFLNAGAINTRIM"=104, "REG_RF_RXBIASTR"=105, "REG_RF_RXGENCTRL"=106, "REG_RF_RXIFADCDECLEV"=107, "REG_RF_RXIFDETFILTERTUNE"=108, "REG_RF_RXIFFILTERTUNE"=109, "REG_RF_GENENABLES"=110, "REG_RF_SYNTH_CHANNEL"=111, "REG_TX_RAMP_RTRIM"=112, "REG_TX_RAMP_CTRIM"=113, "REG_RF_XO_TRIM"=114, "REG_RF_SYNTH_SET_TRIM"=115, "REG_RF_ADCCTRL"=116, "REG_RF_ADCOUTPUT"=117, "REG_RF_TXIFAMP"=118, "REG_RF_SYNTH_RTRIM"=119, "REG_RF_SYNTH_CTRIM"=120, "REG_RF_SYNTH_CT"=121, "REG_RF_TXMIXER_IOSTRIM_HIGH_IP"=122, "REG_RF_TXMIXER_IOSTRIM_HIGH_IN"=123, "REG_RF_TXMIXER_IOSTRIM_HIGH_QP"=124, "REG_RF_TXMIXER_IOSTRIM_HIGH_QN"=125, "REG_HX_WUADDR"=126, "REG_REVISION"=127, "REG_NOREG_TEST"=128, "REG_DTEST_RXBUFF"=129, "REG_RXBUFF_NEXT_BLOCK"=130, "REG_RXBUFF_FIRST_IN_PACK"=131, "REG_RXBUFF_FIRST_EMPTY"=132, "REG_MAC_BYPASS"=133, "REG_DTEST_TXBUFF"=134, "REG_TXBUFF_NEXT_BLOCK"=135, "REG_TXBUFF_FIRST_IN_PACK"=136, "REG_TXBUFF_FIRST_EMPTY"=137, "REG_DTEST_SEQ"=138, "REG_DTEST_CKCORR"=139, "REG_MAC_TOPSTATE"=140, "REG_DTEST_INTERFACE"=141, "REG_IFACE_TXRX_BYPASS"=142, "REG_MAC_TXRXWAIT"=143, "REG_MAC_TXRFRAMP"=144, "REG_MAC_TRAINWORD"=145, "REG_MAC_TRAINWORD2"=146, "REG_MAC_SETTINGS"=147, "REG_MAC_CALSELECT1"=148, "REG_MAC_CALSELECT2"=149, "REG_MAC_ANTMATCHSEL"=150, "REG_MAC_ANTTUNESEL1"=151, "REG_MAC_ANTTUNESEL2"=152, "REG_MAC_ANTTUNESEL3"=153, "REG_MAC_ANTTUNESTEP"=154, "REG_MAC_WUMODEBURST"=156, "REG_MAC_WUOFFSHORT"=157, "REG_MAC_WUOFFLONG"=158, "REG_MAC_CLKRECCTRL"=159, "REG_HK_MODE_P2"=162, "REG_MAC_ANTTUNERES1"=164, "REG_MAC_ANTTUNERES2"=165, "REG_INTERFACE_MODE_TEST"=171, "REG_TXRXBUFF_BOTH_P2"=172, "REG_TXRXBUFF_P2"=173, "REG_IRQ_RAWSTATUS1_P2"=174, "REG_MAC_TXIFSTATUS1"=176, "REG_MAC_TXIFSTATUS2"=177, "REG_IRQ_RAWSTATUS2_P2"=178, "REG_MAC_TXIFRAMPDELAY"=179, "REG_MAC_TXIFRAMPSLOPE"=180, "REG_MAX_TXIFRAMP"=181, "REG_IRQ_STATUS1_P2"=182, "REG_IRQ_STATUS2_P2"=183, "REG_IRQ_AUXSTATUS_P2"=184, "REG_MAC_UNLOCK"=188, "REG_MAC_TXIFFREQ"=190, "REG_WAKEUP_TESTCTRL1"=192, "REG_WAKEUP_RX_EN_CNT"=193, "REG_WAKEUP_TESTENABLES"=194, "REG_WAKEUP_DTBI_CTRL"=195, "REG_WAKEUP_DTBO_CTRL"=196, "REG_WAKEUP_TESTIOBUFTEST"=197, "REG_WAKEUP_WK_RX_TESTCTRL1"=198, "REG_WAKEUP_WK_RX_TESTCTRL2"=199, "REG_WAKEUP_SENS_SEQUENCE_CTRL"=200, "REG_WAKEUP_LNABIAS"=201, "REG_WAKEUP_DET_TH_TRIM1"=202, "REG_WAKEUP_LNABIAS_NOM1"=203, "REG_WAKEUP_RX_TSHORT_TRIM1"=204, "REG_WAKEUP_LNABIAS_NOM2"=205, "REG_WAKEUP_RX_TLONG_TRIM1"=206, "REG_WAKEUP_LNA_NEGRTRIM_NOM1"=207, "REG_WAKEUP_RX_TBURST_TRIM1"=208, "REG_WAKEUP_RX_LNA_NEGRTRIM_NOM2"=209, "REG_WAKEUP_RX_BB_G_BW_SEL1"=210, "REG_WAKEUP_WK_RX_DET_IOSTRIM1"=212, "REG_WAKEUP_WK_RX_CTRL2"=214, "REG_WAKEUP_WK_RX_RSSIVOSTRIM"=215, "REG_WAKEUP_LNANEGR_EFF"=216, "REG_WAKEUP_XOSU_FAST"=217, "REG_WAKEUP_STROSCPWIDTH1"=218, "REG_WAKEUP_STROSCPERIOD1"=220, "REG_WAKEUP_STROSCPERIOD2"=221, "REG_WAKEUP_WK_RX_LNA_NEGRTRIM1"=222, "REG_RF_TXTESTENABLE"=224, "REG_RF_TXIFTESTMODE"=225, "REG_RF_RXTESTENABLE"=226, "REG_RF_RXIFTESTCTRL1"=227, "REG_RF_RXIFTESTCTRL2"=228, "REG_RF_RXIFTESTCTRL3"=229, "REG_RF_SYNTH_TESTCTRL1"=230, "REG_RF_SYNTH_TESTCTRL2"=231, "REG_RF_SYNTH_TESTCTRL3"=232, "REG_RF_ADCTEST1"=237, "REG_RF_ADCTEST2"=238, "REG_RF_TXMIXER_IOSTRIM_LOW_IP"=240, "REG_RF_TXMIXER_IOSTRIM_LOW_IN"=241, "REG_RF_TXMIXER_ISOTRIM_LOW_QP"=242, "REG_RF_TXMIXER_IOSTRIM_LOW_QN"=243, "REG_RF_SYNTH_KPD"=244, "REG_RF_SYNTH_LOLEV"=245, "REG_RF_TXRFPWRTUNEANTSET"=246, "REG_RF_TXPD_GAIN_CTRL"=247, "REG_RF_SYNTH_STARTUP"=248, "REG_RF_TXRFANTTUNE_TXMODE"=249, "REG_RF_TXRFANTTUNE_RXMODE"=250, "REG_RF_RXRFANTTUNE_TXMODE"=251, "REG_RF_RXRFANTTUNE_RXMODE"=252, "REG_ANTMATCH1"=253, "REG_ANTMATCH2"=254, "REG_REVISION_P2"=255] ("Register")
                  n99 = call "JTAG SPI.vi"("Mask"=u8 9 ("Data"), "Value"=u8 0 ("Data"), "error in (no error)"=w430, "Target"=w426, "Function"=w425, "Address"=w428) -> ("error out"=w429:errorcluster)  [unwired: 2 in, 3 out]
                }
              }
            }
          }
          n100 = case shown="True" "Loopback Detector" {
            tunnel: w400 -> [w431 w432]
            tunnel: [w431 w439] -> w404
            frame False {
            }
            frame True {
              w434 = u16 2 items=["Power ASIC", "Stim ASIC", "MICS Radio", "FRAM"] ("Target")
              w435 = u16 3 items=["Power UP", "Power DN", "Write Single", "Read Single", "Write Block", "Read Block", "Write Masked", "Test Value"] ("Function")
              w437 = u16 85 items=["---MANUAL ENTRY---"=1000, "REG_NOREG"=0, "REG_RXBUFF_USED"=1, "REG_RXBUFF_BSIZE"=2, "REG_TXBUFF_USED"=3, "REG_TXBUFF_BSIZE"=4, "REG_TXBUFF_MAXPACKSIZE"=5, "REG_MAC_ERRCLR"=6, "REG_MAC_TRAINNUM"=7, "REG_MAC_SYNCMATCH"=8, "REG_MAC_SYNC1"=9, "REG_MAC_SYNC2"=10, "REG_MAC_SYNC3"=11, "REG_MAC_SYNC4"=12, "REG_MAC_SYNC5"=13, "REG_MAC_MAXBERR"=14, "REG_MAC_ECCORR"=15, "REG_MAC_CRCERR"=16, "REG_MAC_BLKCNT1"=17, "REG_MAC_BLKCNT2"=18, "REG_MAC_IMDTRANSID1"=19, "REG_MAC_IMDTRANSID2"=20, "REG_MAC_IMDTRANSID3"=21, "REG_MAC_COMPANYID"=22, "REG_MAC_MODUSER"=23, "REG_MAC_CHANNEL"=25, "REG_MAC_CLEARWDOG"=26, "REG_MAC_CKCORRTHRESH"=27, "REG_HK_TXADDR"=28, "REG_HK_TXDATA"=29, "REG_HK_TXREPLY"=30, "REG_HK_USERDATA"=31, "REG_HK_USERSTATUS"=32, "REG_HK_LASTADDRESS"=33, "REG_HK_MODE"=34, "REG_MAC_STATUSSEQ"=35, "REG_MAC_MAXRETRIES"=36, "REG_MAC_RESENDTIME"=37, "REG_MAC_POWERSAVETIME"=38, "REG_MAC_HEAD_DET"=39, "REG_MAC_CTRL"=41, "REG_MAC_INITCOM"=42, "REG_INTERFACE_MODE"=43, "REG_TXRXBUFF_BOTH"=44, "REG_TXRXBUFF"=45, "REG_IRQ_RAWSTATUS1"=46, "REG_IRQ_ENABLE1"=47, "REG_IRQ_ENABLESET1"=48, "REG_IRQ_ENABLECLEAR1"=49, "REG_IRQ_RAWSTATUS2"=50, "REG_IRQ_ENABLE2"=51, "REG_IRQ_ENABLESET2"=52, "REG_IRQ_ENABLECLEAR2"=53, "REG_IRQ_STATUS1"=54, "REG_IRQ_STATUS2"=55, "REG_IRQ_AUXSTATUS"=56, "REG_TXBUFF_OVERFLOW"=57, "REG_PO0"=58, "REG_P01"=59, "REG_P02"=60, "REG_P03"=61, "REG_GP0"=62, "REG_GPI"=63, "REG_WAKEUP_245IN"=64, "REG_WAKEUP_COMPANYID"=65, "REG_WAKEUP_IMDTRANSID1"=66, "REG_WAKEUP_IMDTRANSID2"=67, "REG_WAKEUP_IMDTRANSID3"=68, "REG_WAKEUP_CHANNEL"=69, "REG_WAKEUP_MODUSER"=70, "REG_WAKEUP_DEVICEMODE"=71, "REG_WAKEUP_WK_RX_CTRL1"=72, "REG_WAKEUP_STACK_ADDR"=73, "REG_WAKEUP_CTRL"=74, "REG_WAKEUP_STROSCRTRIM"=75, "REG_WAKEUP_BIASTRIM"=76, "REG_WAKEUP_ANT245TUNE"=77, "REG_WAKEUP_WK_RX_RTRIMDET"=78, "REG_WAKEUP_WK_RX_RTRIMDEMOD"=79, "REG_WAKEUP_WK_RX_RSSIGAIN"=80, "REG_WAKEUP_LNAFREQ1"=81, "REG_WAKEUP_STACK"=83, "REG_WAKUP_XOSU"=84, "REG_WAKUP_CNTDROPOUT"=85, "REG_WAKEUP_CRCCTRL"=86, "REG_WAKEUP_CRCWORD1"=87, "REG_WAKEUP_CRCWORD2"=88, "REG_WAKEUP_WK_RX_CTRIM"=89, "REG_WAKEUP_VDDATRIM"=90, "REG_WAKEUP_VDDDTRIM"=91, "REG_WAKEUP_TESTIOBUFEN"=92, "REG_WAKEUP_TESTIOCLAMP"=93, "CORE_RESET_ADDRESS"=94, "CHIP_RESET_ADDRESS"=95, "REG_RF_TXGENCTRL"=96, "REG_RF_TXIFCTRL"=97, "REG_RF_TXRF_SEL_CTRL"=98, "REG_RF_TXRFPWRDEFAULTSET"=99, "REG_RF_RSSITRIM"=100, "REG_RF_TXIFOSCTUNE"=101, "REG_RF_TXIFGAINIMB"=102, "REG_RF_TXIFLOCK"=103, "REG_RF_RXRFLNAGAINTRIM"=104, "REG_RF_RXBIASTR"=105, "REG_RF_RXGENCTRL"=106, "REG_RF_RXIFADCDECLEV"=107, "REG_RF_RXIFDETFILTERTUNE"=108, "REG_RF_RXIFFILTERTUNE"=109, "REG_RF_GENENABLES"=110, "REG_RF_SYNTH_CHANNEL"=111, "REG_TX_RAMP_RTRIM"=112, "REG_TX_RAMP_CTRIM"=113, "REG_RF_XO_TRIM"=114, "REG_RF_SYNTH_SET_TRIM"=115, "REG_RF_ADCCTRL"=116, "REG_RF_ADCOUTPUT"=117, "REG_RF_TXIFAMP"=118, "REG_RF_SYNTH_RTRIM"=119, "REG_RF_SYNTH_CTRIM"=120, "REG_RF_SYNTH_CT"=121, "REG_RF_TXMIXER_IOSTRIM_HIGH_IP"=122, "REG_RF_TXMIXER_IOSTRIM_HIGH_IN"=123, "REG_RF_TXMIXER_IOSTRIM_HIGH_QP"=124, "REG_RF_TXMIXER_IOSTRIM_HIGH_QN"=125, "REG_HX_WUADDR"=126, "REG_REVISION"=127, "REG_NOREG_TEST"=128, "REG_DTEST_RXBUFF"=129, "REG_RXBUFF_NEXT_BLOCK"=130, "REG_RXBUFF_FIRST_IN_PACK"=131, "REG_RXBUFF_FIRST_EMPTY"=132, "REG_MAC_BYPASS"=133, "REG_DTEST_TXBUFF"=134, "REG_TXBUFF_NEXT_BLOCK"=135, "REG_TXBUFF_FIRST_IN_PACK"=136, "REG_TXBUFF_FIRST_EMPTY"=137, "REG_DTEST_SEQ"=138, "REG_DTEST_CKCORR"=139, "REG_MAC_TOPSTATE"=140, "REG_DTEST_INTERFACE"=141, "REG_IFACE_TXRX_BYPASS"=142, "REG_MAC_TXRXWAIT"=143, "REG_MAC_TXRFRAMP"=144, "REG_MAC_TRAINWORD"=145, "REG_MAC_TRAINWORD2"=146, "REG_MAC_SETTINGS"=147, "REG_MAC_CALSELECT1"=148, "REG_MAC_CALSELECT2"=149, "REG_MAC_ANTMATCHSEL"=150, "REG_MAC_ANTTUNESEL1"=151, "REG_MAC_ANTTUNESEL2"=152, "REG_MAC_ANTTUNESEL3"=153, "REG_MAC_ANTTUNESTEP"=154, "REG_MAC_WUMODEBURST"=156, "REG_MAC_WUOFFSHORT"=157, "REG_MAC_WUOFFLONG"=158, "REG_MAC_CLKRECCTRL"=159, "REG_HK_MODE_P2"=162, "REG_MAC_ANTTUNERES1"=164, "REG_MAC_ANTTUNERES2"=165, "REG_INTERFACE_MODE_TEST"=171, "REG_TXRXBUFF_BOTH_P2"=172, "REG_TXRXBUFF_P2"=173, "REG_IRQ_RAWSTATUS1_P2"=174, "REG_MAC_TXIFSTATUS1"=176, "REG_MAC_TXIFSTATUS2"=177, "REG_IRQ_RAWSTATUS2_P2"=178, "REG_MAC_TXIFRAMPDELAY"=179, "REG_MAC_TXIFRAMPSLOPE"=180, "REG_MAX_TXIFRAMP"=181, "REG_IRQ_STATUS1_P2"=182, "REG_IRQ_STATUS2_P2"=183, "REG_IRQ_AUXSTATUS_P2"=184, "REG_MAC_UNLOCK"=188, "REG_MAC_TXIFFREQ"=190, "REG_WAKEUP_TESTCTRL1"=192, "REG_WAKEUP_RX_EN_CNT"=193, "REG_WAKEUP_TESTENABLES"=194, "REG_WAKEUP_DTBI_CTRL"=195, "REG_WAKEUP_DTBO_CTRL"=196, "REG_WAKEUP_TESTIOBUFTEST"=197, "REG_WAKEUP_WK_RX_TESTCTRL1"=198, "REG_WAKEUP_WK_RX_TESTCTRL2"=199, "REG_WAKEUP_SENS_SEQUENCE_CTRL"=200, "REG_WAKEUP_LNABIAS"=201, "REG_WAKEUP_DET_TH_TRIM1"=202, "REG_WAKEUP_LNABIAS_NOM1"=203, "REG_WAKEUP_RX_TSHORT_TRIM1"=204, "REG_WAKEUP_LNABIAS_NOM2"=205, "REG_WAKEUP_RX_TLONG_TRIM1"=206, "REG_WAKEUP_LNA_NEGRTRIM_NOM1"=207, "REG_WAKEUP_RX_TBURST_TRIM1"=208, "REG_WAKEUP_RX_LNA_NEGRTRIM_NOM2"=209, "REG_WAKEUP_RX_BB_G_BW_SEL1"=210, "REG_WAKEUP_WK_RX_DET_IOSTRIM1"=212, "REG_WAKEUP_WK_RX_CTRL2"=214, "REG_WAKEUP_WK_RX_RSSIVOSTRIM"=215, "REG_WAKEUP_LNANEGR_EFF"=216, "REG_WAKEUP_XOSU_FAST"=217, "REG_WAKEUP_STROSCPWIDTH1"=218, "REG_WAKEUP_STROSCPERIOD1"=220, "REG_WAKEUP_STROSCPERIOD2"=221, "REG_WAKEUP_WK_RX_LNA_NEGRTRIM1"=222, "REG_RF_TXTESTENABLE"=224, "REG_RF_TXIFTESTMODE"=225, "REG_RF_RXTESTENABLE"=226, "REG_RF_RXIFTESTCTRL1"=227, "REG_RF_RXIFTESTCTRL2"=228, "REG_RF_RXIFTESTCTRL3"=229, "REG_RF_SYNTH_TESTCTRL1"=230, "REG_RF_SYNTH_TESTCTRL2"=231, "REG_RF_SYNTH_TESTCTRL3"=232, "REG_RF_ADCTEST1"=237, "REG_RF_ADCTEST2"=238, "REG_RF_TXMIXER_IOSTRIM_LOW_IP"=240, "REG_RF_TXMIXER_IOSTRIM_LOW_IN"=241, "REG_RF_TXMIXER_ISOTRIM_LOW_QP"=242, "REG_RF_TXMIXER_IOSTRIM_LOW_QN"=243, "REG_RF_SYNTH_KPD"=244, "REG_RF_SYNTH_LOLEV"=245, "REG_RF_TXRFPWRTUNEANTSET"=246, "REG_RF_TXPD_GAIN_CTRL"=247, "REG_RF_SYNTH_STARTUP"=248, "REG_RF_TXRFANTTUNE_TXMODE"=249, "REG_RF_TXRFANTTUNE_RXMODE"=250, "REG_RF_RXRFANTTUNE_TXMODE"=251, "REG_RF_RXRFANTTUNE_RXMODE"=252, "REG_ANTMATCH1"=253, "REG_ANTMATCH2"=254, "REG_REVISION_P2"=255] ("Register")
              w438 = u16 64 items=["---MANUAL ENTRY---"=1000, "REG_NOREG"=0, "REG_RXBUFF_USED"=1, "REG_RXBUFF_BSIZE"=2, "REG_TXBUFF_USED"=3, "REG_TXBUFF_BSIZE"=4, "REG_TXBUFF_MAXPACKSIZE"=5, "REG_MAC_ERRCLR"=6, "REG_MAC_TRAINNUM"=7, "REG_MAC_SYNCMATCH"=8, "REG_MAC_SYNC1"=9, "REG_MAC_SYNC2"=10, "REG_MAC_SYNC3"=11, "REG_MAC_SYNC4"=12, "REG_MAC_SYNC5"=13, "REG_MAC_MAXBERR"=14, "REG_MAC_ECCORR"=15, "REG_MAC_CRCERR"=16, "REG_MAC_BLKCNT1"=17, "REG_MAC_BLKCNT2"=18, "REG_MAC_IMDTRANSID1"=19, "REG_MAC_IMDTRANSID2"=20, "REG_MAC_IMDTRANSID3"=21, "REG_MAC_COMPANYID"=22, "REG_MAC_MODUSER"=23, "REG_MAC_CHANNEL"=25, "REG_MAC_CLEARWDOG"=26, "REG_MAC_CKCORRTHRESH"=27, "REG_HK_TXADDR"=28, "REG_HK_TXDATA"=29, "REG_HK_TXREPLY"=30, "REG_HK_USERDATA"=31, "REG_HK_USERSTATUS"=32, "REG_HK_LASTADDRESS"=33, "REG_HK_MODE"=34, "REG_MAC_STATUSSEQ"=35, "REG_MAC_MAXRETRIES"=36, "REG_MAC_RESENDTIME"=37, "REG_MAC_POWERSAVETIME"=38, "REG_MAC_HEAD_DET"=39, "REG_MAC_CTRL"=41, "REG_MAC_INITCOM"=42, "REG_INTERFACE_MODE"=43, "REG_TXRXBUFF_BOTH"=44, "REG_TXRXBUFF"=45, "REG_IRQ_RAWSTATUS1"=46, "REG_IRQ_ENABLE1"=47, "REG_IRQ_ENABLESET1"=48, "REG_IRQ_ENABLECLEAR1"=49, "REG_IRQ_RAWSTATUS2"=50, "REG_IRQ_ENABLE2"=51, "REG_IRQ_ENABLESET2"=52, "REG_IRQ_ENABLECLEAR2"=53, "REG_IRQ_STATUS1"=54, "REG_IRQ_STATUS2"=55, "REG_IRQ_AUXSTATUS"=56, "REG_TXBUFF_OVERFLOW"=57, "REG_PO0"=58, "REG_P01"=59, "REG_P02"=60, "REG_P03"=61, "REG_GP0"=62, "REG_GPI"=63, "REG_WAKEUP_245IN"=64, "REG_WAKEUP_COMPANYID"=65, "REG_WAKEUP_IMDTRANSID1"=66, "REG_WAKEUP_IMDTRANSID2"=67, "REG_WAKEUP_IMDTRANSID3"=68, "REG_WAKEUP_CHANNEL"=69, "REG_WAKEUP_MODUSER"=70, "REG_WAKEUP_DEVICEMODE"=71, "REG_WAKEUP_WK_RX_CTRL1"=72, "REG_WAKEUP_STACK_ADDR"=73, "REG_WAKEUP_CTRL"=74, "REG_WAKEUP_STROSCRTRIM"=75, "REG_WAKEUP_BIASTRIM"=76, "REG_WAKEUP_ANT245TUNE"=77, "REG_WAKEUP_WK_RX_RTRIMDET"=78, "REG_WAKEUP_WK_RX_RTRIMDEMOD"=79, "REG_WAKEUP_WK_RX_RSSIGAIN"=80, "REG_WAKEUP_LNAFREQ1"=81, "REG_WAKEUP_STACK"=83, "REG_WAKUP_XOSU"=84, "REG_WAKUP_CNTDROPOUT"=85, "REG_WAKEUP_CRCCTRL"=86, "REG_WAKEUP_CRCWORD1"=87, "REG_WAKEUP_CRCWORD2"=88, "REG_WAKEUP_WK_RX_CTRIM"=89, "REG_WAKEUP_VDDATRIM"=90, "REG_WAKEUP_VDDDTRIM"=91, "REG_WAKEUP_TESTIOBUFEN"=92, "REG_WAKEUP_TESTIOCLAMP"=93, "CORE_RESET_ADDRESS"=94, "CHIP_RESET_ADDRESS"=95, "REG_RF_TXGENCTRL"=96, "REG_RF_TXIFCTRL"=97, "REG_RF_TXRF_SEL_CTRL"=98, "REG_RF_TXRFPWRDEFAULTSET"=99, "REG_RF_RSSITRIM"=100, "REG_RF_TXIFOSCTUNE"=101, "REG_RF_TXIFGAINIMB"=102, "REG_RF_TXIFLOCK"=103, "REG_RF_RXRFLNAGAINTRIM"=104, "REG_RF_RXBIASTR"=105, "REG_RF_RXGENCTRL"=106, "REG_RF_RXIFADCDECLEV"=107, "REG_RF_RXIFDETFILTERTUNE"=108, "REG_RF_RXIFFILTERTUNE"=109, "REG_RF_GENENABLES"=110, "REG_RF_SYNTH_CHANNEL"=111, "REG_TX_RAMP_RTRIM"=112, "REG_TX_RAMP_CTRIM"=113, "REG_RF_XO_TRIM"=114, "REG_RF_SYNTH_SET_TRIM"=115, "REG_RF_ADCCTRL"=116, "REG_RF_ADCOUTPUT"=117, "REG_RF_TXIFAMP"=118, "REG_RF_SYNTH_RTRIM"=119, "REG_RF_SYNTH_CTRIM"=120, "REG_RF_SYNTH_CT"=121, "REG_RF_TXMIXER_IOSTRIM_HIGH_IP"=122, "REG_RF_TXMIXER_IOSTRIM_HIGH_IN"=123, "REG_RF_TXMIXER_IOSTRIM_HIGH_QP"=124, "REG_RF_TXMIXER_IOSTRIM_HIGH_QN"=125, "REG_HX_WUADDR"=126, "REG_REVISION"=127, "REG_NOREG_TEST"=128, "REG_DTEST_RXBUFF"=129, "REG_RXBUFF_NEXT_BLOCK"=130, "REG_RXBUFF_FIRST_IN_PACK"=131, "REG_RXBUFF_FIRST_EMPTY"=132, "REG_MAC_BYPASS"=133, "REG_DTEST_TXBUFF"=134, "REG_TXBUFF_NEXT_BLOCK"=135, "REG_TXBUFF_FIRST_IN_PACK"=136, "REG_TXBUFF_FIRST_EMPTY"=137, "REG_DTEST_SEQ"=138, "REG_DTEST_CKCORR"=139, "REG_MAC_TOPSTATE"=140, "REG_DTEST_INTERFACE"=141, "REG_IFACE_TXRX_BYPASS"=142, "REG_MAC_TXRXWAIT"=143, "REG_MAC_TXRFRAMP"=144, "REG_MAC_TRAINWORD"=145, "REG_MAC_TRAINWORD2"=146, "REG_MAC_SETTINGS"=147, "REG_MAC_CALSELECT1"=148, "REG_MAC_CALSELECT2"=149, "REG_MAC_ANTMATCHSEL"=150, "REG_MAC_ANTTUNESEL1"=151, "REG_MAC_ANTTUNESEL2"=152, "REG_MAC_ANTTUNESEL3"=153, "REG_MAC_ANTTUNESTEP"=154, "REG_MAC_WUMODEBURST"=156, "REG_MAC_WUOFFSHORT"=157, "REG_MAC_WUOFFLONG"=158, "REG_MAC_CLKRECCTRL"=159, "REG_HK_MODE_P2"=162, "REG_MAC_ANTTUNERES1"=164, "REG_MAC_ANTTUNERES2"=165, "REG_INTERFACE_MODE_TEST"=171, "REG_TXRXBUFF_BOTH_P2"=172, "REG_TXRXBUFF_P2"=173, "REG_IRQ_RAWSTATUS1_P2"=174, "REG_MAC_TXIFSTATUS1"=176, "REG_MAC_TXIFSTATUS2"=177, "REG_IRQ_RAWSTATUS2_P2"=178, "REG_MAC_TXIFRAMPDELAY"=179, "REG_MAC_TXIFRAMPSLOPE"=180, "REG_MAX_TXIFRAMP"=181, "REG_IRQ_STATUS1_P2"=182, "REG_IRQ_STATUS2_P2"=183, "REG_IRQ_AUXSTATUS_P2"=184, "REG_MAC_UNLOCK"=188, "REG_MAC_TXIFFREQ"=190, "REG_WAKEUP_TESTCTRL1"=192, "REG_WAKEUP_RX_EN_CNT"=193, "REG_WAKEUP_TESTENABLES"=194, "REG_WAKEUP_DTBI_CTRL"=195, "REG_WAKEUP_DTBO_CTRL"=196, "REG_WAKEUP_TESTIOBUFTEST"=197, "REG_WAKEUP_WK_RX_TESTCTRL1"=198, "REG_WAKEUP_WK_RX_TESTCTRL2"=199, "REG_WAKEUP_SENS_SEQUENCE_CTRL"=200, "REG_WAKEUP_LNABIAS"=201, "REG_WAKEUP_DET_TH_TRIM1"=202, "REG_WAKEUP_LNABIAS_NOM1"=203, "REG_WAKEUP_RX_TSHORT_TRIM1"=204, "REG_WAKEUP_LNABIAS_NOM2"=205, "REG_WAKEUP_RX_TLONG_TRIM1"=206, "REG_WAKEUP_LNA_NEGRTRIM_NOM1"=207, "REG_WAKEUP_RX_TBURST_TRIM1"=208, "REG_WAKEUP_RX_LNA_NEGRTRIM_NOM2"=209, "REG_WAKEUP_RX_BB_G_BW_SEL1"=210, "REG_WAKEUP_WK_RX_DET_IOSTRIM1"=212, "REG_WAKEUP_WK_RX_CTRL2"=214, "REG_WAKEUP_WK_RX_RSSIVOSTRIM"=215, "REG_WAKEUP_LNANEGR_EFF"=216, "REG_WAKEUP_XOSU_FAST"=217, "REG_WAKEUP_STROSCPWIDTH1"=218, "REG_WAKEUP_STROSCPERIOD1"=220, "REG_WAKEUP_STROSCPERIOD2"=221, "REG_WAKEUP_WK_RX_LNA_NEGRTRIM1"=222, "REG_RF_TXTESTENABLE"=224, "REG_RF_TXIFTESTMODE"=225, "REG_RF_RXTESTENABLE"=226, "REG_RF_RXIFTESTCTRL1"=227, "REG_RF_RXIFTESTCTRL2"=228, "REG_RF_RXIFTESTCTRL3"=229, "REG_RF_SYNTH_TESTCTRL1"=230, "REG_RF_SYNTH_TESTCTRL2"=231, "REG_RF_SYNTH_TESTCTRL3"=232, "REG_RF_ADCTEST1"=237, "REG_RF_ADCTEST2"=238, "REG_RF_TXMIXER_IOSTRIM_LOW_IP"=240, "REG_RF_TXMIXER_IOSTRIM_LOW_IN"=241, "REG_RF_TXMIXER_ISOTRIM_LOW_QP"=242, "REG_RF_TXMIXER_IOSTRIM_LOW_QN"=243, "REG_RF_SYNTH_KPD"=244, "REG_RF_SYNTH_LOLEV"=245, "REG_RF_TXRFPWRTUNEANTSET"=246, "REG_RF_TXPD_GAIN_CTRL"=247, "REG_RF_SYNTH_STARTUP"=248, "REG_RF_TXRFANTTUNE_TXMODE"=249, "REG_RF_TXRFANTTUNE_RXMODE"=250, "REG_RF_RXRFANTTUNE_TXMODE"=251, "REG_RF_RXRFANTTUNE_RXMODE"=252, "REG_ANTMATCH1"=253, "REG_ANTMATCH2"=254, "REG_REVISION_P2"=255] ("Register")
              n101 = call "JTAG SPI.vi"("error in (no error)"=w432, "Target"=w434, "Function"=w435, "Address"=w438) -> ("error out"=w440:errorcluster, "Read Value"=→"Loopback Data":u8)  [unwired: 4 in, 2 out]
              n102 = call "JTAG SPI.vi"("error in (no error)"=w440, "Target"=w434, "Function"=w435, "Address"=w437) -> ("error out"=w439:errorcluster, "Read Value"=→"Retries":u8)  [unwired: 4 in, 2 out]
            }
          }
        }
      }
    }
    n103 = Unbundle By Name(w90) -> ("status"=w87:bool)
    n104 = Or(x=w87, y="Done") -> (x .or. y?=w89:bool)
  }
  n105 = call "JTAG SPI.vi"("Mask"=u8 64 ("Data"), "Value"=u8 0 ("Data"), "error in (no error)"=w33, "Target"=w28, "Function"=w29, "Address"=w32) -> ("error out"=→"error out":errorcluster)  [unwired: 2 in, 3 out]
